vi "Beampointing_ajgEdit.vi"() -> ()   [LabVIEW 2020]
uses:
  Ctrs/beam detection.ctl
  GUI_Beampointing_single_TRA/Ctrs/move.ctl
  Shared/GUI_Template/GUI_master/tcp_new_data_event.ctl
  Shared/GUI_Template/GUI_master/tcp new data cluster.ctl
  Shared/MySQL/Preset Query Enum.ctl
  Ctrs/motor cfg.ctl
  Ctrs/BP configuration.ctl
  General GUIs/Device GUIs/GUI_Cameras/Controls/Crosshair type def.ctl
  <userlib>/_OpenG.lib/array/array.llb/Filter 1D Array with Scalar (String)__ogtk.vi
  <vilib>/Utility/file.llb/Read From Spreadsheet File (string).vi
  <userlib>/_OpenG.lib/array/array.llb/Index 1D Array Elements (String)__ogtk.vi
  <vilib>/Analysis/NI_AALBase.lvlib
  <vilib>/vision/NI_Vision_Development_Module.lvlib
  <vilib>/Utility/file.llb/Write To Spreadsheet File (string).vi
panel:
  in  "Position.Axis 3::99":dbl=77.0 caption="Motor Axis 1" min=0.0 max=20.0 format="%#_6f"
  out "tcp data event 2":T1
  out "error out 3":errorcluster
  out "Array 3":sgl[](array[numeric])
  in  "GUIdevice 97":string="BELLA_ESP_2"
  in  "GUIdevice 98":string="BellaESP"
  in  "Position.Axis 1::97":dbl=77.0 caption="Motor Axis 1" min=-10.0 max=10.0 format="%#_6f"
  in  "Position.Axis 2::97":dbl=77.0 caption="Motor Axis 1" min=-12.0 max=10.0 format="%#_6f"
  in  "Position.Axis 3::97":dbl=77.0 caption="Motor Axis 1" min=-12.0 max=12.0 format="%#_6f"
  in  "Position.Axis 1::98":dbl=77.0 caption="Motor Axis 1" min=0.0 max=20.0 format="%#_6f"
  in  "Position.Axis 2::98":dbl=77.0 caption="Motor Axis 1" min=0.0 max=20.0 format="%#_6f"
  in  "Position.Axis 3::98":dbl=77.0 caption="Motor Axis 1" min=0.0 max=20.0 format="%#_6f"
  in  "save path":path=path "W:/BP_DATA"
  out "size(s) 6":i32
  out "config path":string
  out "Moving Y":string
  out "Moving X":string
  out "particles":T2(array[cluster])
  out "millisecond timer value":u32
  out "appended path":path
  in  "active Axis ref 3":cluster{"Ref X":refnum<vi>, "Ref Y":refnum<vi>}
  out "motor refs 3":refnum<vi>[](array[refnum])
  in  "active man refs":cluster{"Ref X":refnum<vi>, "Ref Y":refnum<vi>}
  in  "Numeric":dbl
  out "Current State":string
  out "CCDs":string[](array[string])
  in  "GUIdevice 12":string
  in  "GUIdevice 11":string
  in  "GUIdevice 10":string
  in  "GUIdevice 9":string
  out "error out 2":errorcluster
  in  "active cams":string[](array[string])
  in  "Motor Y":dbl[][](array[numeric])
  in  "Motor X":dbl[][](array[numeric])
  out "Names":string[](array[string])
  in  "Offset X stats":dbl[][](array[numeric])
  in  "Offset Y stats":dbl[][](array[numeric])
  out "Box":T3(array[cluster])
  in  "Tab Cams":enum32{"Config ", "Main", "History"}(tab)=enum."Main"
  in  "associated motors Y":T4 {"Motor CCD 12" items=["F3M5 Horizontal", "F3M5 Vertical", "F3M6 Horizontal", "F3M3 Vertical", "F3M3 Horizontal", "F3M6 Vertical", "M4 X Axis", "M5 X Axis", "M5 Y Axis"]; "Motor CCD 11" items=["F3M5 Horizontal", "F3M5 Vertical", "F3M6 Horizontal", "F3M3 Vertical", "F3M3 Horizontal", "F3M6 Vertical", "M4 X Axis", "M5 X Axis", "M5 Y Axis"]; "Motor CCD 10" items=["F3M5 Horizontal", "F3M5 Vertical", "F3M6 Horizontal", "F3M3 Vertical", "F3M3 Horizontal", "F3M6 Vertical", "M4 X Axis", "M5 X Axis", "M5 Y Axis"]; "Motor CCD 9" items=["F3M5 Horizontal", "F3M5 Vertical", "F3M6 Horizontal", "F3M3 Vertical", "F3M3 Horizontal", "F3M6 Vertical", "M4 X Axis", "M5 X Axis", "M5 Y Axis"]; "Motor CCD 8" items=["F3M5 Horizontal", "F3M5 Vertical", "F3M6 Horizontal", "F3M3 Vertical", "F3M3 Horizontal", "F3M6 Vertical", "M4 X Axis", "M5 X Axis", "M5 Y Axis"]; "Motor CCD 7" items=["F3M5 Horizontal", "F3M5 Vertical", "F3M6 Horizontal", "F3M3 Vertical", "F3M3 Horizontal", "F3M6 Vertical", "M4 X Axis", "M5 X Axis", "M5 Y Axis"]; "Motor CCD 6" items=["F3M5 Horizontal", "F3M5 Vertical", "F3M6 Horizontal", "F3M3 Vertical", "F3M3 Horizontal", "F3M6 Vertical", "M4 X Axis", "M5 X Axis", "M5 Y Axis"]; "Motor CCD 5" items=["F3M5 Horizontal", "F3M5 Vertical", "F3M6 Horizontal", "F3M3 Vertical", "F3M3 Horizontal", "F3M6 Vertical", "M4 X Axis", "M5 X Axis", "M5 Y Axis"]; "Motor CCD 4" items=["F3M5 Horizontal", "F3M5 Vertical", "F3M6 Horizontal", "F3M3 Vertical", "F3M3 Horizontal", "F3M6 Vertical", "M4 X Axis", "M5 X Axis", "M5 Y Axis"]; "Motor CCD 3" items=["F3M5 Horizontal", "F3M5 Vertical", "F3M6 Horizontal", "F3M3 Vertical", "F3M3 Horizontal", "F3M6 Vertical", "M4 X Axis", "M5 X Axis", "M5 Y Axis"]; "Motor CCD 2" items=["F3M5 Horizontal", "F3M5 Vertical", "F3M6 Horizontal", "F3M3 Vertical", "F3M3 Horizontal", "F3M6 Vertical", "M4 X Axis", "M5 X Axis", "M5 Y Axis"]; "Motor CCD 1" items=["F3M5 Horizontal", "F3M5 Vertical", "F3M6 Horizontal", "F3M3 Vertical", "F3M3 Horizontal", "F3M6 Vertical", "M4 X Axis", "M5 X Axis", "M5 Y Axis"]}
  in  "associated motors X":T4 {"Motor CCD 12" items=["F3M5 Horizontal", "F3M5 Vertical", "F3M6 Horizontal", "F3M3 Vertical", "F3M3 Horizontal", "F3M6 Vertical", "M4 X Axis", "M5 X Axis", "M5 Y Axis"]; "Motor CCD 11" items=["F3M5 Horizontal", "F3M5 Vertical", "F3M6 Horizontal", "F3M3 Vertical", "F3M3 Horizontal", "F3M6 Vertical", "M4 X Axis", "M5 X Axis", "M5 Y Axis"]; "Motor CCD 10" items=["F3M5 Horizontal", "F3M5 Vertical", "F3M6 Horizontal", "F3M3 Vertical", "F3M3 Horizontal", "F3M6 Vertical", "M4 X Axis", "M5 X Axis", "M5 Y Axis"]; "Motor CCD 9" items=["F3M5 Horizontal", "F3M5 Vertical", "F3M6 Horizontal", "F3M3 Vertical", "F3M3 Horizontal", "F3M6 Vertical", "M4 X Axis", "M5 X Axis", "M5 Y Axis"]; "Motor CCD 8" items=["F3M5 Horizontal", "F3M5 Vertical", "F3M6 Horizontal", "F3M3 Vertical", "F3M3 Horizontal", "F3M6 Vertical", "M4 X Axis", "M5 X Axis", "M5 Y Axis"]; "Motor CCD 7" items=["F3M5 Horizontal", "F3M5 Vertical", "F3M6 Horizontal", "F3M3 Vertical", "F3M3 Horizontal", "F3M6 Vertical", "M4 X Axis", "M5 X Axis", "M5 Y Axis"]; "Motor CCD 6" items=["F3M5 Horizontal", "F3M5 Vertical", "F3M6 Horizontal", "F3M3 Vertical", "F3M3 Horizontal", "F3M6 Vertical", "M4 X Axis", "M5 X Axis", "M5 Y Axis"]; "Motor CCD 5" items=["F3M5 Horizontal", "F3M5 Vertical", "F3M6 Horizontal", "F3M3 Vertical", "F3M3 Horizontal", "F3M6 Vertical", "M4 X Axis", "M5 X Axis", "M5 Y Axis"]; "Motor CCD 4" items=["F3M5 Horizontal", "F3M5 Vertical", "F3M6 Horizontal", "F3M3 Vertical", "F3M3 Horizontal", "F3M6 Vertical", "M4 X Axis", "M5 X Axis", "M5 Y Axis"]; "Motor CCD 3" items=["F3M5 Horizontal", "F3M5 Vertical", "F3M6 Horizontal", "F3M3 Vertical", "F3M3 Horizontal", "F3M6 Vertical", "M4 X Axis", "M5 X Axis", "M5 Y Axis"]; "Motor CCD 2" items=["F3M5 Horizontal", "F3M5 Vertical", "F3M6 Horizontal", "F3M3 Vertical", "F3M3 Horizontal", "F3M6 Vertical", "M4 X Axis", "M5 X Axis", "M5 Y Axis"]; "Motor CCD 1" items=["F3M5 Horizontal", "F3M5 Vertical", "F3M6 Horizontal", "F3M3 Vertical", "F3M3 Horizontal", "F3M6 Vertical", "M4 X Axis", "M5 X Axis", "M5 Y Axis"]}
  out "Cameras":T5
  out "Status":cluster{i32, i32, "Centroid X":dbl[][]}(graph)
  in  "Exposure:12":dbl=0.095 min=0.0001 max=1.0 format="%#_6f"
  in  "Triggerdelay::12":dbl=0.003 min=0.0 max=0.09 format="%#_6f"
  in  "Exposure::11":dbl=0.095 min=0.0001 max=1.0 format="%#_6f"
  in  "Triggerdelay::11":dbl=0.003 min=0.0 max=0.09 format="%#_6f"
  in  "Exposure::10":dbl=0.095 min=0.0001 max=1.0 format="%#_6f"
  in  "Triggerdelay::10":dbl=0.003 min=0.0 max=0.09 format="%#_6f"
  in  "Exposure::9":dbl=0.095 min=0.0001 max=1.0 format="%#_6f"
  in  "Triggerdelay::9":dbl=0.003 min=0.0 max=0.09 format="%#_6f"
  in  "Trigger::9":bool
  in  "Trigger::10":bool caption="Trigger:10"
  in  "Trigger::11":bool
  in  "Trigger::12":bool
  in  "Target.Y::9":dbl=45.0 caption="T9y" min=0.0 max=2000.0 format="%#_6f"
  in  "Target.X::9":dbl=47.0 caption="Tx9" min=0.0 max=2000.0 format="%#_6f"
  in  "Target.Y::10":dbl=45.0 caption="T10y" min=0.0 max=2000.0 format="%#_6f"
  in  "Target.X::10":dbl=47.0 caption="T10x" min=0.0 max=2000.0 format="%#_6f"
  in  "Target.Y::11":dbl=45.0 caption="T11y" min=0.0 max=2000.0 format="%#_6f"
  in  "Target.X::11":dbl=47.0 caption="T11x" min=0.0 max=2000.0 format="%#_6f"
  in  "Target.Y::12":dbl=45.0 caption="T12y" min=0.0 max=2000.0 format="%#_6f"
  in  "Target.X::12":dbl=47.0 caption="T12x" min=0.0 max=2000.0 format="%#_6f"
  in  "Exposure::8":dbl=0.095 min=0.0001 max=1.0 format="%#_6f"
  in  "Triggerdelay::8":dbl=0.003 min=0.0 max=0.09 format="%#_6f"
  in  "Trigger::8":bool
  in  "Target.Y::8":dbl=45.0 caption="T8y" min=0.0 max=2000.0 format="%#_6f"
  in  "Target.X::8":dbl=47.0 caption="T8x" min=0.0 max=2000.0 format="%#_6f"
  in  "Target.Y::7":dbl=45.0 caption="T7x" min=0.0 max=2000.0 format="%#_6f"
  in  "Target.X::7":dbl=47.0 caption="T7y" min=0.0 max=2000.0 format="%#_6f"
  in  "Target.Y::6":dbl=45.0 caption="T6y" min=0.0 max=2000.0 format="%#_6f"
  in  "Target.X::6":dbl=47.0 caption="T6x" min=0.0 max=2000.0 format="%#_6f"
  in  "Target.Y::5":dbl=45.0 caption="T5y" min=0.0 max=2000.0 format="%#_6f"
  in  "Target.X::5":dbl=47.0 caption="T5x" min=0.0 max=2000.0 format="%#_6f"
  in  "Target.Y::4":dbl=45.0 caption="T4y" min=0.0 max=2000.0 format="%#_6f"
  in  "Target.X::4":dbl=47.0 caption="T4x" min=0.0 max=2000.0 format="%#_6f"
  in  "Target.Y::3":dbl=163.0 caption="T3y" min=0.0 max=2000.0 format="%#_6f"
  in  "Target.X::3":dbl=152.0 caption="T3x" min=0.0 max=2000.0 format="%#_6f"
  in  "Target.Y::2":dbl=74.0 caption="T2y" min=0.0 max=2000.0 format="%#_6f"
  in  "Target.X::2":dbl=75.0 caption="T2x" min=0.0 max=2000.0 format="%#_6f"
  in  "Target.Y::1":dbl=61.0 caption="T1y" min=0.0 max=2000.0 format="%#_6f"
  in  "Target.X::1":dbl=77.0 caption="T1x" min=0.0 max=2000.0 format="%#_6f"
  in  "Exposure::7":dbl=0.095 min=3.8e-05 max=1.0 format="%#_6f"
  in  "Triggerdelay::7":dbl=0.003 min=0.0 max=0.09 format="%#_6f"
  in  "Trigger::7":bool
  in  "Exposure::6":dbl=0.095 min=3.8e-05 max=1.0 format="%#_6f"
  in  "Triggerdelay::6":dbl=0.003 min=0.0 max=0.09 format="%#_6f"
  in  "Trigger::6":bool
  in  "Exposure::5":dbl=0.095 min=3.8e-05 max=1.0 format="%#_6f"
  in  "Triggerdelay::5":dbl=0.003 min=0.0 max=0.09 format="%#_6f"
  in  "Trigger::5":bool
  in  "Exposure::4":dbl=0.095 min=3.8e-05 max=1.0 format="%#_6f"
  in  "Triggerdelay::4":dbl=0.003 min=0.0 max=0.09 format="%#_6f"
  in  "Trigger::4":bool
  in  "Exposure::3":dbl=0.095 min=3.8e-05 max=1.0 format="%#_6f"
  in  "Triggerdelay::3":dbl=0.003 min=0.0 max=0.09 format="%#_6f"
  in  "Trigger::3":bool
  in  "Exposure::2":dbl=0.095 min=3.8e-05 max=1.0 format="%#_6f"
  in  "Triggerdelay::2":dbl=0.003 min=0.0 max=0.09 format="%#_6f"
  in  "Trigger::2":bool
  out "image::1":T6(plugin-control) caption="CAM-2BL-GHOST"
  out "image::2":T6(plugin-control) caption="CAM-2BL-F3M7"
  out "image::3":T6(plugin-control)
  out "image::4":T6(plugin-control)
  out "image::5":T6(plugin-control)
  out "image::6":T6(plugin-control)
  out "image::7":T6(plugin-control)
  out "image::8":T6(plugin-control)
  in  "Exposure::1":dbl=0.095 min=3.8e-05 max=1.0 format="%#_6f"
  in  "Triggerdelay::1":dbl=0.003 min=0.0 max=0.09 format="%#_6f"
  in  "Trigger::1":bool
  in  "UDP error message":string
  out "required Y":bool[](array[boolean])
  out "required X":bool[](array[boolean])
  out "detected":bool[](array[boolean])
  out "name array":string[](array[string])
  out "image::9":T6(plugin-control)
  out "image::10":T6(plugin-control)
  out "image::11":T6(plugin-control)
  out "image::12":T6(plugin-control)
  out "speedmode X":bool[](array[boolean])
  out "speedmode Y":bool[](array[boolean])
  out "CCD 9":cluster{timestamp[], dbl[]}[](graph)
  out "CCD 10":cluster{timestamp[], dbl[]}[](graph)
  out "CCD 11":cluster{timestamp[], dbl[]}[](graph)
  out "CCD 12":cluster{timestamp[], dbl[]}[](graph)
  out "CCD 5":cluster{timestamp[], dbl[]}[](graph)
  out "CCD 6":cluster{timestamp[], dbl[]}[](graph)
  out "CCD 7":cluster{timestamp[], dbl[]}[](graph)
  out "CCD 8":cluster{timestamp[], dbl[]}[](graph)
  out "CCD 2":cluster{timestamp[], dbl[]}[](graph)
  out "CCD 1":cluster{timestamp[], dbl[]}[](graph)
  out "CCD 3":cluster{timestamp[], dbl[]}[](graph)
  out "CCD 4":cluster{timestamp[], dbl[]}[](graph)
  in  "History Size":i32=500
  out "History Index":i32
  in  "Feedback Global":bool
  in  "detection para":T7[](array[typedef])=[{"Filter"=1, "Filter Para"={"X Size"=5, "Y Size"=5, "% Tolerance"=1}, "detection method"=4, "smal para"=[{"Measurement Parameter"=35, "Range Lower Value"=0.0, "Range Upper Value"=0.0, "Range"=TRUE, "Measurement Type"=FALSE}], "Remove small Objects"=TRUE, "Restrict to round Objects"=FALSE}, {"Filter"=1, "Filter Para"={"X Size"=5, "Y Size"=5, "% Tolerance"=1}, "detection method"=4, "smal para"=[{"Measurement Parameter"=35, "Range Lower Value"=0.0, "Range Upper Value"=500.0, "Range"=FALSE, "Measurement Type"=FALSE}], "Remove small Objects"=TRUE, "Restrict to round Objects"=FALSE}, {"Filter"=1, "Filter Para"={"X Size"=5, "Y Size"=5, "% Tolerance"=1}, "detection method"=4, "smal para"=[{"Measurement Parameter"=35, "Range Lower Value"=0.0, "Range Upper Value"=500.0, "Range"=TRUE, "Measurement Type"=FALSE}], "Remove small Objects"=TRUE, "Restrict to round Objects"=FALSE}, {"Filter"=1, "Filter Para"={"X Size"=5, "Y Size"=5, "% Tolerance"=1}, "detection method"=4, "smal para"=[{"Measurement Parameter"=35, "Range Lower Value"=0.0, "Range Upper Value"=500.0, "Range"=TRUE, "Measurement Type"=FALSE}], "Remove small Objects"=TRUE, "Restrict to round Objects"=FALSE}, {"Filter"=1, "Filter Para"={"X Size"=5, "Y Size"=5, "% Tolerance"=1}, "detection method"=4, "smal para"=[{"Measurement Parameter"=35, "Range Lower Value"=0.0, "Range Upper Value"=500.0, "Range"=TRUE, "Measurement Type"=FALSE}], "Remove small Objects"=TRUE, "Restrict to round Objects"=FALSE}, {"Filter"=1, "Filter Para"={"X Size"=5, "Y Size"=5, "% Tolerance"=1}, "detection method"=4, "smal para"=[{"Measurement Parameter"=35, "Range Lower Value"=0.0, "Range Upper Value"=500.0, "Range"=TRUE, "Measurement Type"=FALSE}], "Remove small Objects"=TRUE, "Restrict to round Objects"=FALSE}, {"Filter"=1, "Filter Para"={"X Size"=5, "Y Size"=5, "% Tolerance"=1}, "detection method"=4, "smal para"=[{"Measurement Parameter"=35, "Range Lower Value"=0.0, "Range Upper Value"=500.0, "Range"=TRUE, "Measurement Type"=FALSE}], "Remove small Objects"=TRUE, "Restrict to round Objects"=FALSE}, {"Filter"=1, "Filter Para"={"X Size"=5, "Y Size"=5, "% Tolerance"=1}, "detection method"=3, "smal para"=[{"Measurement Parameter"=35, "Range Lower Value"=0.0, "Range Upper Value"=0.0, "Range"=FALSE, "Measurement Type"=FALSE}], "Remove small Objects"=TRUE, "Restrict to round Objects"=FALSE}, {"Filter"=1, "Filter Para"={"X Size"=5, "Y Size"=5, "% Tolerance"=1}, "detection method"=4, "smal para"=[{"Measurement Parameter"=35, "Range Lower Value"=0.0, "Range Upper Value"=0.0, "Range"=FALSE, "Measurement Type"=FALSE}], "Remove small Objects"=TRUE, "Restrict to round Objects"=FALSE}, {"Filter"=1, "Filter Para"={"X Size"=5, "Y Size"=5, "% Tolerance"=1}, "detection method"=4, "smal para"=[{"Measurement Parameter"=35, "Range Lower Value"=0.0, "Range Upper Value"=500.0, "Range"=TRUE, "Measurement Type"=FALSE}], "Remove small Objects"=TRUE, "Restrict to round Objects"=FALSE}, {"Filter"=1, "Filter Para"={"X Size"=5, "Y Size"=5, "% Tolerance"=1}, "detection method"=4, "smal para"=[{"Measurement Parameter"=35, "Range Lower Value"=0.0, "Range Upper Value"=500.0, "Range"=TRUE, "Measurement Type"=FALSE}], "Remove small Objects"=TRUE, "Restrict to round Objects"=FALSE}, {"Filter"=1, "Filter Para"={"X Size"=5, "Y Size"=5, "% Tolerance"=1}, "detection method"=4, "smal para"=[{"Measurement Parameter"=35, "Range Lower Value"=0.0, "Range Upper Value"=500.0, "Range"=TRUE, "Measurement Type"=FALSE}], "Remove small Objects"=TRUE, "Restrict to round Objects"=FALSE}] {"smal para"."Measurement Parameter" items=["Center of Mass X", "Center of Mass Y", "First Pixel X", "First Pixel Y", "Bounding Rect Left", "Bounding Rect Top", "Bounding Rect Right", "Bounding Rect Bottom", "Max Feret Diameter Start X", "Max Feret Diameter Start Y", "Max Feret Diameter End X", "Max Feret Diameter End Y", "Max Horiz. Segment Length Left", "Max Horiz. Segment Length Right", "Max Horiz. Segment Length Row", "-", "Bounding Rect Width", "Bounding Rect Height", "Bounding Rect Diagonal", "Perimeter", "Convex Hull Perimeter", "Holes' Perimeter", "Max Feret Diameter", "Equivalent Ellipse Major Axis", "Equivalent Ellipse Minor Axis", "Equivalent Ellipse Minor Axis (Feret)", "Equivalent Rect Long Side", "Equivalent Rect Short Side", "Equivalent Rect Diagonal", "Equivalent Rect Short Side (Feret)", "Average Horiz. Segment Length", "Average Vert. Segment Length", "Hydraulic Radius", "Waddel Disk Diameter", "-", "Area", "Holes' Area", "Particle & Holes' Area", "Convex Hull Area", "Image Area", "-", "Number of Holes", "Number of Horiz. Segments", "Number of Vert. Segments", "-", "Orientation", "Max Feret Diameter Orientation", "-", "% Area/Image Area", "% Area/(Particle & Holes' Area)", "Ratio of Equivalent Ellipse Axes", "Ratio of Equivalent Rect Sides", "-", "Elongation Factor", "Compactness Factor", "Heywood Circularity Factor", "Type Factor", "-", "Sum X", "Sum Y", "Sum XX", "Sum XY", "Sum YY", "Sum XXX", "Sum XXY", "Sum XYY", "Sum YYY", "-", "Moment of Inertia XX", "Moment of Inertia XY", "Moment of Inertia YY", "Moment of Inertia XXX", "Moment of Inertia XXY", "Moment of Inertia XYY", "Moment of Inertia YYY", "Norm. Moment of Inertia XX", "Norm. Moment of Inertia XY", "Norm. Moment of Inertia YY", "Norm. Moment of Inertia XXX", "Norm. Moment of Inertia XXY", "Norm. Moment of Inertia XYY", "Norm. Moment of Inertia YYY", "Hu Moment 1", "Hu Moment 2", "Hu Moment 3", "Hu Moment 4", "Hu Moment 5", "Hu Moment 6", "Hu Moment 7"]; "smal para"."Range Lower Value" format="%.2f"; "smal para"."Range Upper Value" format="%.2f"; "detection method" items=["clustering", "entropy", "metric", "moments", "inter-class variance"]; "Filter" items=["No Filter", "Median Filter", "Low Pass Filter"]}
  in  "GUIdevice 8":string
  in  "Tab Control":T9(tab)
  in  "alarms":bool
  in  "new tdms":bool
  in  "Save Stats":bool
  in  "Save Config":bool
  in  "Load Config":bool
  in  "update speed [ms]":i32=2000
  in  "img to avg":i32=6 min=3 max=200
  in  "Reset History":bool
  in  "autodetect":bool
  in  "Detection Rate":dbl=0.9 min=0.001 max=1.0
  in  "Center":bool
  in  "Align":bool
  in  "Speedmode":dbl=5.0 min=1.0 max=20.0
  in  "device ini":bool
  in  "average centroid":bool
  in  "beam detection para":T7={"Filter"=1, "Filter Para"={"X Size"=5, "Y Size"=5, "% Tolerance"=1}, "detection method"=4, "smal para"=[{"Measurement Parameter"=35, "Range Lower Value"=0.0, "Range Upper Value"=500.0, "Range"=FALSE, "Measurement Type"=FALSE}], "Remove small Objects"=TRUE, "Restrict to round Objects"=FALSE} {"smal para"."Measurement Parameter" items=["Center of Mass X", "Center of Mass Y", "First Pixel X", "First Pixel Y", "Bounding Rect Left", "Bounding Rect Top", "Bounding Rect Right", "Bounding Rect Bottom", "Max Feret Diameter Start X", "Max Feret Diameter Start Y", "Max Feret Diameter End X", "Max Feret Diameter End Y", "Max Horiz. Segment Length Left", "Max Horiz. Segment Length Right", "Max Horiz. Segment Length Row", "-", "Bounding Rect Width", "Bounding Rect Height", "Bounding Rect Diagonal", "Perimeter", "Convex Hull Perimeter", "Holes' Perimeter", "Max Feret Diameter", "Equivalent Ellipse Major Axis", "Equivalent Ellipse Minor Axis", "Equivalent Ellipse Minor Axis (Feret)", "Equivalent Rect Long Side", "Equivalent Rect Short Side", "Equivalent Rect Diagonal", "Equivalent Rect Short Side (Feret)", "Average Horiz. Segment Length", "Average Vert. Segment Length", "Hydraulic Radius", "Waddel Disk Diameter", "-", "Area", "Holes' Area", "Particle & Holes' Area", "Convex Hull Area", "Image Area", "-", "Number of Holes", "Number of Horiz. Segments", "Number of Vert. Segments", "-", "Orientation", "Max Feret Diameter Orientation", "-", "% Area/Image Area", "% Area/(Particle & Holes' Area)", "Ratio of Equivalent Ellipse Axes", "Ratio of Equivalent Rect Sides", "-", "Elongation Factor", "Compactness Factor", "Heywood Circularity Factor", "Type Factor", "-", "Sum X", "Sum Y", "Sum XX", "Sum XY", "Sum YY", "Sum XXX", "Sum XXY", "Sum XYY", "Sum YYY", "-", "Moment of Inertia XX", "Moment of Inertia XY", "Moment of Inertia YY", "Moment of Inertia XXX", "Moment of Inertia XXY", "Moment of Inertia XYY", "Moment of Inertia YYY", "Norm. Moment of Inertia XX", "Norm. Moment of Inertia XY", "Norm. Moment of Inertia YY", "Norm. Moment of Inertia XXX", "Norm. Moment of Inertia XXY", "Norm. Moment of Inertia XYY", "Norm. Moment of Inertia YYY", "Hu Moment 1", "Hu Moment 2", "Hu Moment 3", "Hu Moment 4", "Hu Moment 5", "Hu Moment 6", "Hu Moment 7"]; "smal para"."Range Lower Value" format="%.2f"; "smal para"."Range Upper Value" format="%.2f"; "detection method" items=["clustering", "entropy", "metric", "moments", "inter-class variance"]; "Filter" items=["No Filter", "Median Filter", "Low Pass Filter"]}
  in  "move config":T10={"Tolerance [%]"=0.1, "Stepsize"=0.0001, "Invert Axis"=TRUE, "Invert Direction X"=FALSE, "Invert Direction Y"=TRUE, "enable feedback"=FALSE, "Set Centriod Target"=FALSE}
  in  "Position 2":dbl=0.001 caption="Stepsize" min=0.0 max=999999.0 format="%_6f"
  in  "Position 1":dbl=0.001 caption="Stepsize" min=0.0 max=999999.0 format="%_6f"
  in  "Right":bool caption="RelativeMove.Axis 1.CCW::1"
  in  "Left":bool caption="RelativeMove.Axis 1.CW::1"
  in  "Down":bool caption="RelativeMove.Axis. 2.CCW::1"
  in  "Up":bool caption="RelativeMove.Axis 2.CW::1"
  in  "StepSize":dbl=1.0 caption="Stepsize" min=0.0 max=1.0 step=0.001 format="%#_6p"
  in  "active axis refs 2":T11(array[cluster])
  in  "CCDs":u16(ring) items=["CAM-2BL-GHOST", "CAM-2BL-F3M7", "", "", "", "", "", "", "", "", "", ""]
  out "motor refs":refnum<vi>[](array[refnum])
  in  "Position.Axis 2::99":dbl=77.0 caption="Motor Axis 1" min=0.0 max=20.0 format="%#_6f"
  in  "Position.Axis 1::99":dbl=77.0 caption="Motor Axis 1" min=0.0 max=20.0 format="%#_6f"
  in  "GUIdevice 99":string="BELLA_ESP_M1"
  in  "move properties":T10[](array[typedef])=[{"Tolerance [%]"=0.1, "Stepsize"=0.0001, "Invert Axis"=TRUE, "Invert Direction X"=FALSE, "Invert Direction Y"=TRUE, "enable feedback"=FALSE, "Set Centriod Target"=FALSE}, {"Tolerance [%]"=0.1, "Stepsize"=0.0001, "Invert Axis"=TRUE, "Invert Direction X"=FALSE, "Invert Direction Y"=TRUE, "enable feedback"=FALSE, "Set Centriod Target"=FALSE}, {"Tolerance [%]"=0.1, "Stepsize"=0.0001, "Invert Axis"=TRUE, "Invert Direction X"=FALSE, "Invert Direction Y"=TRUE, "enable feedback"=FALSE, "Set Centriod Target"=FALSE}, {"Tolerance [%]"=0.1, "Stepsize"=0.0001, "Invert Axis"=TRUE, "Invert Direction X"=FALSE, "Invert Direction Y"=TRUE, "enable feedback"=FALSE, "Set Centriod Target"=FALSE}, {"Tolerance [%]"=0.1, "Stepsize"=0.0001, "Invert Axis"=TRUE, "Invert Direction X"=FALSE, "Invert Direction Y"=TRUE, "enable feedback"=FALSE, "Set Centriod Target"=FALSE}, {"Tolerance [%]"=0.1, "Stepsize"=0.0001, "Invert Axis"=TRUE, "Invert Direction X"=FALSE, "Invert Direction Y"=TRUE, "enable feedback"=FALSE, "Set Centriod Target"=FALSE}, {"Tolerance [%]"=0.1, "Stepsize"=0.0001, "Invert Axis"=TRUE, "Invert Direction X"=FALSE, "Invert Direction Y"=TRUE, "enable feedback"=FALSE, "Set Centriod Target"=FALSE}, {"Tolerance [%]"=0.1, "Stepsize"=0.0001, "Invert Axis"=TRUE, "Invert Direction X"=FALSE, "Invert Direction Y"=TRUE, "enable feedback"=FALSE, "Set Centriod Target"=FALSE}, {"Tolerance [%]"=0.1, "Stepsize"=0.0001, "Invert Axis"=TRUE, "Invert Direction X"=FALSE, "Invert Direction Y"=TRUE, "enable feedback"=FALSE, "Set Centriod Target"=FALSE}, {"Tolerance [%]"=0.1, "Stepsize"=0.0001, "Invert Axis"=TRUE, "Invert Direction X"=FALSE, "Invert Direction Y"=TRUE, "enable feedback"=FALSE, "Set Centriod Target"=FALSE}, {"Tolerance [%]"=0.1, "Stepsize"=0.0001, "Invert Axis"=TRUE, "Invert Direction X"=FALSE, "Invert Direction Y"=TRUE, "enable feedback"=FALSE, "Set Centriod Target"=FALSE}, {"Tolerance [%]"=0.1, "Stepsize"=0.0001, "Invert Axis"=TRUE, "Invert Direction X"=FALSE, "Invert Direction Y"=TRUE, "enable feedback"=FALSE, "Set Centriod Target"=FALSE}, {"Tolerance [%]"=0.1, "Stepsize"=0.0001, "Invert Axis"=TRUE, "Invert Direction X"=FALSE, "Invert Direction Y"=TRUE, "enable feedback"=FALSE, "Set Centriod Target"=FALSE}]
  in  "Time":timestamp[][](array[timestamp])
  in  "Mean Size":dbl[][](array[numeric])
  in  "Size":dbl[][](array[numeric])
  in  "active CCDs":i32(listbox)
  in  "Offset Y":dbl[][](array[numeric])
  in  "Offset X":dbl[][](array[numeric])
  in  "Mean Centroid X":dbl[][](array[numeric])
  in  "Mean Centroid Y":dbl[][](array[numeric])
  in  "Centroid Y":dbl[][](array[numeric])
  in  "Centroid X":dbl[][](array[numeric])
  in  "GUIdevice 7":string
  in  "GUIdevice 6":string
  in  "GUIdevice 5":string
  in  "GUIdevice 4":string
  in  "GUIdevice 3":string="TargetCam10Hz_Diode"
  in  "GUIdevice 2":string="StagingM1Far"
  in  "insert tag":bool=TRUE
  in  "stop":bool
  in  "GUIdevice 1":string="StagingM1Near"
  out "error IO 2":errorcluster
  # "Motor axes must have aliases"
  # "max"
  # "invert axis no longer used"
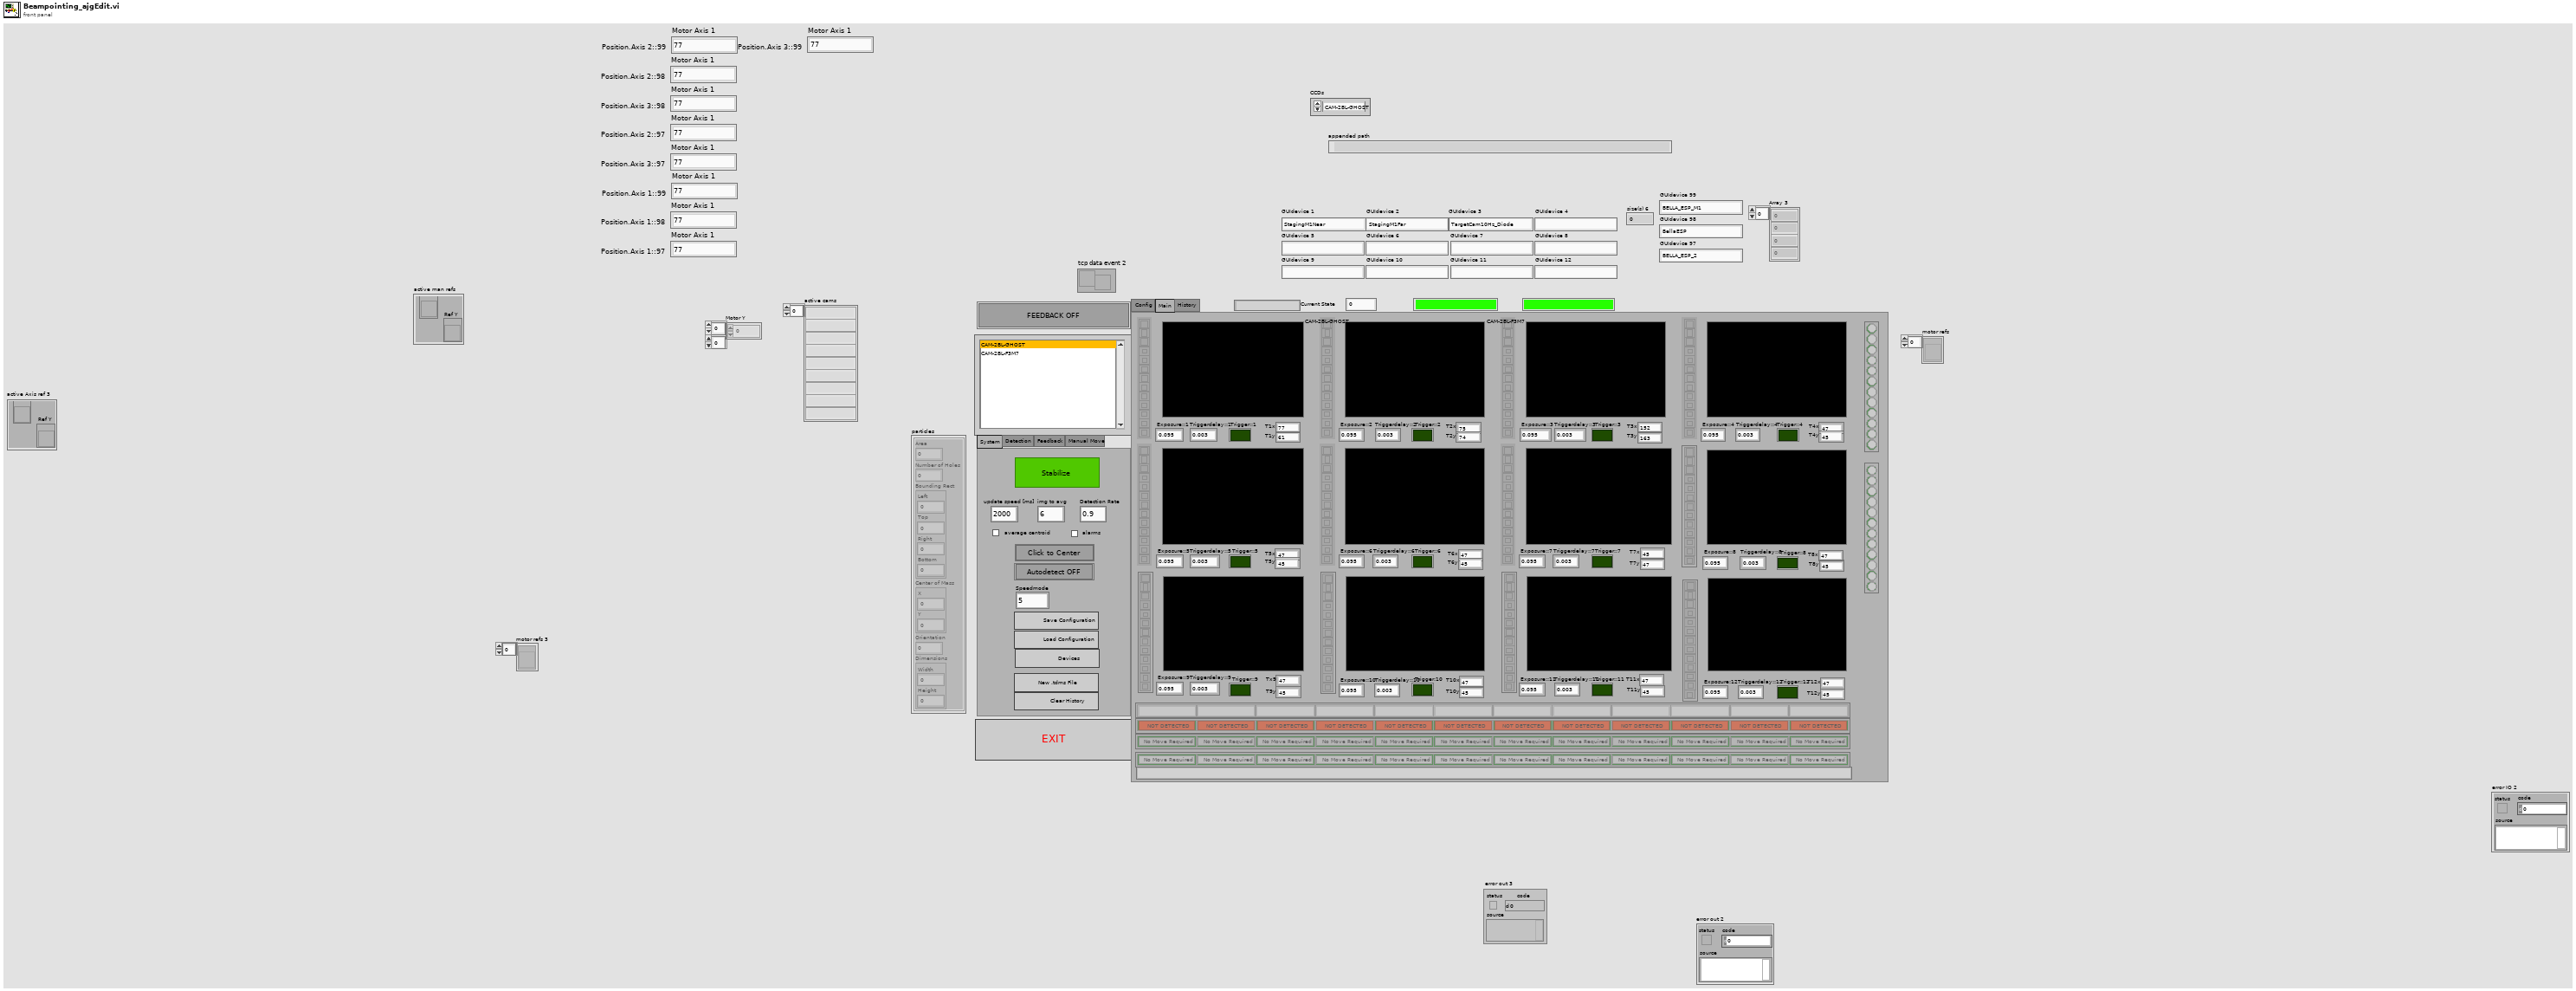
[diagram p1: front panel]
types:
  T1 = typedef "tcp_new_data_event.ctl" = refnum<user-event>
  T2 = cluster{"Area":dbl, "Number of Holes":dbl, "Bounding Rect":cluster{"Left":dbl, "Top":dbl, "Right":dbl, "Bottom":dbl}, "Center of Mass":cluster{"X":dbl, "Y":dbl}, "Orientation":dbl, "Dimensions":cluster{"Width":dbl, "Height":dbl}}[]
  T3 = cluster{"Left":dbl, "Top":dbl, "Right":dbl, "Bottom":dbl}[]
  T4 = cluster{"Motor CCD 1":u16, "Motor CCD 2":u16, "Motor CCD 3":u16, "Motor CCD 4":u16, "Motor CCD 5":u16, "Motor CCD 6":u16, "Motor CCD 7":u16, "Motor CCD 8":u16, "Motor CCD 9":u16, "Motor CCD 10":u16, "Motor CCD 11":u16, "Motor CCD 12":u16}
  T5 = cluster{"[0]":string, "[1]":string, "[2]":string, "[3]":string, "[4]":string, "[5]":string, "[6]":string, "[7]":string, "[8]":string, "[8] 2":string, "[8] 3":string, "[8] 4":string}
  T6 = typedef "IMAQ Image.ctl" = refnum<image>
  T7 = typedef "beam detection.ctl" = cluster{"Filter":u16, "Filter Para":cluster{"X Size":i32, "Y Size":i32, "% Tolerance":i32}, "detection method":i32, "smal para":cluster{"Measurement Parameter":T8, "Range Lower Value":dbl, "Range Upper Value":dbl, "Range":bool, "Measurement Type":bool}[], "Remove small Objects":bool, "Restrict to round Objects":bool}
  T8 = typedef "Particle Parameters" = i32
  T9 = enum32{"System", "Detection", "Feedback", "Manual Move"}
  T10 = typedef "move.ctl" = cluster{"Tolerance [%]":dbl, "Stepsize":dbl, "Invert Axis":bool, "Invert Direction X":bool, "Invert Direction Y":bool, "enable feedback":bool, "Set Centriod Target":bool}
  T11 = cluster{"Ref X":refnum<vi>, "Ref Y":refnum<vi>}[]
  T12 = cluster{"Target.X::1":refnum<vi>, "Target.Y::1":refnum<vi>}
  T13 = cluster{"Target.X::2":refnum<vi>, "Target.Y::2":refnum<vi>}
  T14 = cluster{"Target.X::3":refnum<vi>, "Target.Y::3":refnum<vi>}
  T15 = cluster{"Target.X::4":refnum<vi>, "Target.Y::4":refnum<vi>}
  T16 = cluster{"Target.X::5":refnum<vi>, "Target.Y::5":refnum<vi>}
  T17 = cluster{"Target.X::6":refnum<vi>, "Target.Y::6":refnum<vi>}
  T18 = cluster{"Target.X::7":refnum<vi>, "Target.Y::7":refnum<vi>}
  T19 = cluster{"Target.X::8":refnum<vi>, "Target.Y::8":refnum<vi>}
  T20 = cluster{"Target.X::12":refnum<vi>, "Target.Y::12":refnum<vi>}
  T21 = cluster{"Target.X::9":refnum<vi>, "Target.Y::9":refnum<vi>}
  T22 = cluster{"Target.X::10":refnum<vi>, "Target.Y::10":refnum<vi>}
  T23 = cluster{"Target.X::11":refnum<vi>, "Target.Y::11":refnum<vi>}
  T24 = cluster{"Target.X::12":refnum<vi>, "Target.Y::12":refnum<vi>}[]
  T25 = enum32{"invalid app kind", "Development System", "Run Time System", "Student Edition", "Embedded LabVIEW", "Evaluation", "Custom"}
  T26 = enum16{"open", "open or create", "create or replace", "create", "open (read-only)"}
  T27 = enum32{"Invalid", "Standard", "Closed", "Hidden", "Minimized", "Maximized"}
  T28 = typedef "Preset Query Enum.ctl" = enum16{"Get Locations", "Get all IPs and MACs", "Get classes", "Get expt variables to set at scanstart for particular device", "Get expt devices and variables with start values", "Get expt devices and variables (with data to get)", "Get expt devices with data to get", "Get Expt devices and GUIs", "Get all devices basic properties", "Get Virtual Devices Core Info", "Get Expt names", "Get experiment basic properties", "Get experiment alarm variables", "Get MC Ports", "Get device network comm port", "Get devicetype lvclass path", "Get basic device properties", "Get Init Order", "Get all setable variables of a device", "Get device variable aliases", "Get force values of all settable variables", "Get all variables of a devicetype", "Get all variables of a device", "Get plotter details", "Get Saved Scans", "Get Scan Info", "GetGeneralGUIs", "Get expt for plotter", "Get plotter IDs from expt", "Get all devices", "Get all Virtual Devices", "Get all aliases", "Get variable and device info for Virtual Device", "GetItemLocatorIP", "Get IPs for GUIs", "Get DeviceType from Device", "GetLocalPortRange", "GetDevicePresetVariables", "Get Device Configuration", "GetAllPresetNames", "GetAllConfigurationNames", "GetPresetDeviceNames"}
  T29 = typedef "tcp new data cluster.ctl" = cluster{"EventEnum":enum16{"new data", "connection status update"}, "Device name":string}
  T30 = typedef "motor cfg.ctl" = cluster{"CCDs":string[], "move properties":T10[], "detection para":T7[], "thresholds":cluster{"Lower value":sgl, "Upper value":sgl}[], "Motors X":cluster{"Motor CCD 1":u16, "Motor CCD 2":u16, "Motor CCD 3":u16, "Motor CCD 4":u16, "Motor CCD 5":u16, "Motor CCD 6":u16, "Motor CCD 7":u16, "Motor CCD 8":u16, "Motor CCD 9":u16, "Motor CCD 10":u16, "Motor CCD 11":u16, "Motor CCD 12":u16}, "Motors Y":cluster{"Motor CCD 1":u16, "Motor CCD 2":u16, "Motor CCD 3":u16, "Motor CCD 4":u16, "Motor CCD 5":u16, "Motor CCD 6":u16, "Motor CCD 7":u16, "Motor CCD 8":u16, "Motor CCD 9":u16, "Motor CCD 10":u16, "Motor CCD 11":u16, "Motor CCD 12":u16}}
  T31 = enum16{"open", "replace", "create", "open or create", "replace or create", "replace or create with confirmation"}
  T32 = enum8{"Enabled", "Disabled", "Disabled and Grayed Out"}
  T33 = cluster{"Left":dbl, "Top":dbl, "Right":dbl, "Bottom":dbl}
  T34 = cluster{"Core":cluster{"Current VI Reference":refnum<vi>, "Close Panel on Exit?":bool}, "detection para":T7[], "thresholds":cluster{"Lower value":sgl, "Upper value":sgl}[], "Centroid X":dbl[][], "Centroid Y":dbl[][], "img to avg":i32, "Mean Centroid X":dbl[][], "Mean Centroid Y":dbl[][], "Offset X":dbl[][], "Offset Y":dbl[][], "Offset X stats ":dbl[][], "Offset Y stats ":dbl[][], "Size":dbl[][], "Mean Size":dbl[][], "Time":timestamp[][], "move properties":T10[], "active axis refs 2":cluster{"Ref X":refnum<vi>, "Ref Y":refnum<vi>}[], "active ccd":i32, "Feedback global":bool, "Motor X":dbl[][], "Motor Y":dbl[][], "active cams":string[], "Data Value Reference out":refnum<k34>, "active man refs":cluster{"Ref X":refnum<vi>, "Ref Y":refnum<vi>}, "detected":bool[], "speedmode X":bool[], "speedmode Y":bool[], "steps speed X":dbl[], "steps speed Y":dbl[], "Supergui":cluster{"STOP queue":refnum<queue>, "SuperGUI ref":refnum<vi>}}
  T35 = cluster{"STOP queue":refnum<queue>, "SuperGUI ref":refnum<vi>}
  T36 = cluster{"Current VI Reference":refnum<vi>, "Close Panel on Exit?":bool}
  T37 = typedef "Image Type" = u32
  T38 = cluster{"[0]":string, "[1]":string, "[2]":string, "[3]":string, "[4]":string, "[5]":string, "[6]":string, "[7]":string, "[8]":string, "[9]":string, "[10]":string, "[11]":string}
  T39 = typedef "BP configuration.ctl" = cluster{"Camera names":string[], "Motor aliases x":string[], "Motor aliases y":string[], "detection para":T7[], "thresholds":cluster{"Lower value":sgl, "Upper value":sgl}[], "move properties":T10[]}
  T40 = cluster{"appended array":timestamp[], "appended array":dbl[]}
  T41 = cluster{"appended array":timestamp[], "appended array":dbl[]}[]
  T42 = typedef "Crosshair type def.ctl" = cluster{"Draw":bool, "Target":cluster{"x":dbl, "y":dbl}, "Size":cluster{"x":dbl, "y":dbl}, "Angle":dbl, "Color":u32, "Thickness":u8, "CrosshairLabel":string}
  T43 = cluster{"Left":i32, "Top":i32, "Right":i32, "Bottom":i32}
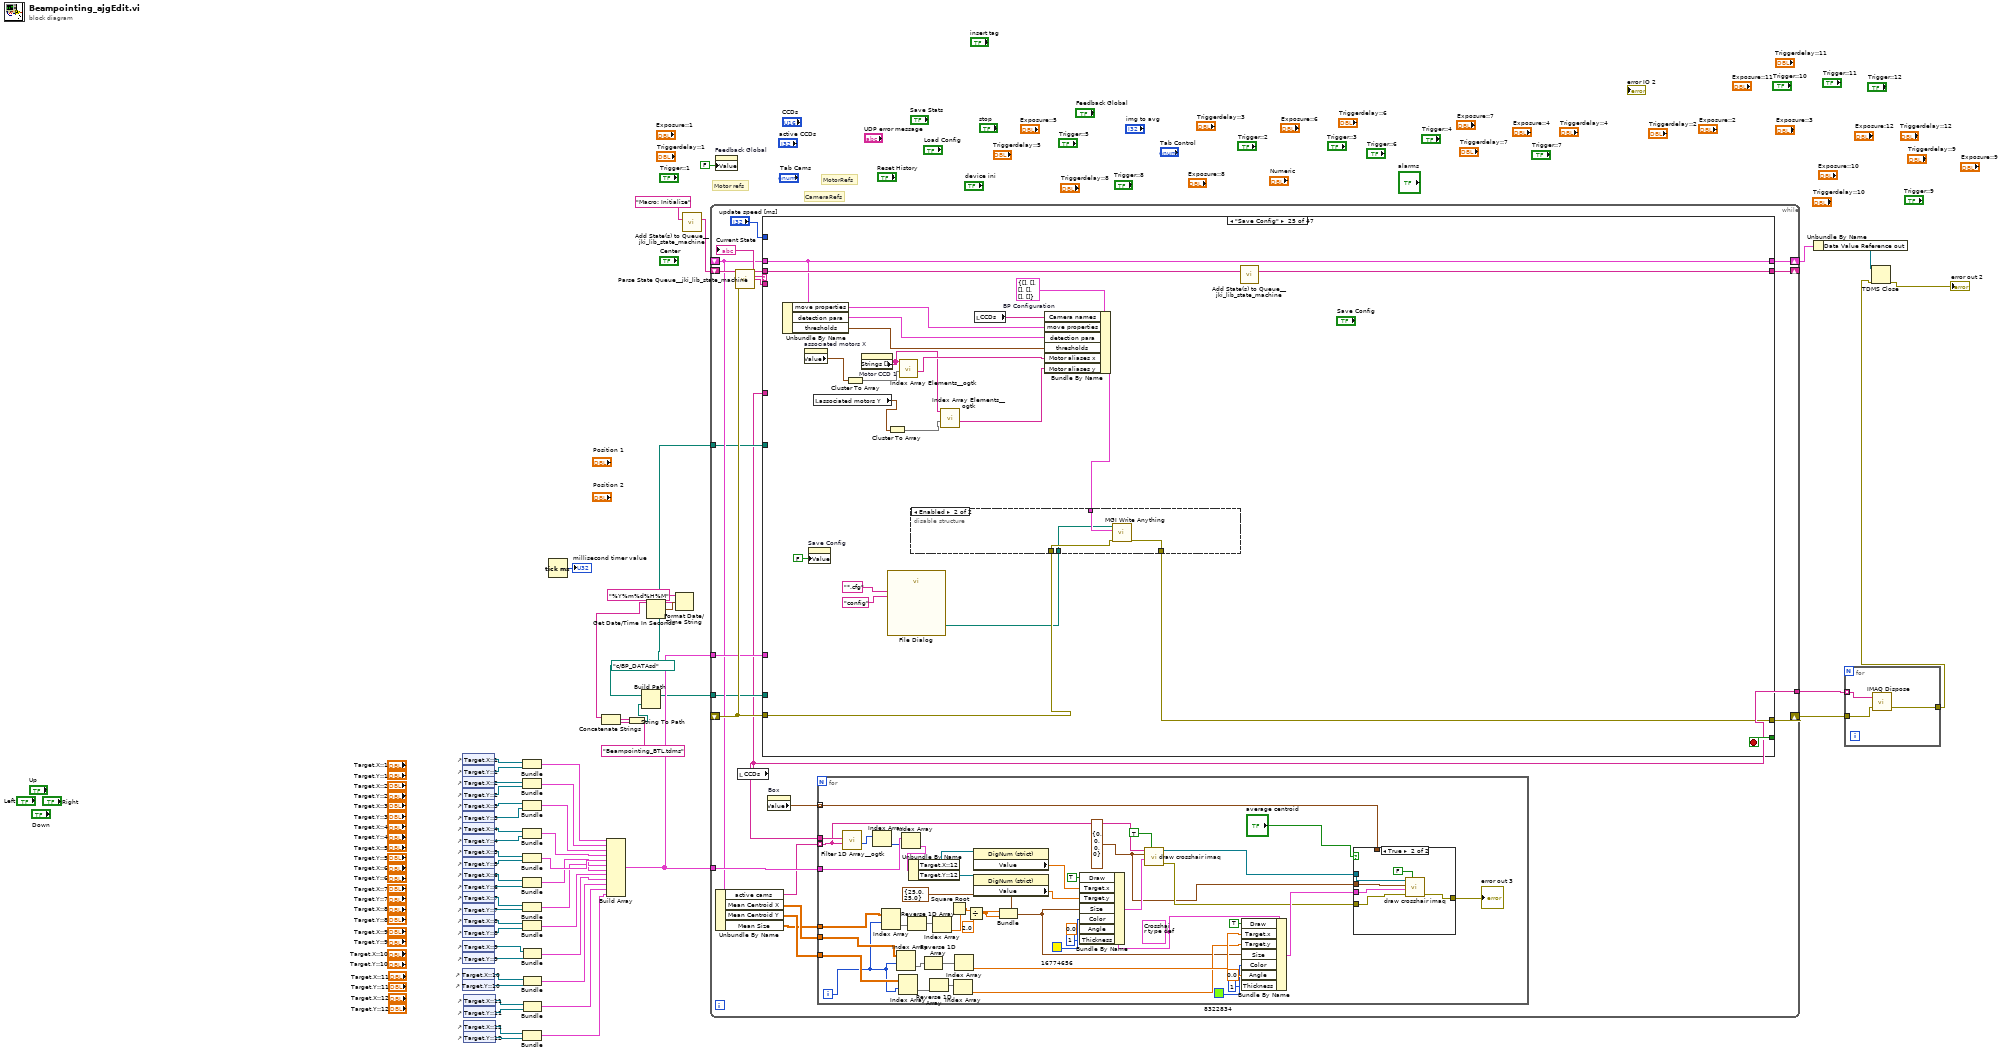
[diagram p0: block diagram]
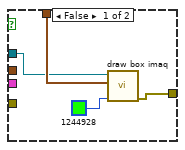
[diagram p2: hidden frame]
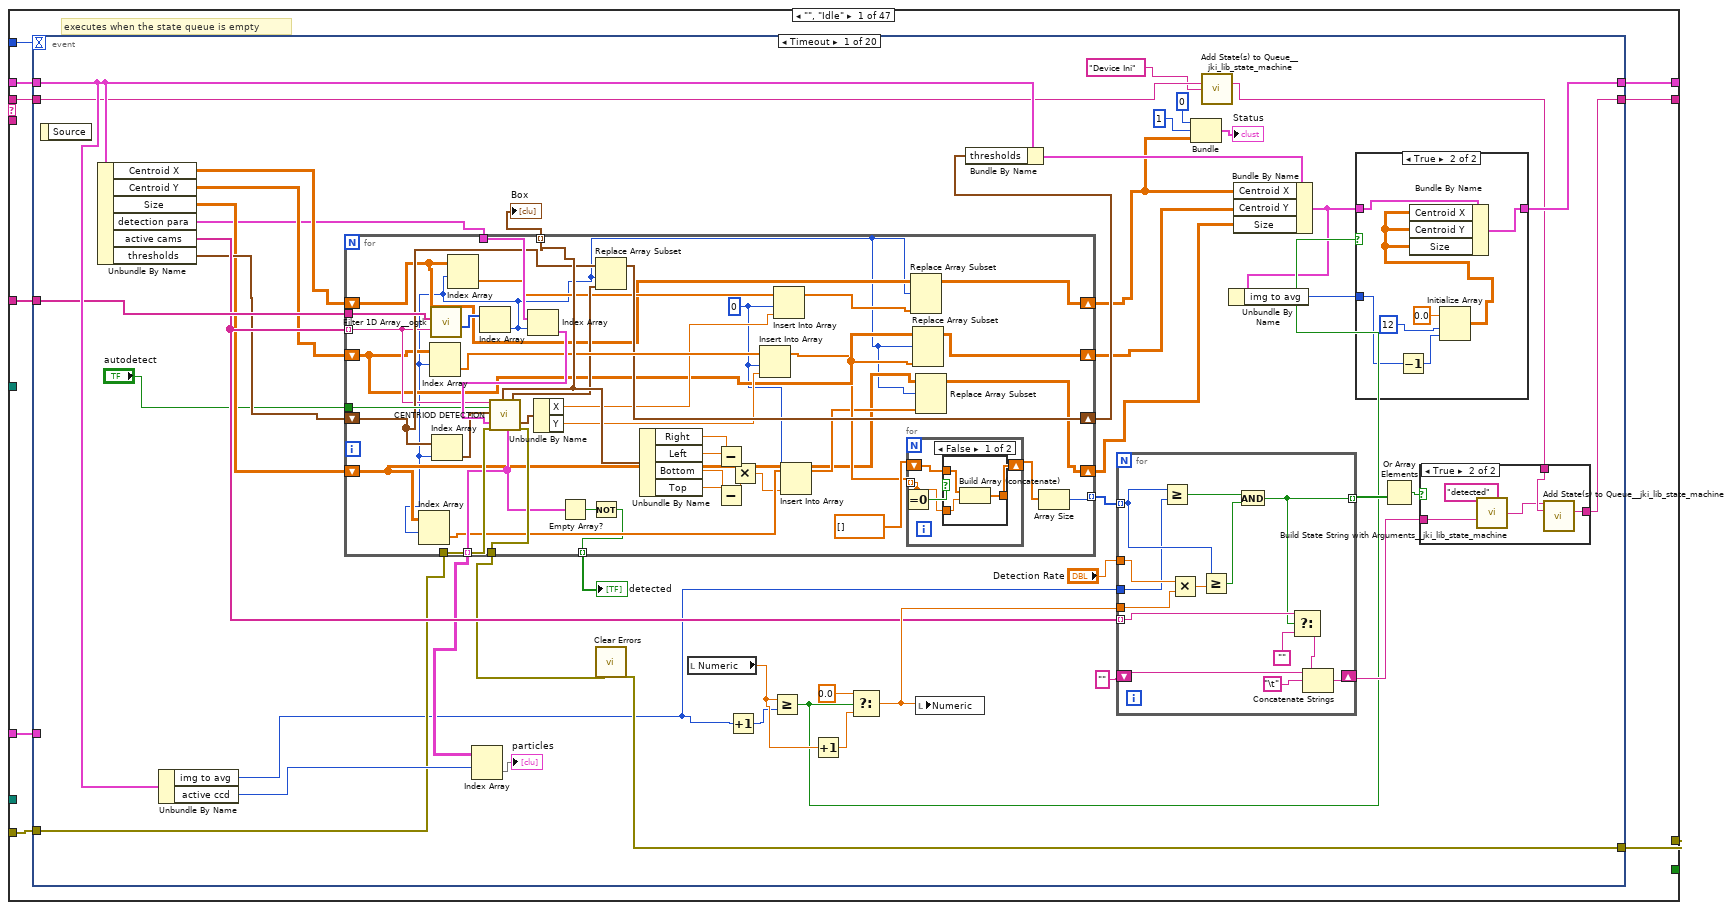
[diagram p3: hidden frame]
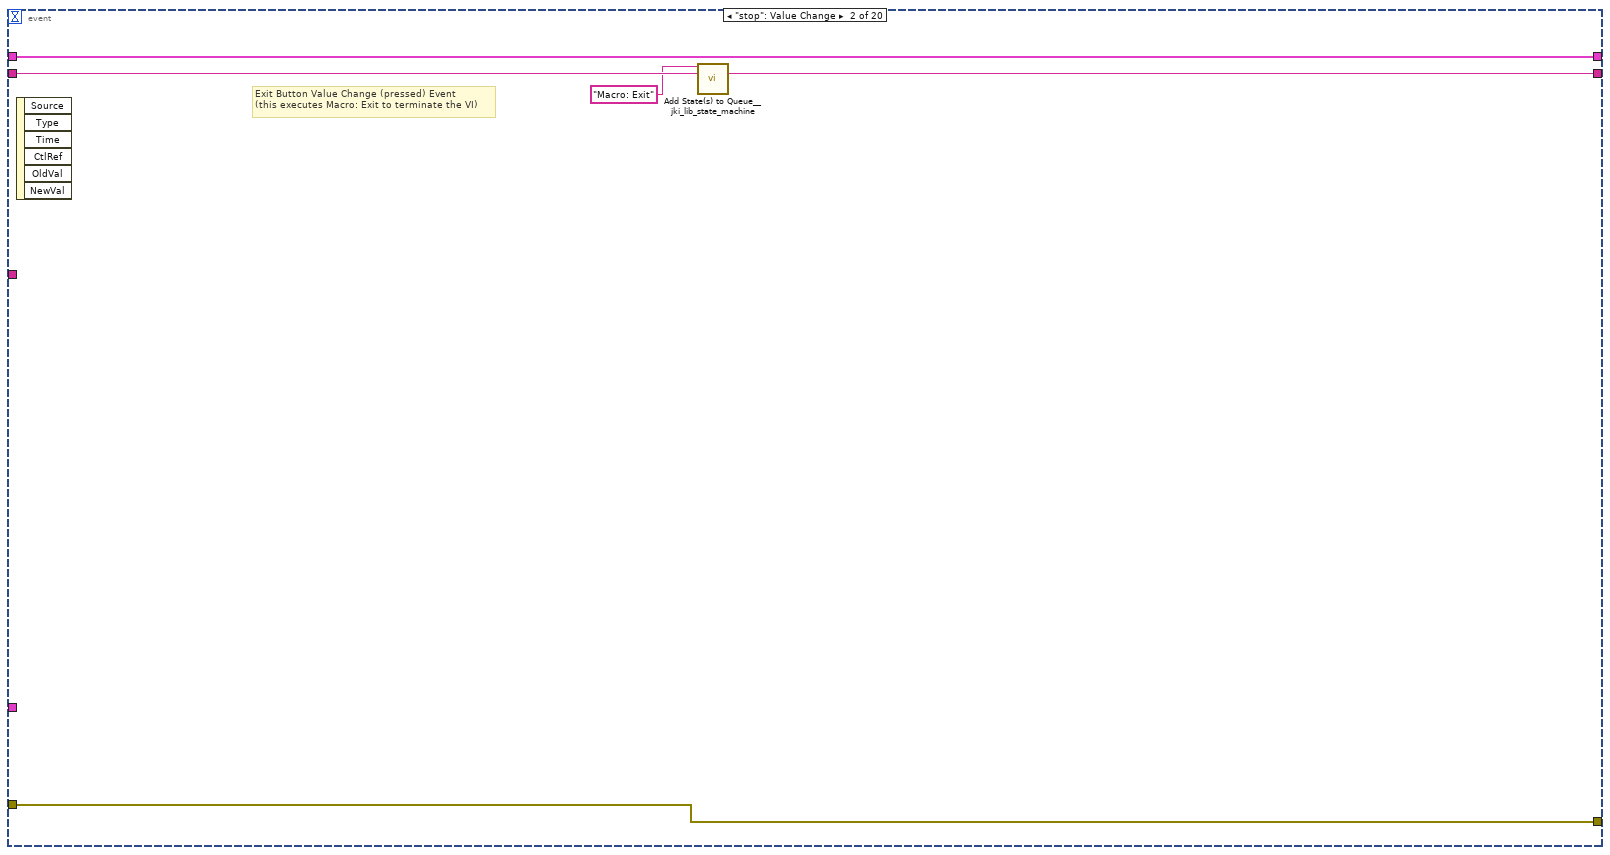
[diagram p7: hidden frame]
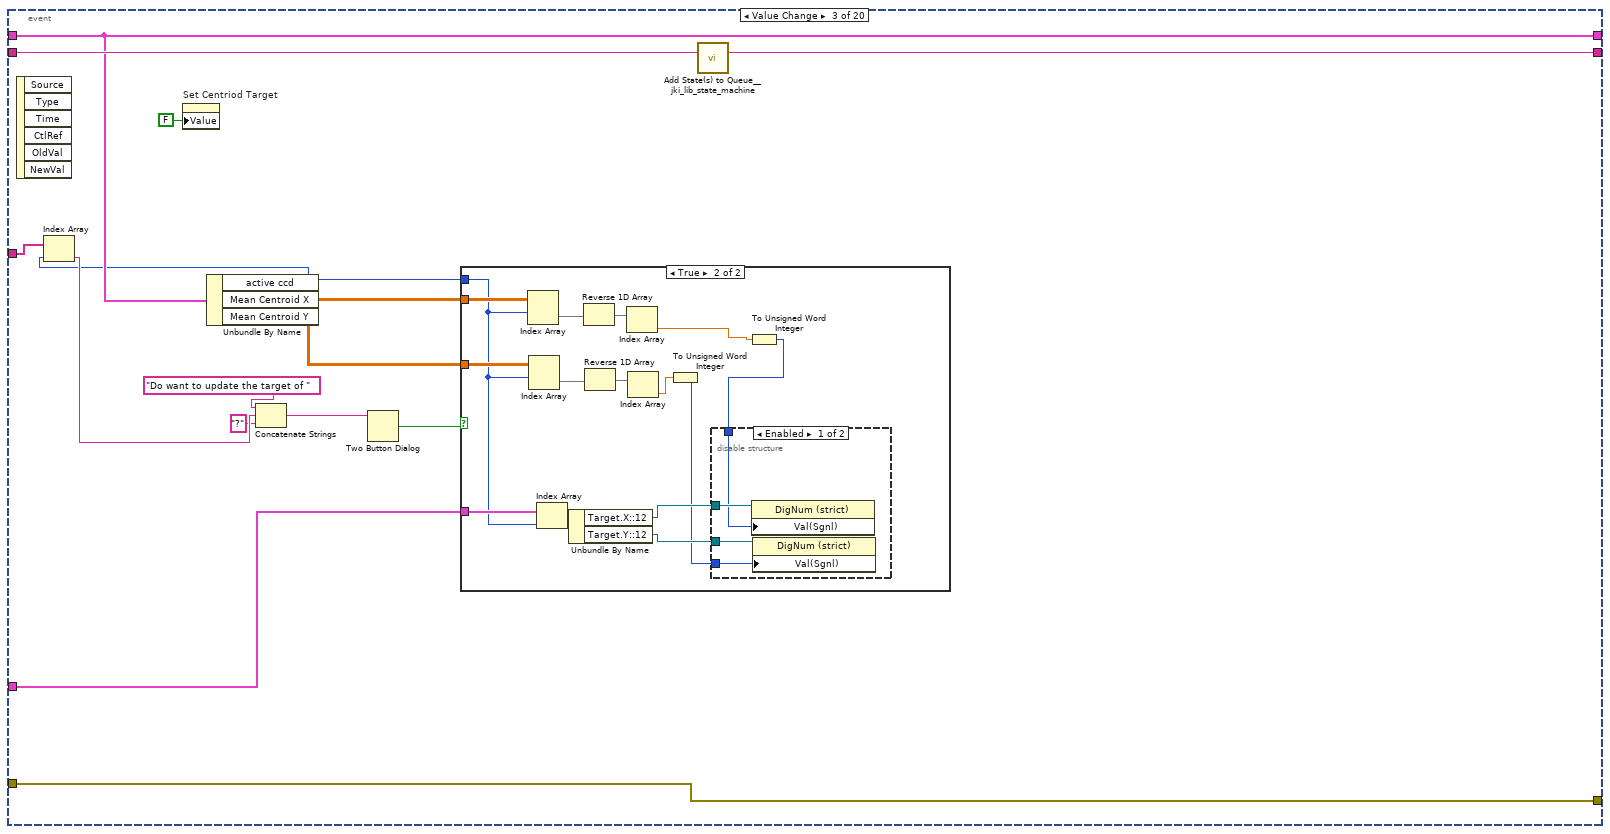
[diagram p8: hidden frame]
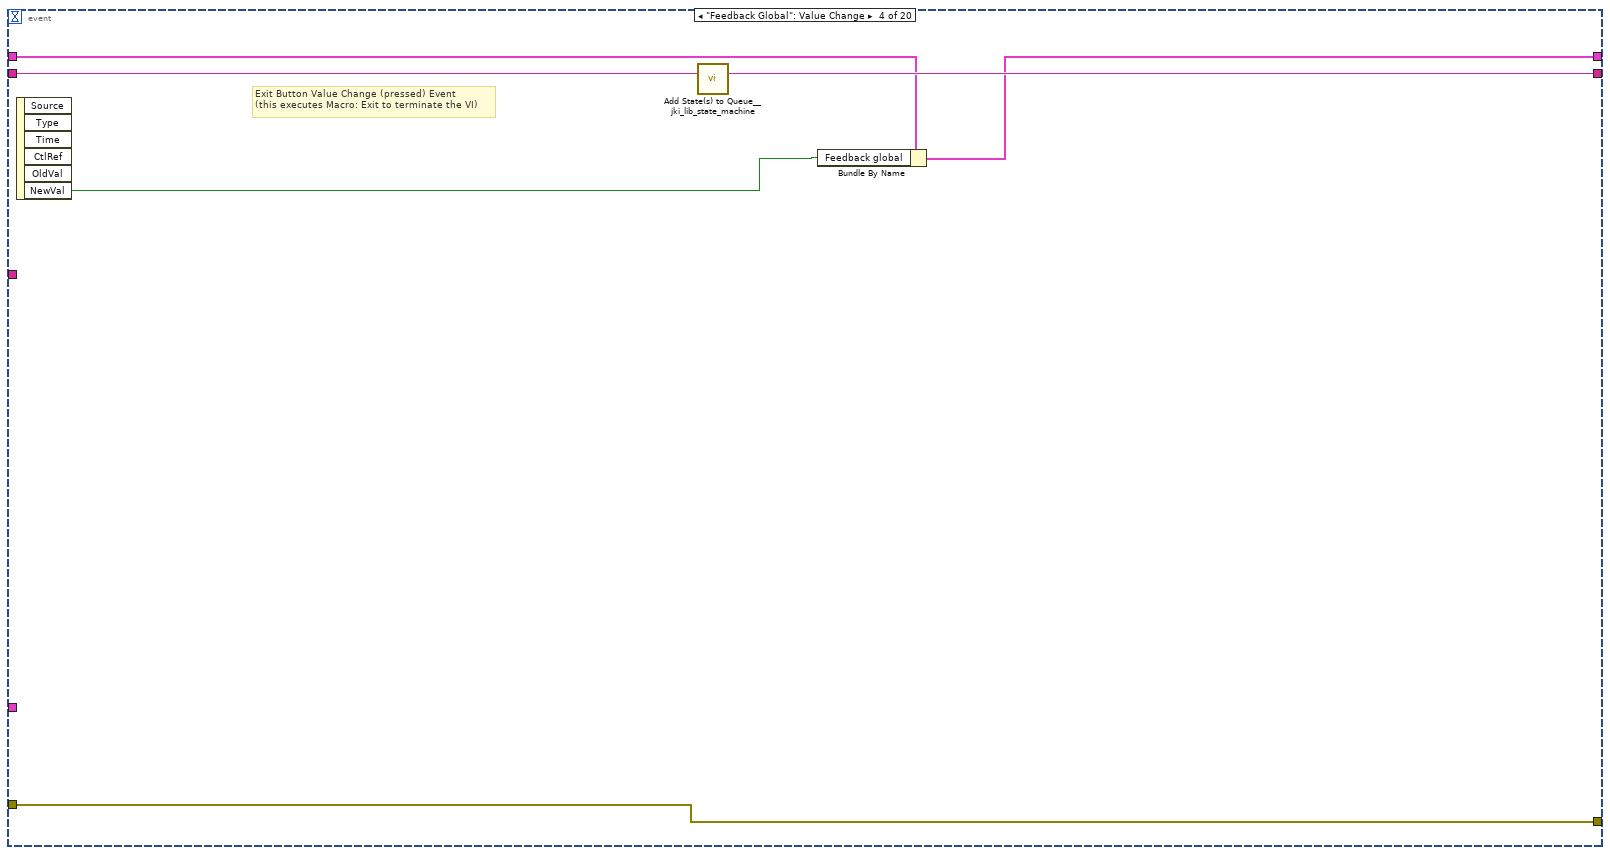
[diagram p11: hidden frame]
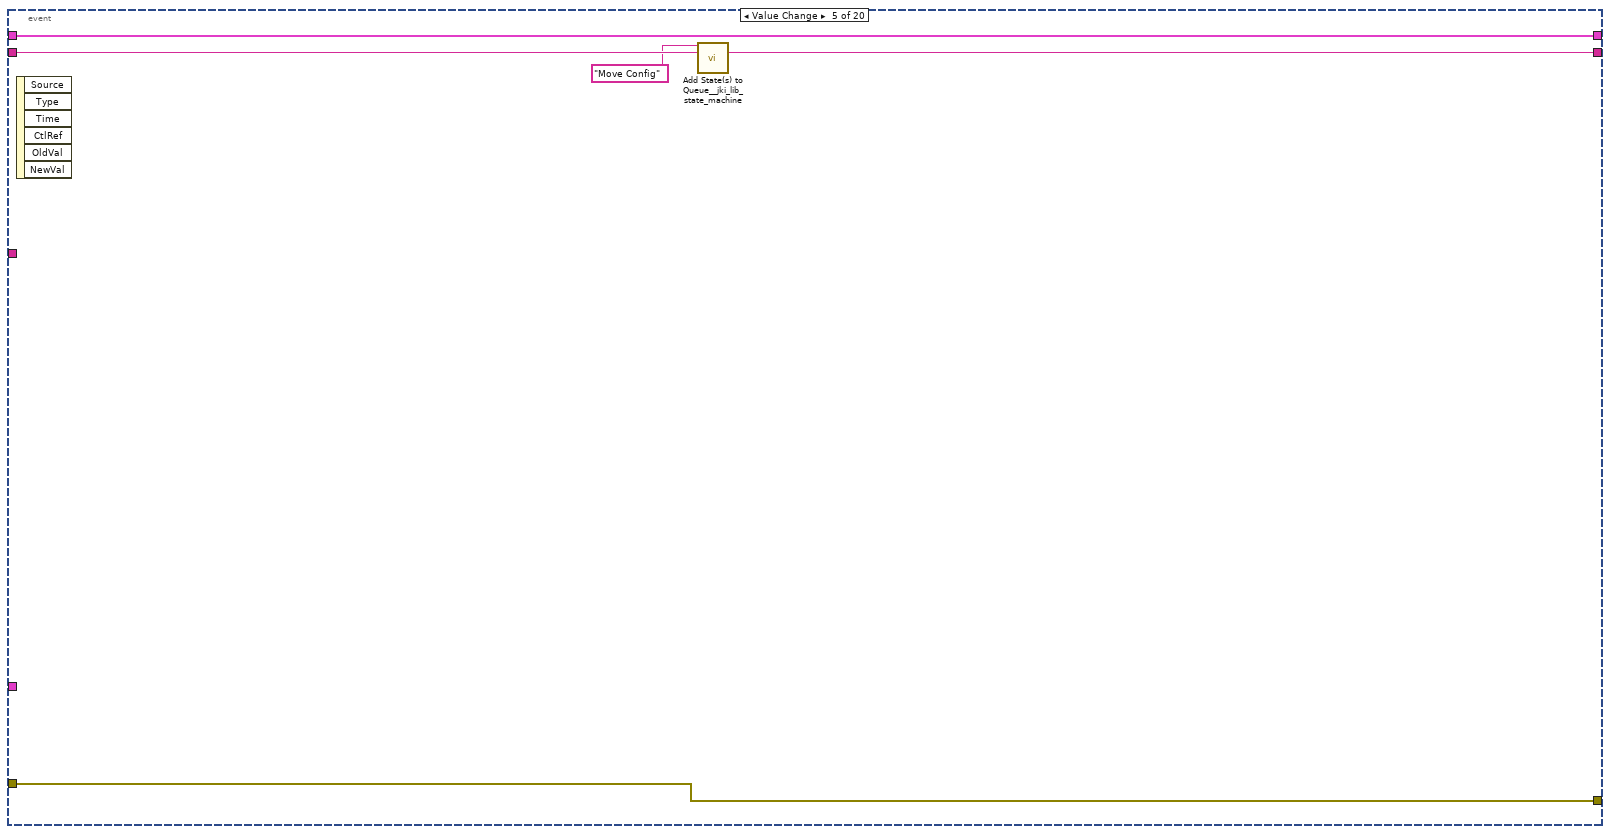
[diagram p12: hidden frame]
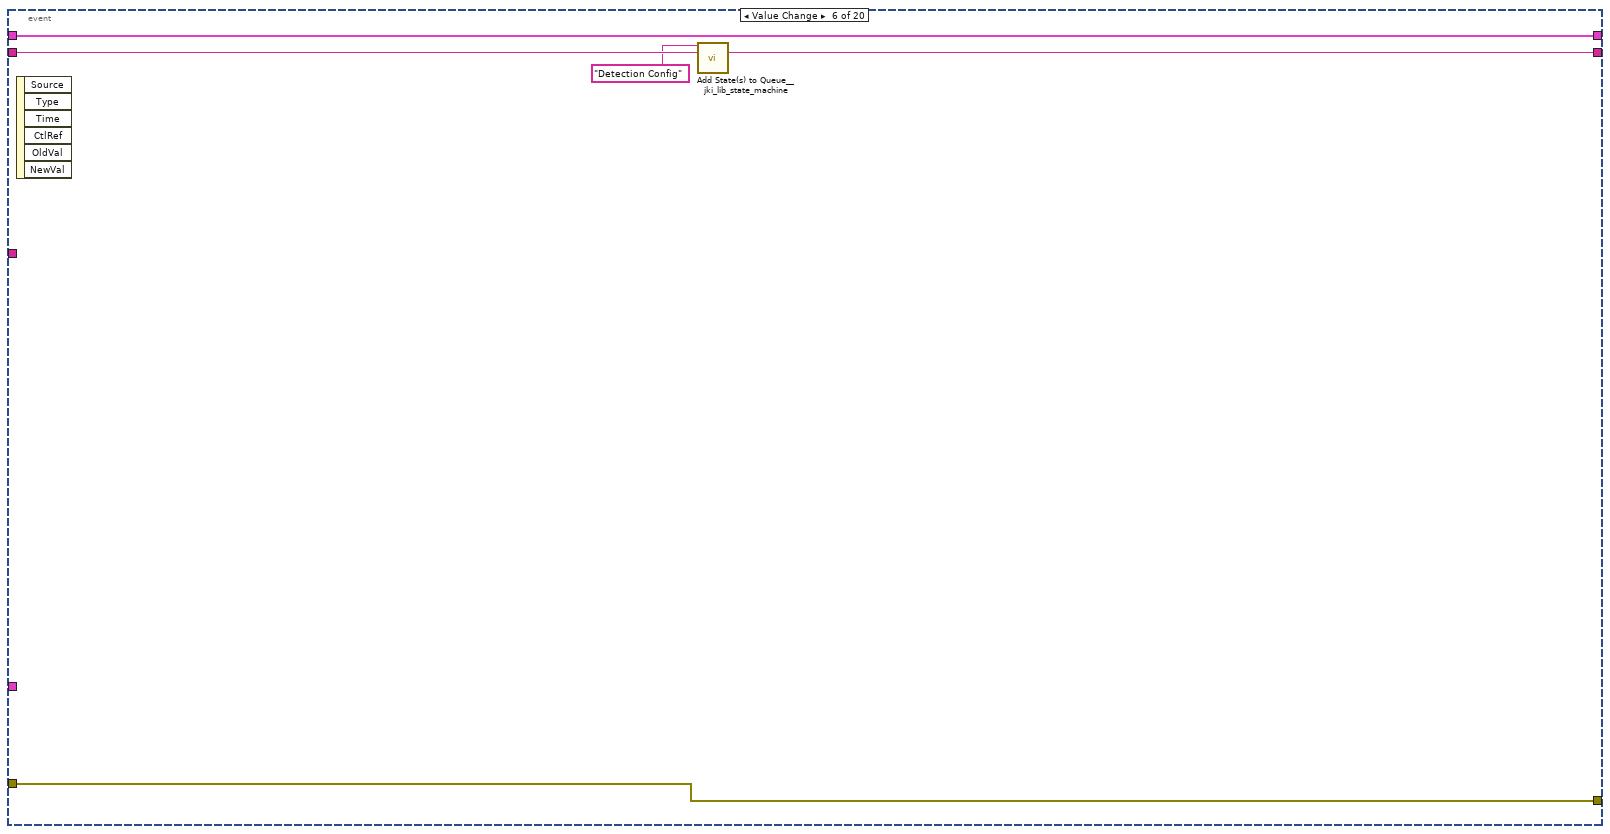
[diagram p13: hidden frame]
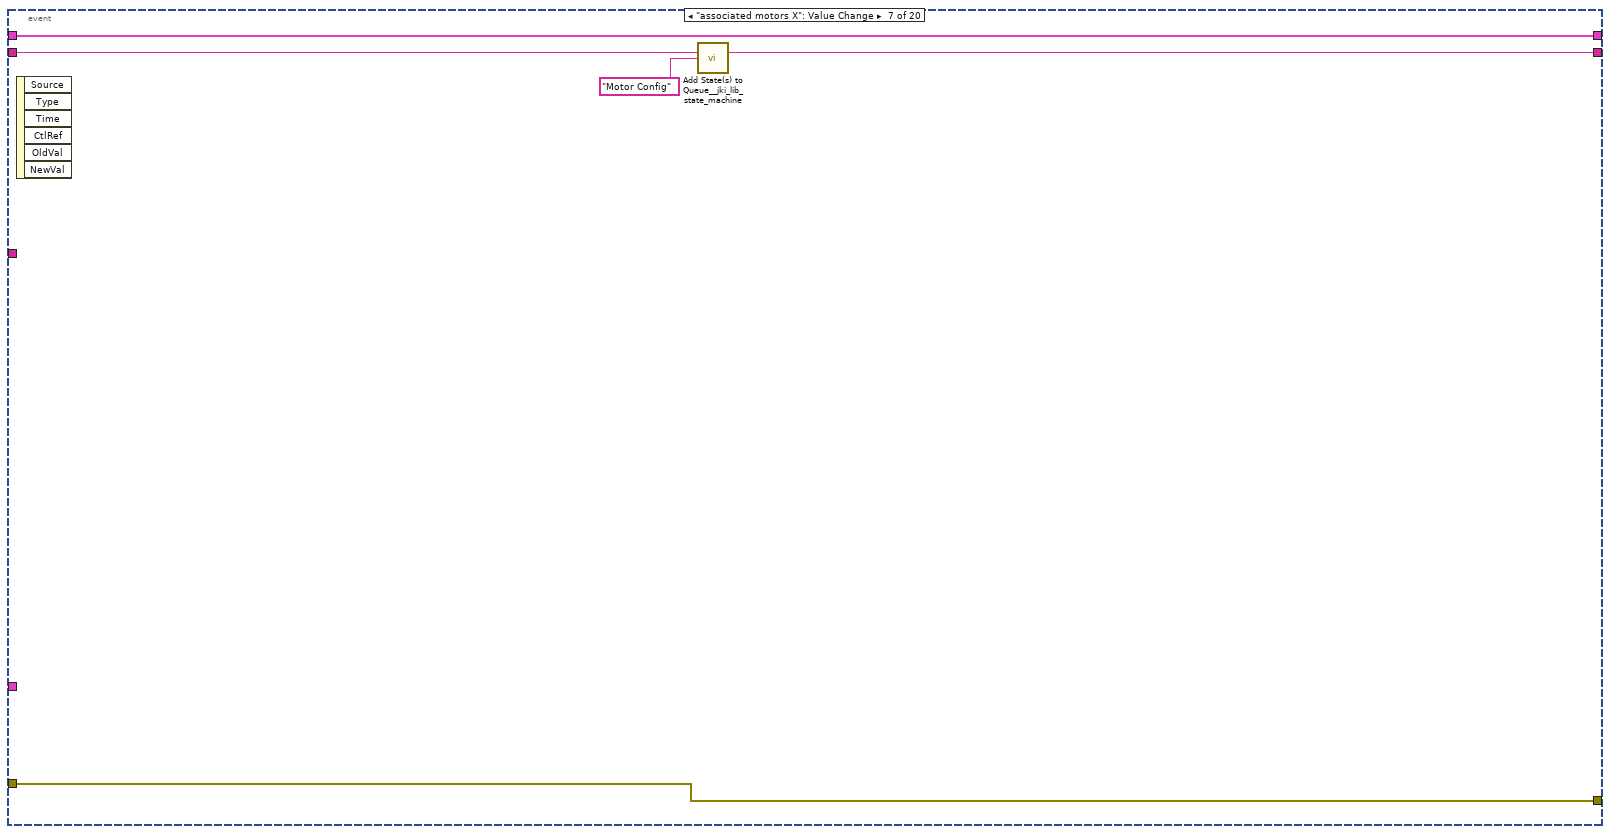
[diagram p14: hidden frame]
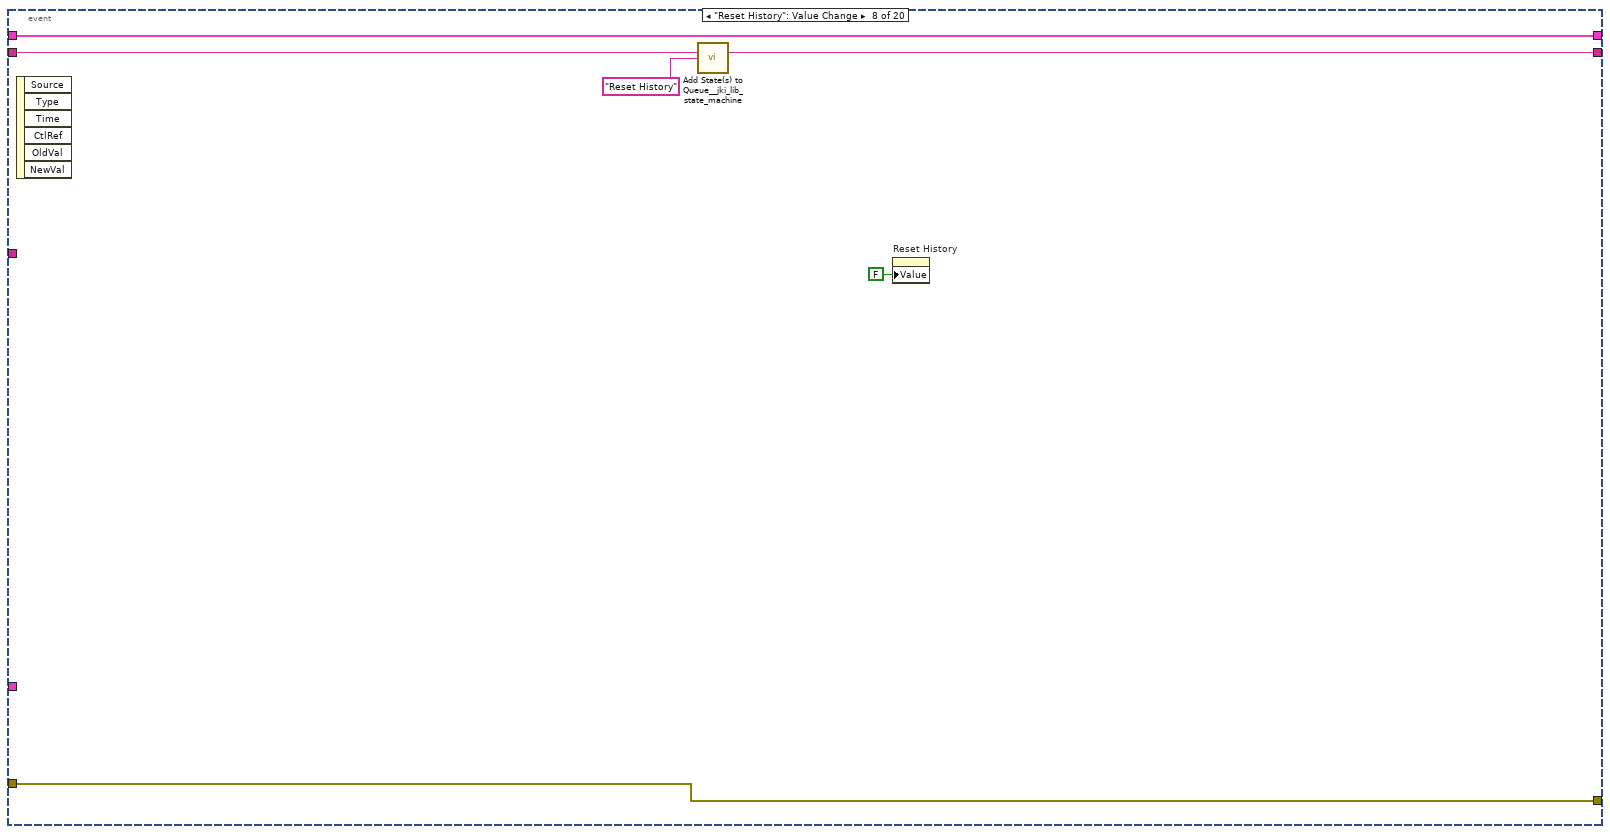
[diagram p15: hidden frame]
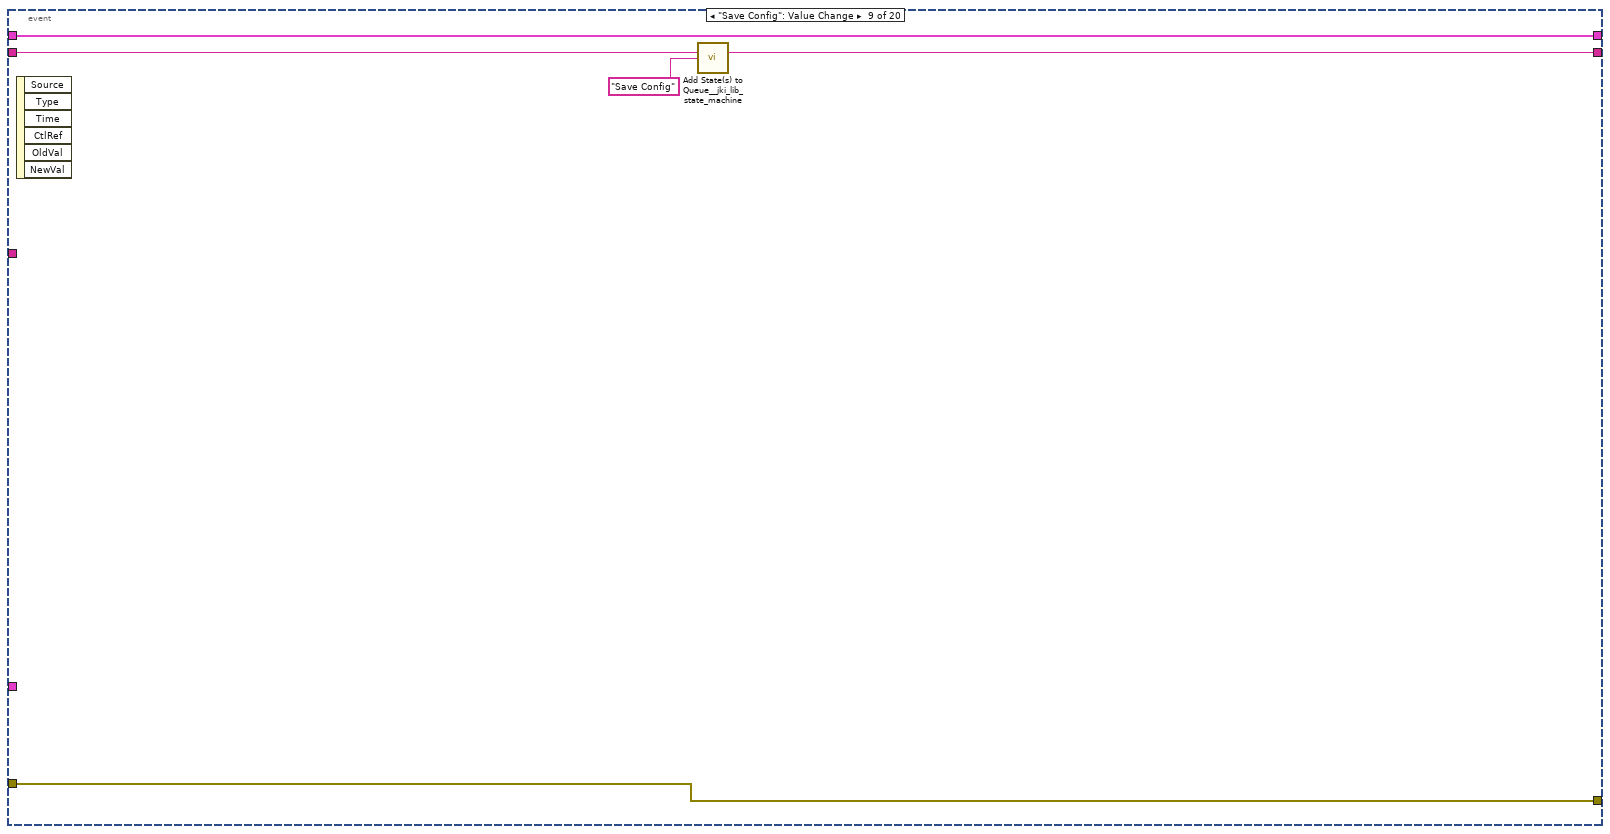
[diagram p16: hidden frame]
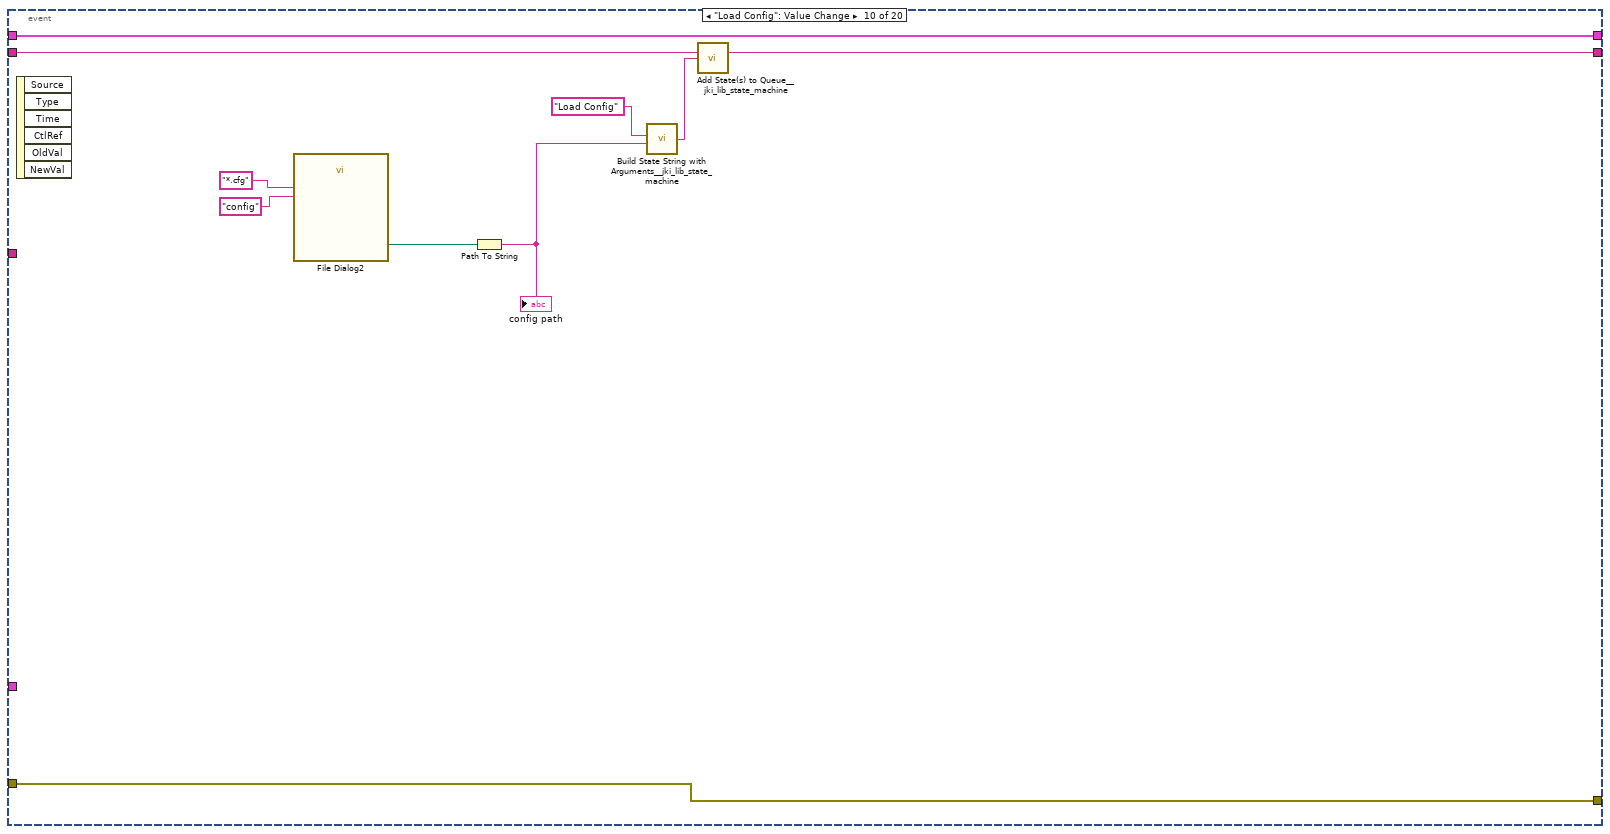
[diagram p17: hidden frame]
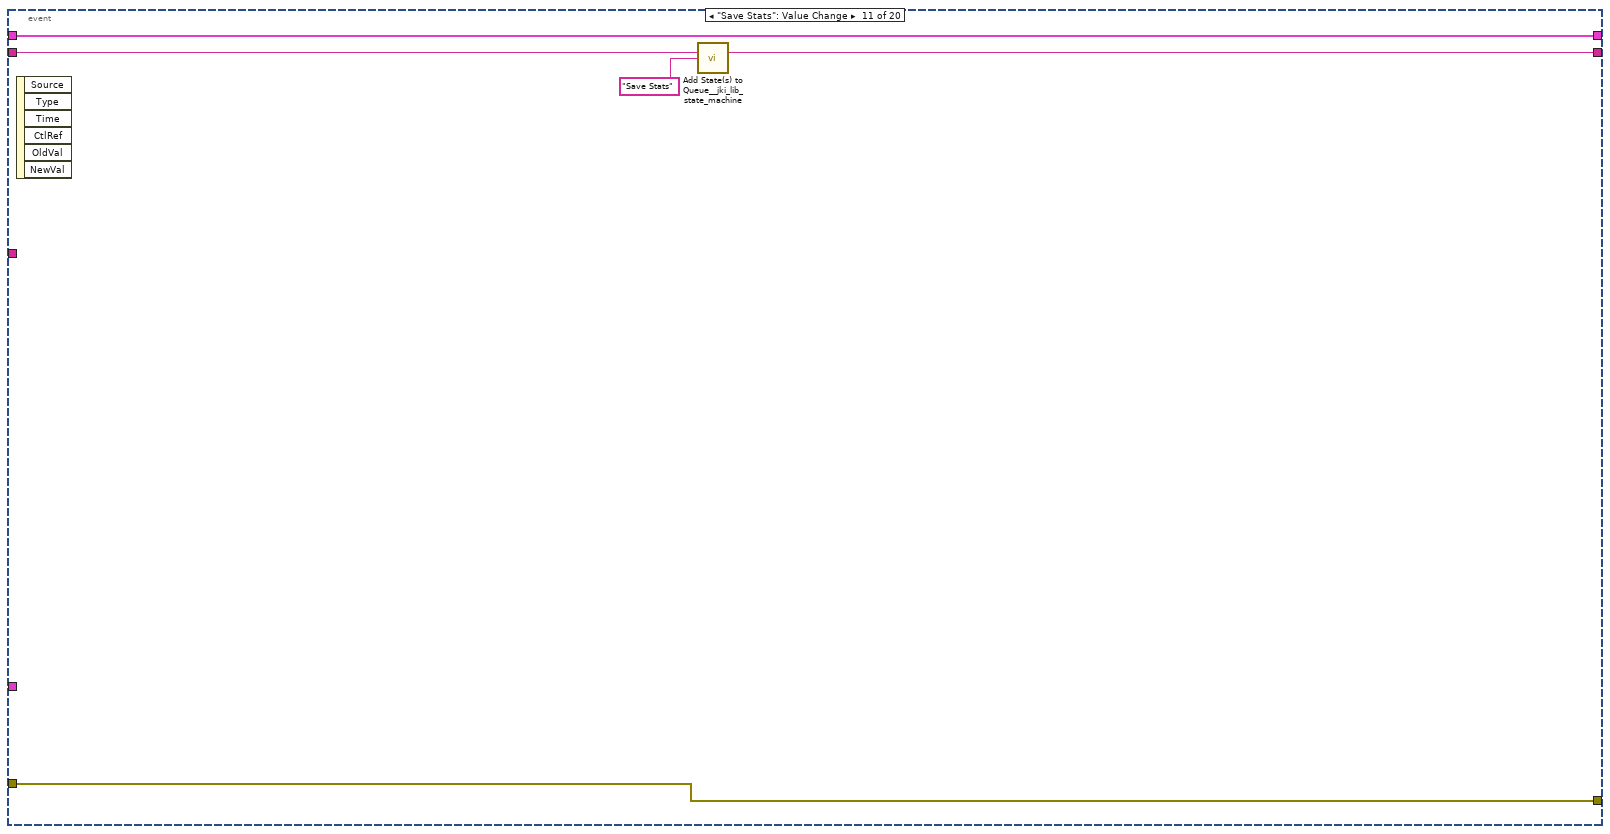
[diagram p18: hidden frame]
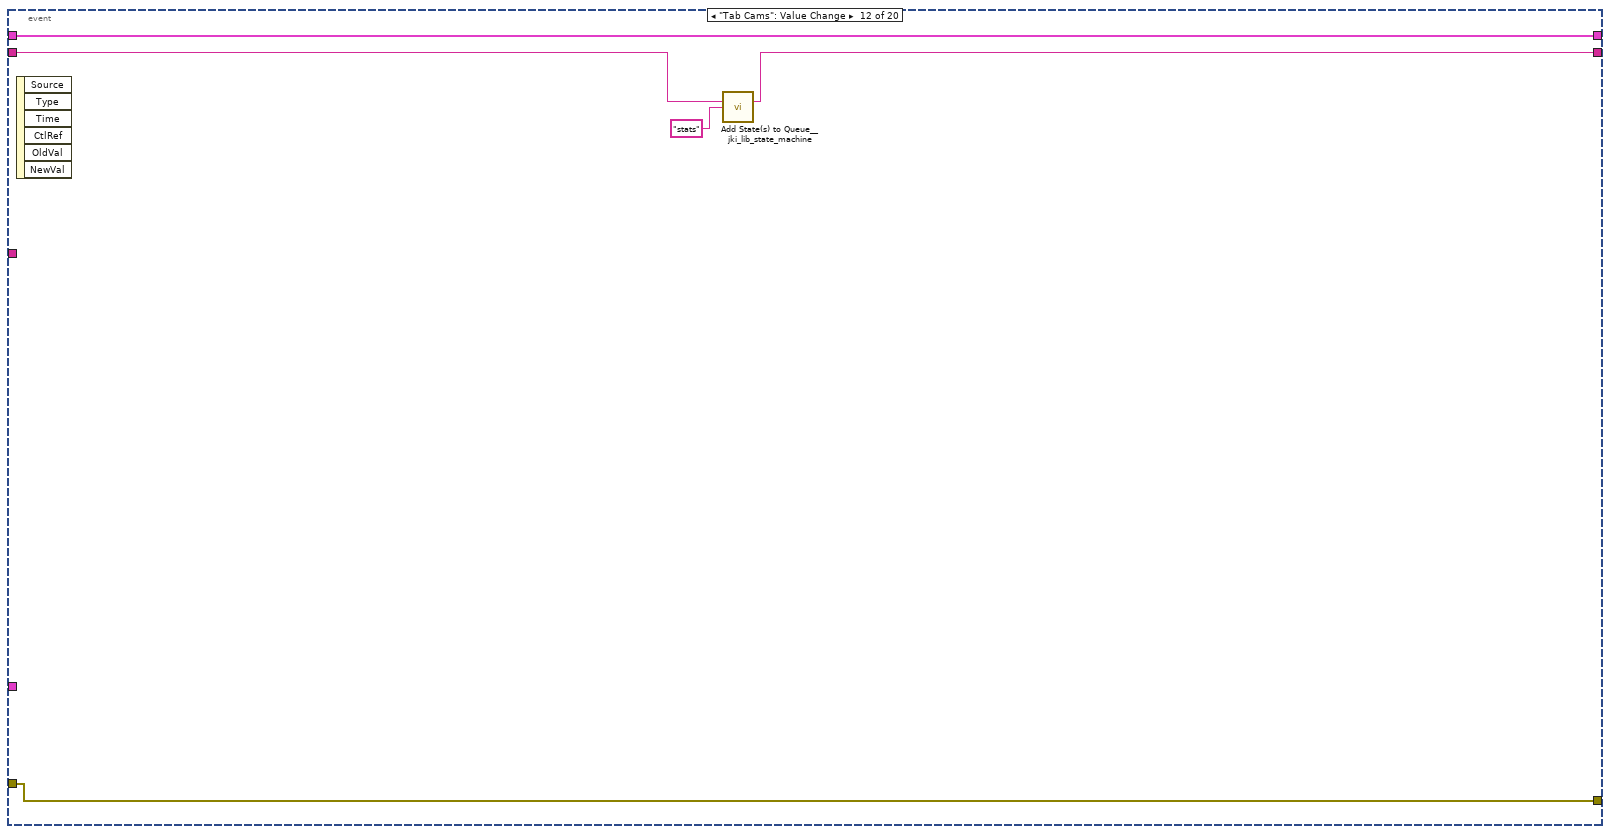
[diagram p19: hidden frame]
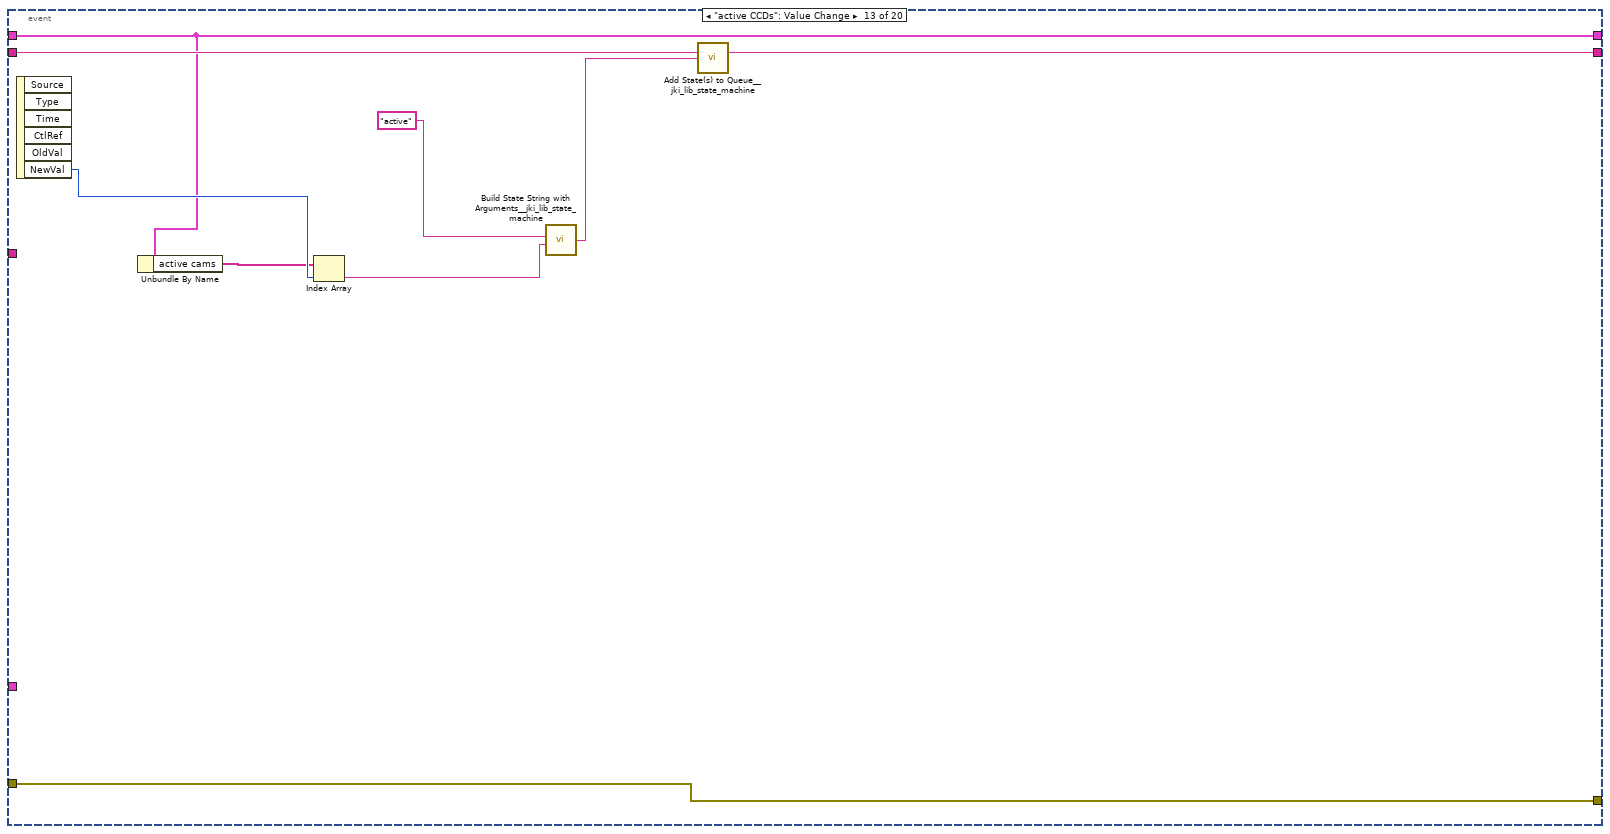
[diagram p20: hidden frame]
diagram:
  w2 = path "c:/BP_DATAsd" ("base path")
  # "MotorRefs"
  # "CameraRefs"
  # "Motor refs"
  n1 = control-ref of="Target.X::1"() -> (w51:refnum<vi>)
  n2 = control-ref of="Target.Y::1"() -> (w50:refnum<vi>)
  n3 = control-ref of="Target.X::2"() -> (w49:refnum<vi>)
  n4 = control-ref of="Target.Y::2"() -> (w48:refnum<vi>)
  n5 = control-ref of="Target.X::3"() -> (w47:refnum<vi>)
  n6 = control-ref of="Target.Y::3"() -> (w46:refnum<vi>)
  n7 = control-ref of="Target.X::4"() -> (w45:refnum<vi>)
  n8 = control-ref of="Target.Y::4"() -> (w44:refnum<vi>)
  n9 = control-ref of="Target.X::5"() -> (w43:refnum<vi>)
  n10 = control-ref of="Target.Y::5"() -> (w42:refnum<vi>)
  n11 = control-ref of="Target.X::6"() -> (w41:refnum<vi>)
  n12 = control-ref of="Target.Y::6"() -> (w40:refnum<vi>)
  n13 = control-ref of="Target.X::7"() -> (w39:refnum<vi>)
  n14 = control-ref of="Target.Y::7"() -> (w38:refnum<vi>)
  n15 = control-ref of="Target.X::8"() -> (w37:refnum<vi>)
  n16 = control-ref of="Target.Y::8"() -> (w36:refnum<vi>)
  n17 = control-ref of="Target.X::9"() -> (w15:refnum<vi>)
  n18 = control-ref of="Target.Y::9"() -> (w14:refnum<vi>)
  n19 = control-ref of="Target.X::10"() -> (w13:refnum<vi>)
  n20 = control-ref of="Target.Y::10"() -> (w12:refnum<vi>)
  n21 = control-ref of="Target.X::11"() -> (w11:refnum<vi>)
  n22 = control-ref of="Target.Y::11"() -> (w10:refnum<vi>)
  n23 = control-ref of="Target.X::12"() -> (w9:refnum<vi>)
  n24 = control-ref of="Target.Y::12"() -> (w8:refnum<vi>)
  n25 = Bundle("Target.X::1"=w51, "Target.Y::1"=w50) -> (w35:T12)  [unwired: 1 in]
  n26 = Bundle("Target.X::2"=w49, "Target.Y::2"=w48) -> (w34:T13)  [unwired: 1 in]
  n27 = Bundle("Target.X::3"=w47, "Target.Y::3"=w46) -> (w33:T14)  [unwired: 1 in]
  n28 = Bundle("Target.X::4"=w45, "Target.Y::4"=w44) -> (w26:T15)  [unwired: 1 in]
  n29 = Bundle("Target.X::5"=w43, "Target.Y::5"=w42) -> (w32:T16)  [unwired: 1 in]
  n30 = Bundle("Target.X::6"=w41, "Target.Y::6"=w40) -> (w31:T17)  [unwired: 1 in]
  n31 = Bundle("Target.X::7"=w39, "Target.Y::7"=w38) -> (w30:T18)  [unwired: 1 in]
  n32 = Bundle("Target.X::8"=w37, "Target.Y::8"=w36) -> (w29:T19)  [unwired: 1 in]
  n33 = Bundle("Target.X::12"=w9, "Target.Y::12"=w8) -> (w4:T20)  [unwired: 1 in]
  n34 = Bundle("Target.X::9"=w15, "Target.Y::9"=w14) -> (w7:T21)  [unwired: 1 in]
  n35 = Bundle("Target.X::10"=w13, "Target.Y::10"=w12) -> (w6:T22)  [unwired: 1 in]
  n36 = Bundle("Target.X::11"=w11, "Target.Y::11"=w10) -> (w5:T23)  [unwired: 1 in]
  n37 = Tick Count (ms)() -> (millisecond timer value=→"millisecond timer value":u32)
  n38 = Build Array(w35, w34, w33, w26, w32, w31, w30, w29, w7, w6, w5, w4) -> (w28:T24)
  n39 = Get Date/Time In Seconds() -> (seconds since 1Jan1904=w17:timestamp)
  n40 = Format Date/Time String(time format string (%c)="%Y%m%d%H%M", seconds (now)=w17) -> (date/time string=w16:string)  [unwired: 1 in]
  n41 = Concatenate Strings(w16, "Beampointing_BTL.tdms" ("string")) -> (w20:string)
  n42 = String To Path(string=w20) -> (path=w19:path)
  n43 = Build Path(base path=w2, name or relative path=w19) -> (appended path=w22:path)
  n44 = call <vilib>:"Add State(s) to Queue__jki_lib_state_machine.vi"("State(s) in (\"\")"="Macro: Initialize") -> ("States Out"=w55:string)  [unwired: 14 in]
  n45 = while "JKI - String-Based Queued State Machine (Basic) v1.0" {
    shift-right: [w69] -> w25
    shift-left: _ -> [w63]
    shift-right: [w72] -> w52
    shift-left: _ -> [w68]
    shift-right: [w71] -> _
    shift-left: w55 -> [w73]
    tunnel: w28 -> [w66]
    tunnel: [w56] -> w53
    tunnel: w28 -> [w65]
    tunnel: w22 -> [w61]
    tunnel: w2 -> [w60]
    stop <- w70 stop-if-true
    n46 = Unbundle By Name(w63) -> ("active cams"=w62:string[], "Mean Centroid X"=w59:dbl[][], "Mean Centroid Y"=w58:dbl[][], "Mean Size"=w57:dbl[][])
    n47 = call <vilib>:"Parse State Queue__jki_lib_state_machine.vi"("State Queue"=w73, "Error In (no error)"=w68) -> ("Remaining States"=w75:string, "Current State"=w76:string, "Arguments"=w74:string)  [unwired: 11 in]
    "Current State" <- w76
    n48 = local read "CCDs"() -> (w56:string[])
    n49 = case shown="\"Save Config\"" w76 {
      selector: w76 -> [_ _ w424 _ _ _ _ _ _ _ _ _ _ _ _ _ _ _ _ _ _ _ _ _ _ _ _ _ _ _ _ _ _ _ _ _ _ _ _ _ _ _ _ _ _ _ _]
      tunnel: w75 -> [w141 w423 w428 w446 w452 w457 w461 w503 w519 w527 w531 w535 w541 w552 w576 w585 w596 w600 w637 w658 w701 w721 w749 w874 w930 w973 w982 w1017 w1033 w1037 w1056 w1201 w1364 w1416 w1455 w1506 w1558 w1582 w1597 w1671 w1723 w1733 w1774 w1869 w1895 w1909 w1932]
      tunnel: w74 -> [_ _ _ _ _ _ _ _ _ _ _ _ w536 w547 _ _ _ _ _ _ _ _ w725 w839 _ w958 _ _ _ _ w1057 _ w1345 w1401 w1439 w1487 w1552 _ _ _ _ _ _ _ _ w1913 _]
      tunnel: w63 -> [w139 w420 w426 w436 w449 w455 w458 _ w514 w522 w528 w533 w539 w546 w573 w582 w588 w597 w635 w656 w699 w706 w740 w864 w928 w954 w978 w1009 w1026 w1034 w1045 w1184 w1342 w1412 w1451 w1479 w1554 w1579 w1594 w1667 w1720 w1730 w1748 w1867 w1892 w1912 w1923]
      tunnel: [w138 w421 w430 w444 errorcluster {"status"=FALSE, "code"=0, "source"=""} ("error out") w454 w459 w470 w516 w520 w529 w532 w537 w549 w574 w583 w594 w598 w634 w655 w698 w703 w743 w842 w926 w962 w980 w1015 w1031 w1035 w1086 w1214 w1362 w1414 w1453 w1504 w1547 w1580 w1595 w1668 w1721 w1731 w1741 w1831 w1893 w1907 w1930] -> w72
      tunnel: w68 -> [w137 w421 w429 w444 w448 w454 w459 w471 w517 w521 w529 w532 w538 w550 w574 w583 w594 w598 w634 w655 w698 w704 w744 w840 w927 w961 w980 w1015 w1031 w1035 w1086 w1214 w1362 w1414 w1453 w1504 w1548 w1580 w1595 w1669 w1721 w1731 w1742 w1865 w1893 w1907 w1930]
      tunnel: [w140 w422 w427 w445 w451 w456 w460 w502 w518 w526 w530 w534 w540 w551 w575 w584 w595 w599 w636 w657 w700 w720 w734 w873 w929 w972 w981 w1016 w1032 w1036 w1039 w1215 w1363 w1415 w1454 w1505 w1557 w1581 w1596 w1670 w1722 w1732 w1773 w1868 w1894 w1908 w1931] -> w71
      tunnel: [_ _ _ _ _ TRUE _ _ _ _ _ _ _ _ _ _ _ _ _ _ _ _ _ _ _ _ _ _ _ _ _ _ _ _ _ _ _ _ _ _ _ _ _ _ _ _ _] -> w70
      tunnel: [w134 w420 w426 w435 w449 w455 w458 w472 w514 w522 w528 w533 w539 w546 w573 w582 w588 w597 w635 w656 w699 w705 w746 w863 w928 w967 w977 w1008 w1025 w1034 w1038 w1185 w1342 w1412 w1451 w1479 w1556 w1579 w1594 w1667 w1719 w1730 w1748 w1866 w1892 w1911 w1922] -> w69
      tunnel: "update speed [ms]" -> [w136 _ _ _ _ _ _ _ _ _ _ _ _ _ _ _ _ _ _ _ _ _ _ _ _ _ _ _ _ _ _ _ _ _ _ _ _ _ _ _ _ _ _ _ _ _ _]
      tunnel: w66 -> [w133 _ _ _ _ _ _ _ _ _ _ _ _ _ _ _ _ _ _ _ _ _ _ _ _ _ _ _ _ _ w1078 _ _ _ _ _ _ _ _ _ _ _ _ _ w1877 _ _]
      tunnel: w56 -> [w135 _ _ _ _ _ _ w467 _ _ _ _ _ _ _ _ _ _ _ _ _ _ w748 w862 _ w968 _ _ _ _ w1049 w1186 w1361 _ _ w1503 w1553 _ w1584 _ _ _ w1747 _ _ _ _]
      tunnel: w61 -> [_ _ _ _ _ _ _ w469 _ _ _ _ _ _ _ _ _ _ _ _ _ _ w745 _ _ _ _ _ _ _ _ _ _ _ _ _ _ _ _ _ _ _ _ _ _ _ _]
      tunnel: w60 -> [_ _ _ _ _ _ _ _ _ _ _ _ _ _ _ _ _ _ _ _ _ _ _ _ _ _ _ _ _ _ _ _ _ _ _ _ _ _ _ _ _ _ _ w1837 _ _ _]
      frame "", "Idle" {
        # "executes when the state queue is empty"
        n50 = event shown="[0] Timeout" {
          selector: _ -> [_ _ _ _ _ _ _ _ _ _ _ _ _ _ _ _ _ _ _ _]
          dyn-events: _ -> [_ _ _ _ _ _ _ _ _ _ _ _ _ _ _ _ _ _ _ _]
          timeout: w136 -> [_ _ _ _ _ _ _ _ _ _ _ _ _ _ _ _ _ _ _ _]
          tunnel: w141 -> [w146 w270 w285 w310 w315 w320 w325 w331 w336 w346 w351 w353 w365 w377 w389 w394 w399 w405 w409 w419]
          tunnel: [w171 w269 w284 w309 w314 w319 w324 w330 w335 w345 w350 w352 w364 w376 w388 w393 w398 w404 w408 w418] -> w140
          tunnel: w139 -> [w167 w267 w281 w306 w312 w317 w322 w328 w333 w343 w348 w356 w358 w375 w387 w392 w397 w403 w410 w416]
          tunnel: [w182 w268 w283 w308 w313 w318 w323 w329 w334 w344 w349 w355 w363 w370 w382 w391 w396 w402 w407 w417] -> w138
          tunnel: w137 -> [w158 w268 w283 w308 w313 w318 w323 w329 w334 w344 w349 w355 w363 w371 w383 w391 w396 w402 w407 w417]
          tunnel: [w170 w267 w281 w305 w312 w317 w322 w328 w333 w343 w348 w356 w358 w375 w387 w392 w397 w403 w410 w416] -> w134
          tunnel: w135 -> [w163 _ w277 _ _ _ _ _ _ _ _ _ _ _ _ _ _ _ _ _]
          tunnel: w133 -> [_ _ w279 _ _ _ _ _ _ _ _ _ _ _ _ _ _ _ _ _]
          event Timeout {
            n51 = event-data() -> ()  [unwired: 1 in, 1 out]
            n52 = Unbundle By Name(w167) -> ("Centroid X"=w164:dbl[][], "Centroid Y"=w161:dbl[][], "Size"=w159:dbl[][], "detection para"=w154:T7[], "active cams"=w162:string[], "thresholds"=w160:cluster{"Lower value":sgl, "Upper value":sgl}[])
            n53 = Unbundle By Name(w167) -> ("img to avg"=w143:i32, "active ccd"=w166:i32)
            n54 = for {
              tunnel: w162 -> [w203] mode=indexing
              tunnel: [w204] -> w150 mode=indexing
              tunnel: w163 -> [w226]
              tunnel: w154 -> [w224]
              tunnel: [w187] -> w149 mode=indexing
              tunnel: [w222] -> w157 mode=indexing
              tunnel: [w220] -> w165 mode=indexing
              tunnel: "autodetect" -> [w214]
              tunnel: w158 -> [w227]
              tunnel: [w228] -> w156
              shift-right: [w211] -> w153
              shift-left: w160 -> [w213]
              shift-right: [w198] -> w142
              shift-left: w164 -> [w200]
              shift-right: [w194] -> w152
              shift-left: w161 -> [w196]
              shift-right: [w188] -> w151
              shift-left: w159 -> [w190]
              w192 = 0 ("index")
              n55 = call-poly <userlib>:"Filter 1D Array__ogtk.vi"("items to filter"=w203, "array"=w226) -> ("filtered item indices"=w225:i32[])  [unwired: 4 in, 1 out]
              n56 = Index Array(array=w225) -> (element=w189:i32)  [unwired: 1 in]
              n57 = Index Array(array=w190, index (row)=w189) -> (element=w218:dbl[])  [unwired: 1 in]
              n58 = Index Array(array=w196, index (row)=w189) -> (element=w219:dbl[])  [unwired: 1 in]
              n59 = Index Array(array=w213, index=w189) -> (element=w217:cluster{"Lower value":sgl, "Upper value":sgl})
              n60 = Index Array(array=w200, index (row)=w189) -> (element=w202:dbl[])  [unwired: 1 in]
              n61 = Index Array(array=w224, index=w189) -> (element=w221:T7)
              n62 = call "CENTRIOD DETECTION.vi"("Refnum in"=w203, "auto threshold"=w214, "Threshold Range In"=w217, "beam detection para"=w221, "error in (no error)"=w227) -> ("Bounding Rect"=w220:T33, "Particle Reports (Pixels)"=w222:T2, "Threshold Range Out"=w212:cluster{"Lower value":sgl, "Upper value":sgl}, "Centriod"=w229:cluster{"X":dbl, "Y":dbl}, "error out"=w228:errorcluster)  [unwired: 7 in, 3 out]
              n63 = Unbundle By Name(w229) -> ("X"=w201:dbl, "Y"=w197:dbl)
              n64 = Empty Array?(array=w222) -> (empty?=w223:bool)
              n65 = Not(x=w223) -> (.not. x?=w187:bool)
              n66 = Replace Array Subset(array=w213, new element=w212, index=w189) -> (w211:cluster{"Lower value":sgl, "Upper value":sgl}[])
              n67 = Unbundle By Name(w220) -> ("Right"=w210:dbl, "Left"=w209:dbl, "Bottom"=w208:dbl, "Top"=w207:dbl)
              n68 = Subtract(x=w210, y=w209) -> (x-y=w205:dbl)
              n69 = Subtract(x=w208, y=w207) -> (x-y=w206:dbl)
              n70 = Multiply(x=w205, y=w206) -> (x*y=w193:dbl)
              n71 = Insert Into Array(array=w219, index=w192, new element=w197) -> (w195:dbl[])
              n72 = Insert Into Array(array=w202, index=w192, new element=w201) -> (w199:dbl[])
              n73 = Insert Into Array(array=w218, index=w192, new element=w193) -> (w191:dbl[])
              n74 = for {
                shift-right: [w230] -> w215
                shift-left: dbl[] [] ("Array 4") -> [w233]
                tunnel: w195 -> [w231] mode=indexing
                n75 = Equal To 0?(x=w231) -> (x = 0?=w232:bool)
                n76 = case shown="False" w232 {
                  tunnel: w233 -> [w236 w237]
                  tunnel: w231 -> [w235 _]
                  tunnel: [w234 w237] -> w230
                  frame False {
                    n77 = Build Array (concatenate)(w236, w235) -> (w234:dbl[])
                  }
                  frame True {
                  }
                }
              }
              n78 = Replace Array Subset(array=w200, new element=w199, index (row)=w189) -> (w198:dbl[][])  [unwired: 1 in]
              n79 = Replace Array Subset(array=w196, new element=w195, index (row)=w189) -> (w194:dbl[][])  [unwired: 1 in]
              n80 = Replace Array Subset(array=w190, new element=w191, index (row)=w189) -> (w188:dbl[][])  [unwired: 1 in]
              n81 = Array Size(array=w215) -> (size(s)=w204:i32)
            }
            "detected" <- w149
            "Box" <- w165
            n82 = Index Array(array=w157, index (row)=w166) -> (element=→"particles":T2)  [unwired: 1 in]
            n83 = call <vilib>:"Clear Errors.vi"("error in (no error)"=w156) -> ("error out"=w182:errorcluster)  [unwired: 5 in, 1 out]
            n84 = local read "Numeric"() -> (w175:dbl)
            n85 = Increment(x=w143) -> (x+1=w172:i32)
            n86 = Greater Or Equal?(x=w175, y=w172) -> (x >= y?=w169:bool)
            n87 = Increment(x=w175) -> (x+1=w174:dbl)
            n88 = Select(t=0.0, s=w169, f=w174) -> (s? t:f=w173:dbl)
            n89 = local write "Numeric"(w173) -> ()
            n90 = Bundle By Name(cluster=w167, "thresholds"=w153) -> (w178:T34)
            n91 = for {
              tunnel: w150 -> [w259] mode=indexing
              tunnel: w162 -> [w265] mode=indexing
              shift-right: [w260] -> w183
              shift-left: "" ("GUIdevice 7") -> [w263]
              tunnel: [w254] -> w185 mode=indexing
              tunnel: "Detection Rate" -> [w258]
              tunnel: w173 -> [w256]
              tunnel: w143 -> [w252]
              n92 = Greater Or Equal?(x=w259, y=w252) -> (x >= y?=w255:bool)
              n93 = Multiply(x=w258, y=w256) -> (x*y=w257:dbl)
              n94 = Greater Or Equal?(x=w259, y=w257) -> (x >= y?=w253:bool)
              n95 = And(x=w255, y=w253) -> (x .and. y?=w254:bool)
              n96 = Select(t=w265, s=w254, f="") -> (s? t:f=w261:string)
              n97 = Concatenate Strings(w263, "\t", w261) -> (w260:string)
            }
            n98 = Bundle(0, 1, "Centroid X"=w142) -> (→"Status":cluster{i32, i32, "Centroid X":dbl[][]})  [unwired: 1 in]
            n99 = call <vilib>:"Add State(s) to Queue__jki_lib_state_machine.vi"("State(s) in (\"\")"=w146, "State(s) at Back (\"\")"="Device Ini" ("State(s) at Back (\"\")")) -> ("States Out"=w145:string)  [unwired: 13 in]
            n100 = Bundle By Name(cluster=w178, "Centroid X"=w142, "Centroid Y"=w152, "Size"=w151) -> (w148:T34)
            n101 = Unbundle By Name(w148) -> ("img to avg"=w147:i32)
            n102 = case shown="True" w169 {
              tunnel: w148 -> [w238 w245]
              tunnel: [w238 w244] -> w170
              tunnel: w147 -> [_ w240]
              frame False {
              }
              frame True {
                n103 = Decrement(x=w240) -> (x-1=w243:i32)
                n104 = Initialize Array(0.0 ("element"), 12 ("dimension size"), w243) -> (w239:dbl[][])
                n105 = Bundle By Name(cluster=w245, "Centroid X"=w239, "Centroid Y"=w239, "Size"=w239) -> (w244:T34)
              }
            }
            n106 = Or Array Elements(Boolean array=w185) -> (logical OR=w184:bool)
            n107 = case shown="True" w184 {
              tunnel: w183 -> [_ w250]
              tunnel: w145 -> [w246 w249]
              tunnel: [w246 w248] -> w171
              frame False {
              }
              frame True {
                n108 = call <vilib>:"Build State String with Arguments__jki_lib_state_machine.vi"("Arguments (\"\")"=w250, "State"="detected") -> ("State with Arguments"=w247:string)  [unwired: 4 in]
                n109 = call <vilib>:"Add State(s) to Queue__jki_lib_state_machine.vi"("State(s) in Front (\"\")"=w247, "State(s) in (\"\")"=w249) -> ("States Out"=w248:string)  [unwired: 13 in]
              }
            }
          }
          event "stop": Value Change {
            # "Exit Button Value Change (pressed) Event\n(this executes Macro: Exit to terminate the VI)"
            n110 = event-data() -> ()  [unwired: 1 in, 6 out]
            n111 = call <vilib>:"Add State(s) to Queue__jki_lib_state_machine.vi"("State(s) in Front (\"\")"="Macro: Exit", "State(s) in (\"\")"=w270) -> ("States Out"=w269:string)  [unwired: 13 in]
          }
          event Value Change {
            n112 = event-data() -> ()  [unwired: 1 in, 6 out]
            n113 = property on="Set Centriod Target" class="Bool (strict)"("Value"=FALSE) -> ()  [unwired: 2 in, 2 out]
            n114 = Unbundle By Name(w281) -> ("active ccd"=w273:i32, "Mean Centroid X"=w272:dbl[][], "Mean Centroid Y"=w271:dbl[][])
            n115 = Index Array(array=w277, index=w273) -> (element=w276:string)
            n116 = Concatenate Strings("Do want to update the target of " ("message"), w276, "?" ("string")) -> (w274:string)
            n117 = Two Button Dialog(message=w274) -> (T button?=w280:bool)  [unwired: 2 in]
            n118 = case shown="True" w280 {
              tunnel: w279 -> [_ w294]
              tunnel: w273 -> [_ w293]
              tunnel: w272 -> [_ w300]
              tunnel: w271 -> [_ w295]
              frame False {
              }
              frame True {
                n119 = Index Array(array=w300, index (row)=w293) -> (element=w299:dbl[])  [unwired: 1 in]
                n120 = Index Array(array=w295, index (row)=w293) -> (element=w296:dbl[])  [unwired: 1 in]
                n121 = Index Array(array=w294, index=w293) -> (element=w292:T20)
                n122 = Unbundle By Name(w292) -> ("Target.X::12"=w291:refnum<vi>, "Target.Y::12"=w290:refnum<vi>)
                n123 = Reverse 1D Array(array=w299) -> (reversed array=w298:dbl[])
                n124 = Reverse 1D Array(array=w296) -> (reversed array=w297:dbl[])
                n125 = Index Array(array=w298) -> (element=w289:dbl)  [unwired: 1 in]
                n126 = Index Array(array=w297) -> (element=w287:dbl)  [unwired: 1 in]
                n127 = To Unsigned Word Integer(number=w287) -> (unsigned 16bit integer=w286:u16)
                n128 = To Unsigned Word Integer(number=w289) -> (unsigned 16bit integer=w288:u16)
                n129 = disable-structure shown="Enabled" {
                  disable-tunnel: w291 -> [w304 _]
                  disable-tunnel: w288 -> [w303 _]
                  disable-tunnel: w290 -> [w302 _]
                  disable-tunnel: w286 -> [w301 _]
                  frame Enabled {
                    n130 = property class="DigNum (strict)"(reference=w304, "Val(Sgnl)"=w303) -> ()  [unwired: 1 in, 2 out]
                    n131 = property class="DigNum (strict)"(reference=w302, "Val(Sgnl)"=w301) -> ()  [unwired: 1 in, 2 out]
                  }
                  frame Disabled {
                  }
                }
              }
            }
            n132 = call <vilib>:"Add State(s) to Queue__jki_lib_state_machine.vi"("State(s) in (\"\")"=w285) -> ("States Out"=w284:string)  [unwired: 14 in]
          }
          event "Feedback Global": Value Change {
            # "Exit Button Value Change (pressed) Event\n(this executes Macro: Exit to terminate the VI)"
            n133 = event-data() -> ("NewVal"=w307:bool)  [unwired: 1 in, 5 out]
            n134 = call <vilib>:"Add State(s) to Queue__jki_lib_state_machine.vi"("State(s) in (\"\")"=w310) -> ("States Out"=w309:string)  [unwired: 14 in]
            n135 = Bundle By Name(cluster=w306, "Feedback global"=w307) -> (w305:T34)
          }
          event Value Change {
            n136 = event-data() -> ()  [unwired: 1 in, 6 out]
            n137 = call <vilib>:"Add State(s) to Queue__jki_lib_state_machine.vi"("State(s) in Front (\"\")"="Move Config", "State(s) in (\"\")"=w315) -> ("States Out"=w314:string)  [unwired: 13 in]
          }
          event Value Change {
            n138 = event-data() -> ()  [unwired: 1 in, 6 out]
            n139 = call <vilib>:"Add State(s) to Queue__jki_lib_state_machine.vi"("State(s) in Front (\"\")"="Detection Config", "State(s) in (\"\")"=w320) -> ("States Out"=w319:string)  [unwired: 13 in]
          }
          event "associated motors X": Value Change {
            n140 = event-data() -> ()  [unwired: 1 in, 6 out]
            n141 = call <vilib>:"Add State(s) to Queue__jki_lib_state_machine.vi"("State(s) in (\"\")"=w325, "State(s) at Back (\"\")"="Motor Config" ("State(s) at Back (\"\")")) -> ("States Out"=w324:string)  [unwired: 13 in]
          }
          event "Reset History": Value Change {
            n142 = event-data() -> ()  [unwired: 1 in, 6 out]
            n143 = call <vilib>:"Add State(s) to Queue__jki_lib_state_machine.vi"("State(s) in (\"\")"=w331, "State(s) at Back (\"\")"="Reset History" ("State(s) at Back (\"\")")) -> ("States Out"=w330:string)  [unwired: 13 in]
            n144 = property on="Reset History" class="Bool (strict)"("Value"=FALSE ("Reset History")) -> ()  [unwired: 2 in, 2 out]
          }
          event "Save Config": Value Change {
            n145 = event-data() -> ()  [unwired: 1 in, 6 out]
            n146 = call <vilib>:"Add State(s) to Queue__jki_lib_state_machine.vi"("State(s) in (\"\")"=w336, "State(s) at Back (\"\")"="Save Config" ("State(s) at Back (\"\")")) -> ("States Out"=w335:string)  [unwired: 13 in]
          }
          event "Load Config": Value Change {
            n147 = event-data() -> ()  [unwired: 1 in, 6 out]
            n148 = call "File Dialog2"("pattern (all files)"="*.cfg", "pattern label"="config") -> ("selected path"=w340:path)  [unwired: 10 in, 3 out]
            n149 = Path To String(path=w340) -> (string=w338:string)
            "config path" <- w338
            n150 = call <vilib>:"Build State String with Arguments__jki_lib_state_machine.vi"("Arguments (\"\")"=w338, "State"="Load Config" ("State(s) at Back (\"\")")) -> ("State with Arguments"=w337:string)  [unwired: 4 in]
            n151 = call <vilib>:"Add State(s) to Queue__jki_lib_state_machine.vi"("State(s) in (\"\")"=w346, "State(s) at Back (\"\")"=w337) -> ("States Out"=w345:string)  [unwired: 13 in]
          }
          event "Save Stats": Value Change {
            n152 = event-data() -> ()  [unwired: 1 in, 6 out]
            n153 = call <vilib>:"Add State(s) to Queue__jki_lib_state_machine.vi"("State(s) in (\"\")"=w351, "State(s) at Back (\"\")"="Save Stats" ("State(s) at Back (\"\")")) -> ("States Out"=w350:string)  [unwired: 13 in]
          }
          event "Tab Cams": Value Change {
            n154 = event-data() -> ()  [unwired: 1 in, 6 out]
            n155 = call <vilib>:"Add State(s) to Queue__jki_lib_state_machine.vi"("State(s) in (\"\")"=w353, "State(s) at Back (\"\")"="stats" ("State")) -> ("States Out"=w352:string)  [unwired: 13 in]
          }
          event "active CCDs": Value Change {
            n156 = event-data() -> ("NewVal"=w362:i32)  [unwired: 1 in, 5 out]
            n157 = Unbundle By Name(w358) -> ("active cams"=w357:string[])
            n158 = Index Array(array=w357, index=w362) -> (element=w360:string)
            n159 = call <vilib>:"Build State String with Arguments__jki_lib_state_machine.vi"("Arguments (\"\")"=w360, "State"="active" ("State(s) at Back (\"\")")) -> ("State with Arguments"=w359:string)  [unwired: 4 in]
            n160 = call <vilib>:"Add State(s) to Queue__jki_lib_state_machine.vi"("State(s) in (\"\")"=w365, "State(s) at Back (\"\")"=w359) -> ("States Out"=w364:string)  [unwired: 13 in]
          }
          event "Left", "Right": Value Change {
            n161 = event-data() -> ("CtlRef"=w374:refnum<vi>)  [unwired: 1 in, 5 out]
            n162 = property class="Bool (strict)"(reference=w374, error in=w371) -> (reference out=w373:refnum<vi>, error out=w372:errorcluster, "Label.Text"=w368:string)
            n163 = property class="Bool (strict)"(reference=w373, error in=w372, "Value"=FALSE) -> (error out=w370:errorcluster)  [unwired: 1 out]
            n164 = call <vilib>:"Build State String with Arguments__jki_lib_state_machine.vi"("Arguments (\"\")"=w368, "State"="ManMove X") -> ("State with Arguments"=w367:string)  [unwired: 4 in]
            n165 = call <vilib>:"Add State(s) to Queue__jki_lib_state_machine.vi"("State(s) in (\"\")"=w377, "State(s) at Back (\"\")"=w367) -> ("States Out"=w376:string)  [unwired: 13 in]
          }
          event "Up", "Down": Value Change {
            n166 = event-data() -> ("CtlRef"=w386:refnum<vi>)  [unwired: 1 in, 5 out]
            n167 = property class="Bool (strict)"(reference=w386, error in=w383) -> (reference out=w385:refnum<vi>, error out=w384:errorcluster, "Label.Text"=w380:string)
            n168 = property class="Bool (strict)"(reference=w385, error in=w384, "Value"=FALSE) -> (error out=w382:errorcluster)  [unwired: 1 out]
            n169 = call <vilib>:"Build State String with Arguments__jki_lib_state_machine.vi"("Arguments (\"\")"=w380, "State"="ManMove Y") -> ("State with Arguments"=w379:string)  [unwired: 4 in]
            n170 = call <vilib>:"Add State(s) to Queue__jki_lib_state_machine.vi"("State(s) in (\"\")"=w389, "State(s) at Back (\"\")"=w379) -> ("States Out"=w388:string)  [unwired: 13 in]
          }
          event "Center": Value Change {
            n171 = event-data() -> ()  [unwired: 1 in, 6 out]
            n172 = call <vilib>:"Add State(s) to Queue__jki_lib_state_machine.vi"("State(s) in (\"\")"=w394, "State(s) at Back (\"\")"="Center" ("State(s) at Back (\"\")")) -> ("States Out"=w393:string)  [unwired: 13 in]
          }
          event "new tdms": Value Change {
            n173 = event-data() -> ()  [unwired: 1 in, 6 out]
            n174 = call <vilib>:"Add State(s) to Queue__jki_lib_state_machine.vi"("State(s) in (\"\")"=w399, "State(s) at Back (\"\")"="newtdms" ("State(s) at Back (\"\")")) -> ("States Out"=w398:string)  [unwired: 13 in]
          }
          event "device ini": Value Change {
            n175 = event-data() -> ()  [unwired: 1 in, 6 out]
            n176 = property on="device ini" class="Bool (strict)"("Value"=FALSE ("test")) -> ()  [unwired: 2 in, 2 out]
            n177 = call <vilib>:"Add State(s) to Queue__jki_lib_state_machine.vi"("State(s) in (\"\")"=w405, "State(s) at Back (\"\")"="Device Ini" ("State(s) at Back (\"\")")) -> ("States Out"=w404:string)  [unwired: 13 in]
          }
          event "img to avg": Value Change {
            n178 = event-data() -> ("NewVal"=w411:i32)  [unwired: 1 in, 5 out]
            n179 = Number To Decimal String(number=w411) -> (decimal integer string=w413:string)  [unwired: 1 in]
            n180 = call <vilib>:"Build State String with Arguments__jki_lib_state_machine.vi"("Arguments (\"\")"=w413, "State"="ImgToAvg" ("State(s) at Back (\"\")")) -> ("State with Arguments"=w406:string)  [unwired: 4 in]
            n181 = call <vilib>:"Add State(s) to Queue__jki_lib_state_machine.vi"("State(s) in Front (\"\")"=w406, "State(s) in (\"\")"=w409) -> ("States Out"=w408:string)  [unwired: 13 in]
          }
          event Panel Close? {
            # "Discard the event because we'll close the front panel ourselves in Macro: Exit"
            # "Close Panel button (pressed) Event\n(this executes Macro: Exit to terminate the VI)"
            n182 = event-data() -> ()  [unwired: 1 in, 1 out]
            n183 = call <vilib>:"Add State(s) to Queue__jki_lib_state_machine.vi"("State(s) in Front (\"\")"="Macro: Exit", "State(s) in (\"\")"=w419) -> ("States Out"=w418:string)  [unwired: 13 in]
            n184 = event-data("Discard?"=TRUE) -> ()  [unwired: 1 in, 1 out]
          }
        }
      }
      frame "---------- Core ----------" {
        # "Do not put any code in this frame.\n(it is a separator no-op)"
        n185 = call <vilib>:"Add State(s) to Queue__jki_lib_state_machine.vi"("State(s) in (\"\")"=w423) -> ("States Out"=w422:string)  [unwired: 14 in]
      }
      frame Default {
        w433 = 42 items=["No error", "Argument error", "Memory is full", "Out of zone", "End of file", "File already open", "Generic file I/O error", "File not found", "File permission error", "Disk is full", "Duplicate path", "Too many files open", "System feature not enabled", "Resource file not found", "Cannot add resource", "Resource not found", "Image not found", "Image memory error", "Pen does not exist", "Config type invalid", "Config token not found", "Config parse error", "Config memory error", "Bad external code format", "Bad external code offset", "External code not present", "Null window", "Destroy window error", "Null menu", "Print aborted", "Bad print record", "Print driver error", "Windows error during printing", "Memory error during printing", "Print dialog error", "Generic print error", "Invalid device refnum", "Device not found", "Device parameter error", "Device unit error", "Cannot open device", "Device call aborted", "Generic error", "Cancelled by user", "Object ID too low", "Object ID too high", "Object not in heap", "Unknown heap", "Unknown object (invalid DefProc)", "Unknown object (DefProc not in table)", "Message out of range", "Invalid (null) method", "Unknown message", "Manager call not supported", "Bad address", "Network operation in progress", "Network operation timed out", "Connection is busy", "Network attribute not supported", "Network error", "Address in use", "System out of memory", "Connection aborted", "Connection refused", "Not connected", "Already connected", "Connection closed", "Initialization error (interapplication manager)", "Bad occurrence", "Wait on unbound occurrence handler", "Occurrence queue overflow", "Datalog type conflict", "Unused", "Unrecognized type (interapplication manager)", "Memory corrupt", "Failed to make temporary DLL", "Old CIN version", "Drag socket not found", "Failed to load drop-object", "Failed to register OLE object", "Failed to release OLE object", "Format specifier type mismatch", "Unknown format specifier", "Too few format specifiers", "Too many format specifiers", "Scan failed", "Newer CIN version", "Error converting to variant", "Runtime menu error", "Password tampered", "Variant attribute not found", "Incompatible variant data type", "Event data is not available", "Event Store is not present", "Occurrence is not found", "Event Queue is not created", "Event info is not available", "Refnum passed is NULL", "Error retrieving Class GUID", "Error retrieving CoClass GUID", "Error retrieving TypeLib GUID.", "Bad built application magic bytes.", "Specific driver is different from the specific driver associated with the Logical Name.", "There is no session opened to the class driver.", "Max Error", "MAX - Error with config objects", "MAX - Error loading configuration", "MAX - Group not supported"]
        # "Current State"
        # "Do not delete, rename, or modify this frame.\n(this is used to capture unhandled states and typos)"
        # "Handle mistyped state name (developer tool)"
        n186 = Format Into String(format string="Software Exception: Unhandled State \"%s\"." ("message"), error in=w429, w424) -> (resulting string=w432:string, error out=w431:errorcluster)  [unwired: 1 in]
        n187 = call <vilib>:"Error Cluster From Error Code.vi"("show call chain? (False)"=TRUE, "error in (no error)"=w431, "error message (\"\")"=w432, "error code (0)"=w433) -> ("error out"=w430:errorcluster)  [unwired: 5 in]
        n188 = call <vilib>:"Add State(s) to Queue__jki_lib_state_machine.vi"("State(s) in (\"\")"=w428) -> ("States Out"=w427:string)  [unwired: 14 in]
      }
      frame "Initialize Core Data" {
        # "Do not delete, rename, or modify this frame.\n(this is used to determine panel behavior on exit)"
        # "originally closed?"
        # "exe?"
        # "If panel starts closed or is an EXE, then close it when we exit"
        n189 = property class="VI"() -> ("Front Panel.Open"=w443:bool)  [unwired: 2 in, 2 out]
        n190 = property class="App"() -> ("App.Kind"=w442:T25)  [unwired: 2 in, 2 out]
        n191 = control-ref of="Current VI Reference"() -> (w437:refnum<vi>)
        n192 = Not(x=w443) -> (.not. x?=w440:bool)
        n193 = Equal?(x=w442, y=T25."Run Time System" ("Application:Kind")) -> (x = y?=w439:bool)
        n194 = Or(x=w440, y=w439) -> (x .or. y?=w438:bool)
        n195 = Bundle By Name(cluster=w436, "Core.Current VI Reference"=w437, "Core.Close Panel on Exit?"=w438) -> (w435:T34)
        n196 = call <vilib>:"Add State(s) to Queue__jki_lib_state_machine.vi"("State(s) in (\"\")"=w446) -> ("States Out"=w445:string)  [unwired: 14 in]
      }
      frame "Error Handler" {
        # "Unhandled Error -- Display it"
        # "Handle any errors here.\nYou can also output any states to clean-up after errors occur"
        # "Clear error"
        n197 = call <vilib>:"General Error Handler.vi"("error in (no error)"=w448) -> ()  [unwired: 10 in, 5 out]
        n198 = call <vilib>:"Add State(s) to Queue__jki_lib_state_machine.vi"("State(s) in Front (\"\")"="/* Post Error States", "State(s) in (\"\")"=w452) -> ("States Out"=w451:string)  [unwired: 13 in]
      }
      frame "Exit" {
        # "Do not put any code in this frame.\n(No errors that occur here will be handled.)"
        n199 = call <vilib>:"Add State(s) to Queue__jki_lib_state_machine.vi"("State(s) in (\"\")"=w457) -> ("States Out"=w456:string)  [unwired: 14 in]
      }
      frame "---------- Data ----------" {
        # "Do not put any code in this frame.\n(It is a separator no-op. You can make a copy of this frame to create a new Data frame)"
        n200 = call <vilib>:"Add State(s) to Queue__jki_lib_state_machine.vi"("State(s) in (\"\")"=w461) -> ("States Out"=w460:string)  [unwired: 14 in]
      }
      frame "Data: Initialize" {
        w462 = T35 {"STOP queue"=refnum, "SuperGUI ref"=refnum}  # Supergui
        w463 = dbl[] [0.0, 0.0, 0.0, 0.0, 0.0, 0.0, 0.0, 0.0, 0.0, 0.0, 0.0, 0.0]  # steps speed Y
        w464 = dbl[] [0.0, 0.0, 0.0, 0.0, 0.0, 0.0, 0.0, 0.0, 0.0, 0.0, 0.0, 0.0]  # steps speed X
        w468 = bool[] [FALSE, FALSE, FALSE, FALSE, TRUE, TRUE, TRUE, FALSE, FALSE, FALSE, FALSE, FALSE]  # detected
        w478 = bool[] [FALSE, FALSE, FALSE, FALSE, FALSE, FALSE, FALSE, FALSE, FALSE, FALSE, FALSE, TRUE]  # speedmode Y
        w479 = bool[] [FALSE, FALSE, FALSE, FALSE, FALSE, FALSE, FALSE, FALSE, FALSE, FALSE, FALSE, TRUE]  # speedmode X
        w481 = cluster{"Lower value":sgl, "Upper value":sgl}[] [{"Lower value"=93.0, "Upper value"=255.0}, {"Lower value"=105.0, "Upper value"=255.0}, {"Lower value"=0.0, "Upper value"=255.0}, {"Lower value"=127.0, "Upper value"=255.0}, {"Lower value"=0.0, "Upper value"=255.0}, {"Lower value"=0.0, "Upper value"=255.0}, {"Lower value"=0.0, "Upper value"=255.0}, {"Lower value"=0.0, "Upper value"=255.0}, {"Lower value"=0.0, "Upper value"=255.0}, {"Lower value"=0.0, "Upper value"=255.0}, {"Lower value"=0.0, "Upper value"=255.0}, {"Lower value"=0.0, "Upper value"=255.0}]  # thresholds
        w488 = FALSE  # Feedback global
        w490 = 0  # active ccd
        w474 = 6  # img to avg
        w501 = T36 {"Current VI Reference"=refnum, "Close Panel on Exit?"=FALSE}  # Core
        # "Initialize the shift-register data, here.\n(data names are defined by what you wire into the bundle function)"
        n201 = disable-structure shown="Disabled" {
          disable-tunnel: w471 -> [w513 _]
          disable-tunnel: [w512 _] -> w470
          disable-tunnel: w469 -> [w511 _]
          disable-tunnel: [w510 _] -> _
          disable-tunnel: w467 -> [w504 _]
          frame Disabled {
            n202 = TDMS Open(6:FALSE ("disable buffering (T)"), 7:enum16{"1.0", "2.0"}."2.0" ("file format version (2.0)"), 8:w513, 10:T26."create or replace" ("operation"), 11:w511) -> (0:w508:errorcluster, 3:w509:refnum<k34>)  [unwired: 2 in]
            n203 = call "TDMSbuffersize.vi"("error in (no error)"=w508, "group names"=w504, "Data Value Reference in"=w509) -> ("error out"=w512:errorcluster, "Data Value Reference out"=w510:refnum<k34>)  [unwired: 7 in]
          }
          frame Enabled {
          }
        }
        n204 = call <vilib>:"Add State(s) to Queue__jki_lib_state_machine.vi"("State(s) in Front (\"\")"="newtdms" ("State(s) in Front (\"\")"), "State(s) in (\"\")"=w503) -> ("States Out"=w502:string)  [unwired: 13 in]
        n205 = Bundle("Core"=w501, "detection para"="detection para", "thresholds"=w481, "Centroid X"="Centroid X", "Centroid Y"="Centroid Y", "img to avg"=w474, "Mean Centroid X"="Mean Centroid X", "Mean Centroid Y"="Mean Centroid Y", "Offset X"="Offset X", "Offset Y"="Offset Y", "Offset X stats"="Offset X stats", "Offset Y stats"="Offset Y stats", "Size"="Size", "Mean Size"="Mean Size", "Time"="Time", "move properties"="move properties", "active axis refs 2"="active axis refs 2", "active ccd"=w490, "Feedback global"=w488, "Motor X"="Motor X", "Motor Y"="Motor Y", "active cams"="active cams", "Data Value Reference out"=refnum<k34> refnum, "active man refs"="active man refs", "detected"=w468, "speedmode X"=w479, "speedmode Y"=w478, "steps speed X"=w464, "steps speed Y"=w463, "Supergui"=w462) -> (w473:T34)  [unwired: 1 in]
        n206 = Initialize Array(0.0 ("element"), 12 ("dimension size"), w474) -> (w477:dbl[][])
        n207 = Bundle By Name(cluster=w473, "Centroid X"=w477, "Centroid Y"=w477, "Size"=w477) -> (w472:T34)
      }
      frame "Data: Cleanup" {
        # "Cleanup any data and references, here.\n(this is called automatically, by the Macro: Exit)"
        n208 = Unbundle By Name(w514) -> ("Core.Current VI Reference"=w515:refnum<vi>)
        n209 = Close Reference(reference=w515, error in (no error)=w517) -> (error out=w516:errorcluster)
        n210 = call <vilib>:"Add State(s) to Queue__jki_lib_state_machine.vi"("State(s) in (\"\")"=w519) -> ("States Out"=w518:string)  [unwired: 14 in]
      }
      frame "StopSuperGUI" {
        # "Initialize the User Interface, here.\n(this is called automatically, by the Macro: Init)"
        n211 = Unbundle By Name(w522) -> ("Supergui.SuperGUI ref"=w524:refnum<vi>, "Supergui.STOP queue"=w525:refnum<queue>)
        n212 = Release Queue(queue=w525, error in (no error)=w521) -> (error out=w523:errorcluster)  [unwired: 1 in, 2 out]
        n213 = call <vilib>:"Add State(s) to Queue__jki_lib_state_machine.vi"("State(s) in (\"\")"=w527) -> ("States Out"=w526:string)  [unwired: 14 in]
        n214 = call-by-ref "Wait On Asynchronous Call"(reference=w524, error in=w523) -> ("error out"=w520:errorcluster)  [unwired: 11 in, 2 out]
      }
      frame "---------- UI ----------" {
        # "Do not put any code in this frame.\n(It is a separator no-op. You can make a copy of this frame to create a new UI frame)"
        n215 = call <vilib>:"Add State(s) to Queue__jki_lib_state_machine.vi"("State(s) in (\"\")"=w531) -> ("States Out"=w530:string)  [unwired: 14 in]
      }
      frame "UI: Initialize" {
        # "Initialize the User Interface, here.\n(this is called automatically, by the Macro: Init)"
        n216 = call <vilib>:"Add State(s) to Queue__jki_lib_state_machine.vi"("State(s) in (\"\")"=w535) -> ("States Out"=w534:string)  [unwired: 14 in]
      }
      frame "UI: Cursor Set" {
        # "Argument"
        # "Set and Unset Cursor Busy.\n(Usage: \"UI: Cursor Set >> Busy|Idle\")"
        n217 = case shown="\"Idle\", Default" w536 {
          tunnel: w538 -> [w543 w545]
          tunnel: [w542 w544] -> w537
          frame "Idle", Default {
            n218 = call <vilib>:"Unset Busy.vi"("error in (no error)"=w543) -> ("error out"=w542:errorcluster)  [unwired: 10 in]
          }
          frame "Busy" {
            n219 = call <vilib>:"Set Busy.vi"("error in (no error)"=w545) -> ("error out"=w544:errorcluster)  [unwired: 9 in, 1 out]
          }
        }
        n220 = call <vilib>:"Add State(s) to Queue__jki_lib_state_machine.vi"("State(s) in (\"\")"=w541) -> ("States Out"=w540:string)  [unwired: 14 in]
      }
      frame "UI: Front Panel State" {
        # "Argument"
        # "Set Front Panel Open or Closed\n(Usage: \"UI: Front Panel State >> Open|Close\")"
        n221 = Unbundle By Name(w546) -> ("Core.Current VI Reference"=w548:refnum<vi>)
        n222 = case shown="\"Open\", Default" w547 {
          tunnel: w550 -> [w556 w567]
          tunnel: [w557 w568] -> w549
          tunnel: w548 -> [_ _]
          frame "Open", Default {
            n223 = property class="VI"(error in=w556) -> (reference out=w554:refnum<vi>, error out=w555:errorcluster, "Front Panel.Open"=w553:bool)  [unwired: 1 in]
            n224 = case shown="False" w553 {
              tunnel: [w560 w563] -> w557
              tunnel: w555 -> [w559 w563]
              tunnel: w554 -> [w558 _]
              frame False {
                n225 = invoke class="VI" method="FP.Open"(reference=w558, error in=w559, "Activate"=TRUE, "State"=T27."Standard") -> (error out=w560:errorcluster)  [unwired: 1 in, 4 out]
              }
              frame True {
              }
            }
          }
          frame "Close" {
            n226 = property class="VI"(error in=w567) -> (reference out=w565:refnum<vi>, error out=w566:errorcluster, "Front Panel.Open"=w564:bool)  [unwired: 1 in]
            n227 = case shown="True" w564 {
              tunnel: [w569 w572] -> w568
              tunnel: w566 -> [w569 w571]
              tunnel: w565 -> [_ w570]
              frame False {
              }
              frame True {
                n228 = invoke class="VI" method="FP.Close"(reference=w570, error in=w571) -> (error out=w572:errorcluster)  [unwired: 1 in, 2 out]
              }
            }
          }
        }
        n229 = call <vilib>:"Add State(s) to Queue__jki_lib_state_machine.vi"("State(s) in (\"\")"=w552) -> ("States Out"=w551:string)  [unwired: 14 in]
      }
      frame "---------- Macro ----------" {
        # "Do not put any code in this frame.\n(It is a separator no-op. You can make a copy of this frame to create a new Macro frame)"
        n230 = call <vilib>:"Add State(s) to Queue__jki_lib_state_machine.vi"("State(s) in (\"\")"=w576) -> ("States Out"=w575:string)  [unwired: 14 in]
      }
      frame "Macro: Initialize" {
        # "Initialization Macro\n(This is called once, when the VI starts)"
        n231 = property on="img to avg" class="DigNum (strict)"() -> ("Value"=w578:i32)  [unwired: 2 in, 2 out]
        n232 = Number To Decimal String(number=w578) -> (decimal integer string=w580:string)  [unwired: 1 in]
        n233 = call <vilib>:"Build State String with Arguments__jki_lib_state_machine.vi"("Arguments (\"\")"=w580, "State"="ImgToAvg") -> ("State with Arguments"=w577:string)  [unwired: 4 in]
        n234 = call <vilib>:"Add State(s) to Queue__jki_lib_state_machine.vi"("State(s) in Front (\"\")"="Data: Initialize\nInitialize Core Data\nUI: Initialize\nUI: Front Panel State >> Open\nReadDevicesFile\nMotorRefs\nCameraRefs\nStartSuperGUI\nDevice Ini >> 3000", "State(s) in (\"\")"=w585, "State(s) at Back (\"\")"=w577) -> ("States Out"=w584:string)  [unwired: 12 in]
      }
      frame "Macro: Exit" {
        # "Exit Macro\n(This is called once, when the VI exits)"
        n235 = Unbundle By Name(w588) -> ("Core.Close Panel on Exit?"=w587:bool)
        n236 = Select(t="UI: Front Panel State >> Close", s=w587, f="") -> (s? t:f=w591:string)
        n237 = call <vilib>:"Add State(s) to Queue__jki_lib_state_machine.vi"("State(s) in Front (\"\")"="StopSuperGUI" ("State(s) in Front (\"\")"), "State(s) in (\"\")"=w591, "State(s) at Back (\"\")"="Data: Cleanup\nExit") -> ("States Out"=w589:string)  [unwired: 12 in]
        n238 = call <vilib>:"Add State(s) to Queue__jki_lib_state_machine.vi"("State(s) in Front (\"\")"=w589, "State(s) in (\"\")"=w596) -> ("States Out"=w595:string)  [unwired: 13 in]
      }
      frame "---------- Ini and Configure ----------" {
        # "Template Separator\n(You can make a copy of, or modify, this frame)"
        n239 = call <vilib>:"Add State(s) to Queue__jki_lib_state_machine.vi"("State(s) in (\"\")"=w600) -> ("States Out"=w599:string)  [unwired: 14 in]
      }
      frame "ReadDevicesFile" {
        # "Initialize the User Interface, here.\n(this is called automatically, by the Macro: Init)"
        n240 = call <vilib>:"Application Directory.vi"() -> ("Application Directory"=w604:path)
        n241 = call "File Dialog3"("start path"=w604, "default name"="defaultDevices_ BELLA_BTL.txt", "pattern (all files)"="*.txt") -> ("selected path"=w601:path)  [unwired: 9 in, 3 out]
        "appended path" <- w601
        n242 = Build Path(base path=w604, name or relative path="defaultDevices_ BELLA_BTL.txt") -> ()  [unwired: 1 out]
        n243 = call-poly <vilib>:"Read From Spreadsheet File.vi"("file path (dialog if empty)"=w601) -> ("all rows"=w633:string[][])  [unwired: 6 in, 4 out]
        n244 = Index Array(array=w633, index (col) #1=0 ("disabled index (col)"), index (col) #2=1 ("index (col)")) -> (element #1=w632:string[])  [unwired: 2 in, 1 out]
        n245 = call <vilib>:"Add State(s) to Queue__jki_lib_state_machine.vi"("State(s) in (\"\")"=w637) -> ("States Out"=w636:string)  [unwired: 14 in]
        n246 = Index Array(array=w632, index #1=0 ("index"), index #2=1 ("index"), index #3=2 ("index"), index #4=3 ("index"), index #5=4 ("index"), index #6=5 ("index"), index #7=6 ("index"), index #8=7 ("index"), index #9=8 ("index"), index #10=9 ("index"), index #11=10 ("index"), index #12=11 ("index")) -> (element #1=w631:string, element #2=w630:string, element #3=w629:string, element #4=w628:string, element #5=w627:string, element #6=w626:string, element #7=w625:string, element #8=w624:string, element #9=w623:string, element #10=w622:string, element #11=w621:string, element #12=w620:string)
        n247 = property on="GUIdevice 1" class="Str"("Val(Sgnl)"=w631) -> ()  [unwired: 2 in, 2 out]
        n248 = property on="GUIdevice 2" class="Str"("Val(Sgnl)"=w630) -> ()  [unwired: 2 in, 2 out]
        n249 = property on="GUIdevice 3" class="Str"("Val(Sgnl)"=w629) -> ()  [unwired: 2 in, 2 out]
        n250 = property on="GUIdevice 4" class="Str"("Val(Sgnl)"=w628) -> ()  [unwired: 2 in, 2 out]
        n251 = property on="GUIdevice 5" class="Str"("Val(Sgnl)"=w627) -> ()  [unwired: 2 in, 2 out]
        n252 = property on="GUIdevice 6" class="Str"("Val(Sgnl)"=w626) -> ()  [unwired: 2 in, 2 out]
        n253 = property on="GUIdevice 7" class="Str"("Val(Sgnl)"=w625) -> ()  [unwired: 2 in, 2 out]
        n254 = property on="GUIdevice 8" class="Str"("Val(Sgnl)"=w624) -> ()  [unwired: 2 in, 2 out]
        n255 = property on="GUIdevice 9" class="Str"("Val(Sgnl)"=w623) -> ()  [unwired: 2 in, 2 out]
        n256 = property on="GUIdevice 10" class="Str"("Val(Sgnl)"=w622) -> ()  [unwired: 2 in, 2 out]
        n257 = property on="GUIdevice 11" class="Str"("Val(Sgnl)"=w621) -> ()  [unwired: 2 in, 2 out]
        n258 = property on="GUIdevice 12" class="Str"("Val(Sgnl)"=w620) -> ()  [unwired: 2 in, 2 out]
      }
      frame "MotorRefs" {
        # "#todo can use get all aliases to fill in motor names, and use\nudp directly to set and get values, rather than super gui"
        n259 = Build Array("GUIdevice 99", "GUIdevice 98", "GUIdevice 97") -> (w649:string[])
        n260 = for {
          tunnel: w649 -> [w664] mode=indexing
          tunnel: [w663] -> w654 mode=concatenating
          n261 = for {
            tunnel: w664 -> [w670]
            tunnel: string[] ["Position.Axis 1", "Position.Axis 2", "Position.Axis 3"] ("elements") -> [w669] mode=indexing
            tunnel: [w666] -> w663 mode=indexing
            n262 = call "preset SQL Queries.vi"("Expt name / MCIP/ Variable/Preset Name"=w669, "Device/Devicetype name\n/Plotter.id/ScanName#"=w670, "Preset Query"=Preset_Query_Enum."Get device variable aliases") -> ("1st column 1st data"=w667:string[])  [unwired: 6 in, 2 out]
            n263 = Index Array(array=w667) -> (element=w666:string)  [unwired: 1 in]
          }
        }
        "Names" <- w654
        n264 = control-ref of="Position.Axis 1::99"() -> (w639:refnum<vi>)
        n265 = control-ref of="Position.Axis 2::99"() -> (w640:refnum<vi>)
        n266 = control-ref of="Position.Axis 3::99"() -> (w650:refnum<vi>)
        n267 = control-ref of="Position.Axis 1::98"() -> (w642:refnum<vi>)
        n268 = control-ref of="Position.Axis 2::98"() -> (w643:refnum<vi>)
        n269 = control-ref of="Position.Axis 3::98"() -> (w644:refnum<vi>)
        n270 = control-ref of="Position.Axis 1::97"() -> (w645:refnum<vi>)
        n271 = control-ref of="Position.Axis 2::97"() -> (w646:refnum<vi>)
        n272 = control-ref of="Position.Axis 3::97"() -> (w647:refnum<vi>)
        n273 = property on="associated motors Y" class="Clust (strict)"() -> ("Controls[]"=w653:refnum<vi>[])  [unwired: 2 in, 2 out]
        n274 = for {
          tunnel: w653 -> [w662] mode=indexing
          tunnel: refnum<vi> refnum ("Motor CCD 1") -> [w661]
          tunnel: w654 -> [w659]
          n275 = To More Specific Class(target class=w661, reference=w662) -> (specific class reference=w660:refnum<vi>)  [unwired: 1 in, 1 out]
          n276 = property on="Property Node" class="Ring (strict)"(reference=w660, "Strings []"=w659) -> ()  [unwired: 1 in, 2 out]
        }
        n277 = Build Array(w639, w640, w650, w642, w643, w644, w645, w646, w647) -> (→"motor refs":refnum<vi>[])
        n278 = call <vilib>:"Add State(s) to Queue__jki_lib_state_machine.vi"("State(s) in (\"\")"=w658) -> ("States Out"=w657:string)  [unwired: 14 in]
        n279 = property on="Motor CCD 1" class="Ring (strict)"("Strings []"=w654) -> ()  [unwired: 2 in, 2 out]
        n280 = property on="Motor CCD 2" class="Ring (strict)"("Strings []"=w654) -> ()  [unwired: 2 in, 2 out]
        n281 = property on="Motor CCD 3" class="Ring (strict)"("Strings []"=w654) -> ()  [unwired: 2 in, 2 out]
        n282 = property on="Motor CCD 4" class="Ring (strict)"("Strings []"=w654) -> ()  [unwired: 2 in, 2 out]
        n283 = property on="Motor CCD 5" class="Ring (strict)"("Strings []"=w654) -> ()  [unwired: 2 in, 2 out]
        n284 = property on="Motor CCD 6" class="Ring (strict)"("Strings []"=w654) -> ()  [unwired: 2 in, 2 out]
        n285 = property on="Motor CCD 7" class="Ring (strict)"("Strings []"=w654) -> ()  [unwired: 2 in, 2 out]
        n286 = property on="Motor CCD 8" class="Ring (strict)"("Strings []"=w654) -> ()  [unwired: 2 in, 2 out]
        n287 = property on="Motor CCD 9" class="Ring (strict)"("Strings []"=w654) -> ()  [unwired: 2 in, 2 out]
        n288 = property on="Motor CCD 10" class="Ring (strict)"("Strings []"=w654) -> ()  [unwired: 2 in, 2 out]
        n289 = property on="Motor CCD 11" class="Ring (strict)"("Strings []"=w654) -> ()  [unwired: 2 in, 2 out]
        n290 = property on="Motor CCD 12" class="Ring (strict)"("Strings []"=w654) -> ()  [unwired: 2 in, 2 out]
      }
      frame "CameraRefs" {
        w671 = T37 0 items=["Grayscale (U8)", "Grayscale (I16)", "Grayscale (SGL)", "Complex (CSG)", "RGB (U32)", "HSL (U32)", "RGB (U64)", "Grayscale (U16)"] ("Image Type")
        n291 = property on="image::5" class="ImageControl"("Caption.Text"="GUIdevice 5") -> ()  [unwired: 2 in, 2 out]
        n292 = property on="image::7" class="ImageControl"("Caption.Text"="GUIdevice 7") -> ()  [unwired: 2 in, 2 out]
        n293 = property on="image::6" class="ImageControl"("Caption.Text"="GUIdevice 6") -> ()  [unwired: 2 in, 2 out]
        n294 = property on="image::9" class="ImageControl"("Caption.Text"="GUIdevice 9") -> ()  [unwired: 2 in, 2 out]
        n295 = property on="image::1" class="ImageControl"("Caption.Text"="GUIdevice 1") -> ()  [unwired: 2 in, 2 out]
        n296 = property on="image::10" class="ImageControl"("Caption.Text"="GUIdevice 10") -> ()  [unwired: 2 in, 2 out]
        n297 = property on="image::8" class="ImageControl"("Caption.Text"="GUIdevice 8") -> ()  [unwired: 2 in, 2 out]
        n298 = property on="image::2" class="ImageControl"("Caption.Text"="GUIdevice 2") -> ()  [unwired: 2 in, 2 out]
        n299 = property on="image::4" class="ImageControl"("Caption.Text"="GUIdevice 4") -> ()  [unwired: 2 in, 2 out]
        n300 = property on="image::3" class="ImageControl"("Caption.Text"="GUIdevice 3") -> ()  [unwired: 2 in, 2 out]
        n301 = property on="image::11" class="ImageControl"("Caption.Text"="GUIdevice 11") -> ()  [unwired: 2 in, 2 out]
        n302 = property on="image::12" class="ImageControl"("Caption.Text"="GUIdevice 12") -> ()  [unwired: 2 in, 2 out]
        n303 = call "IMAQ Create"("Image Name"="GUIdevice 8", "Image Type"=w671) -> ("New Image"=→"image::8":T6)  [unwired: 3 in, 1 out]
        n304 = call "IMAQ Create"("Image Name"="GUIdevice 9", "Image Type"=w671) -> ("New Image"=→"image::9":T6)  [unwired: 3 in, 1 out]
        n305 = call "IMAQ Create"("Image Name"="GUIdevice 10", "Image Type"=w671) -> ("New Image"=→"image::10":T6)  [unwired: 3 in, 1 out]
        n306 = call "IMAQ Create"("Image Name"="GUIdevice 6", "Image Type"=w671) -> ("New Image"=→"image::6":T6)  [unwired: 3 in, 1 out]
        n307 = call "IMAQ Create"("Image Name"="GUIdevice 7", "Image Type"=w671) -> ("New Image"=→"image::7":T6)  [unwired: 3 in, 1 out]
        n308 = call "IMAQ Create"("Image Name"="GUIdevice 11", "Image Type"=w671) -> ("New Image"=→"image::11":T6)  [unwired: 3 in, 1 out]
        n309 = call "IMAQ Create"("Image Name"="GUIdevice 12", "Image Type"=w671) -> ("New Image"=→"image::12":T6)  [unwired: 3 in, 1 out]
        n310 = call "IMAQ Create"("Image Name"="GUIdevice 2") -> ("New Image"=→"image::2":T6)  [unwired: 4 in, 1 out]
        n311 = call "IMAQ Create"("Image Name"="GUIdevice 4", "Image Type"=w671) -> ("New Image"=→"image::4":T6)  [unwired: 3 in, 1 out]
        n312 = call "IMAQ Create"("Image Name"="GUIdevice 1", "Image Type"=w671) -> ("New Image"=→"image::1":T6)  [unwired: 3 in, 1 out]
        n313 = call "IMAQ Create"("Image Name"="GUIdevice 3", "Image Type"=w671) -> ("New Image"=→"image::3":T6)  [unwired: 3 in, 1 out]
        n314 = call "IMAQ Create"("Image Name"="GUIdevice 5", "Image Type"=w671) -> ("New Image"=→"image::5":T6)  [unwired: 3 in, 1 out]
        n315 = Build Array("GUIdevice 1", "GUIdevice 2", "GUIdevice 3", "GUIdevice 4", "GUIdevice 5", "GUIdevice 6", "GUIdevice 7", "GUIdevice 8", "GUIdevice 9", "GUIdevice 10", "GUIdevice 11", "GUIdevice 12") -> (w689:string[])
        "CCDs" <- w689
        n316 = Array To Cluster(array=w689) -> (cluster=→"Cameras":T38)
        n317 = property on="CCDs" class="Ring (strict)"("Strings []"=w689) -> ()  [unwired: 2 in, 2 out]
        n318 = call <vilib>:"Add State(s) to Queue__jki_lib_state_machine.vi"("State(s) in (\"\")"=w701) -> ("States Out"=w700:string)  [unwired: 14 in]
      }
      frame "StartSuperGUI" {
        # "create stop queue for supergui and its clones"
        # "can make an icon"
        # "x100 abort will be dependent on caller VI\nx80 abort will be independent of caller vi, this will abort vi when labview is closed."
        # "Initialize the User Interface, here.\n(this is called automatically, by the Macro: Init)"
        n319 = vi-ref "GUI_Master_subvi_reentrant_queues.vi"() -> (w709:refnum<vi>)
        n320 = call "supergui create stop queue.vi"() -> ("STOP Queue out"=w710:refnum<queue>)  [unwired: 11 in]
        n321 = control-ref of="This Application"() -> (w713:refnum<vi>)
        n322 = property class="VI"(reference=w709) -> ("Path"=w708:path)  [unwired: 1 in, 2 out]
        n323 = control-ref of="This VI"() -> (w712:refnum<vi>)
        n324 = Create User Event(user event datatype=T29 {"EventEnum"=enum."new data", "Device name"="Device name"} ("New Event"), error in=w704) -> (user event=w714:refnum<user-event>, error out=w715:errorcluster)
        "tcp data event 2" <- w714
        n325 = Current VI's Menubar() -> (w711:refnum<k9>)
        n326 = register-events(w714) -> ()  [unwired: 2 in, 2 out]
        n327 = Open VI Reference(type specifier VI Refnum (for type only)=refnum<vi> refnum, vi path=w708, options=256, error in (no error)=w704) -> (vi reference=w719:refnum<vi>, error out=w718:errorcluster)  [unwired: 2 in]
        n328 = call <vilib>:"Add State(s) to Queue__jki_lib_state_machine.vi"("State(s) in (\"\")"=w721) -> ("States Out"=w720:string)  [unwired: 14 in]
        n329 = call-by-ref "Start Asynchronous Call"(reference=w719, error in=w718, "STOP Queue in"=w710, "This Application"=w713, 8:"error in (no error)"=w715, "tcp data event"=w714, "Caller menu reference"=w711, "Caller VI ref"=w712) -> (reference out=w707:refnum<vi>, error out=w703:errorcluster)  [unwired: 5 in, 1 out]
        n330 = Bundle By Name(cluster=w706, "Supergui.SuperGUI ref"=w707, "Supergui.STOP queue"=w710) -> (w705:T34)
      }
      frame "Device Ini" {
        # "Your code here.\n(You can make a copy of, or modify, this frame)"
        n331 = Empty String/Path?(string/path=w725) -> (empty?=w742:bool)
        n332 = case shown="False" w742 {
          tunnel: w725 -> [w784 _]
          tunnel: [w783 0] -> w741
          frame False {
            n333 = Decimal String To Number(string=w784) -> (number=w783:i32)  [unwired: 2 in, 1 out]
          }
          frame True {
          }
        }
        n334 = flat-sequence {
          tunnel: w748 -> [w787]
          tunnel: [w787] -> w747
          tunnel: w741 -> [w786]
          tunnel: w747 -> [w793]
          tunnel: [w791] -> w728
          tunnel: [w790] -> _
          frame #0 {
            n335 = Wait (ms)(milliseconds to wait=w786) -> ()  [unwired: 1 out]
          }
          frame #1 {
            n336 = local read "Array 3"() -> (w788:sgl[])
            n337 = disable-structure shown="Disabled" {
              disable-tunnel: w793 -> [w796 _]
              disable-tunnel: [w794 _] -> w790
              frame Disabled {
                n338 = for {
                  tunnel: w796 -> [w797] mode=indexing
                  shift-right: [w799] -> w794
                  shift-left: string[] [] -> [w800]
                  n339 = call "send command.vi"("Device Name"=w797) -> ("status"=w801:bool)  [unwired: 4 in]
                  n340 = Wait (ms)(milliseconds to wait=u32 1) -> ()  [unwired: 1 out]
                  n341 = case shown="True" w801 {
                    tunnel: w800 -> [w802 w805]
                    tunnel: [w802 w804] -> w799
                    tunnel: w797 -> [_ w803]
                    frame False {
                    }
                    frame True {
                      n342 = Build Array (concatenate)(w805, w803) -> (w804:string[])
                    }
                  }
                }
              }
              frame Enabled {
              }
            }
            n343 = for {
              tunnel: w793 -> [w808] mode=indexing
              shift-right: [w813] -> w791
              shift-left: string[] [] -> [w814]
              tunnel: [w807] -> w789 mode=indexing
              shift-right: [w811] -> _
              shift-left: w788 -> [w811]
              i -> [w812]
              n344 = call "IMAQ Histograph"("Image"=w808) -> ("error out"=w806:errorcluster, "Mean Value"=w807:sgl)  [unwired: 7 in, 2 out]
              n345 = Index Array(array=w811, index=w812) -> (element=w810:sgl)
              n346 = call <vilib>:"Clear Errors.vi"("error in (no error)"=w806) -> ()  [unwired: 5 in, 2 out]
              n347 = Equal?(x=w807, y=w810) -> (x = y?=w809:bool)
              n348 = case shown="False" w809 {
                tunnel: w814 -> [w817 w818]
                tunnel: [w816 w818] -> w813
                tunnel: w808 -> [w815 _]
                frame False {
                  n349 = Build Array (concatenate)(w817, w815) -> (w816:string[])
                }
                frame True {
                }
              }
            }
            "Array 3" <- w789
          }
        }
        n350 = Equal?(x=w725, y="T") -> (x = y?=w723:bool)
        n351 = Unbundle By Name(w740) -> ("active cams"=w733:string[])
        n352 = call <vilib>:"Add State(s) to Queue__jki_lib_state_machine.vi"("State(s) in (\"\")"=w749) -> ("States Out"=w735:string)  [unwired: 14 in]
        n353 = Equal?(x=w733, y=w728) -> (x = y?=w739:bool[])
        n354 = Empty Array?(array=w733) -> (empty?=w738:bool)
        n355 = Not(x=w738) -> (.not. x?=w737:bool)
        n356 = Build Array (concatenate)(w739, w737) -> (w736:bool[])
        n357 = Array Size(array=w728) -> (size(s)=w732:i32)
        n358 = Array Size(array=w733) -> (size(s)=w731:i32)
        n359 = And Array Elements(Boolean array=w736) -> (logical AND=w729:bool)
        n360 = Equal?(x=w732, y=w731) -> (x = y?=w730:bool)
        n361 = And(x=w730, y=w729) -> (x .and. y?=w727:bool)
        n362 = Not(x=w727) -> (.not. x?=w724:bool)
        n363 = Or(x=w724, y=w723) -> (x .or. y?=w722:bool)
        n364 = case shown="True" w722 {
          tunnel: [w752 w768] -> w746
          tunnel: w745 -> [_ _]
          tunnel: w744 -> [w751 w766]
          tunnel: [w751 w766] -> w743
          tunnel: w740 -> [w752 w762]
          tunnel: w728 -> [_ w763]
          tunnel: w735 -> [w750 _]
          tunnel: [w750 w756] -> w734
          frame False {
          }
          frame True {
            n365 = property on="active CCDs" class="LstBox (strict)"("Item Names"=w763) -> ()  [unwired: 2 in, 2 out]
            n366 = Array Size(array=w763) -> (size(s)=w775:i32)
            n367 = Initialize Array(0.0 ("element"), w775, 0 ("dimension size")) -> (w770:dbl[][])
            n368 = Unbundle By Name(w762) -> ("img to avg"=w761:i32)
            n369 = Bundle By Name(cluster=w762, "active cams"=w763) -> (w769:T34)
            n370 = Initialize Array(0.0 ("element"), 12 ("dimension size"), w761) -> (w760:dbl[][])
            n371 = local write "Numeric"(0.0 ("Numeric")) -> ()
            n372 = Bundle By Name(cluster=w769, "Offset X stats"=w770, "Offset Y stats"=w770, "Centroid X"=w760, "Centroid Y"=w760, "Mean Centroid X"=w770, "Mean Centroid Y"=w770, "Offset X"=w770, "Offset Y"=w770, "Size"=w760, "Mean Size"=w770, "Motor X"=w770, "Motor Y"=w770) -> (w768:T34)
            n373 = for {
              N: 1 -> [_]
              shift-right: [w777] -> w773
              shift-left: timestamp[][] [] ("Time") -> [w779]
              n374 = for {
                N: 12 -> [_]
                tunnel: w779 -> [w782] mode=indexing
                tunnel: [w780] -> w777 mode=indexing
                n375 = Get Date/Time In Seconds() -> (seconds since 1Jan1904=w781:timestamp)
                n376 = Build Array (concatenate)(w782, w781) -> (w780:timestamp[])
              }
            }
            n377 = property on="config path" class="Str"() -> ("Value"=w758:string)  [unwired: 2 in, 2 out]
            n378 = call <vilib>:"Add State(s) to Queue__jki_lib_state_machine.vi"("State(s) in Front (\"\")"="Move Config\nMotor Config\nDetection Config\nactive\nCenter" ("State(s) in Front (\"\")"), "State(s) in (\"\")"="" ("State(s) in (\"\")")) -> ("States Out"=w757:string)  [unwired: 13 in]
            n379 = call <vilib>:"Build State String with Arguments__jki_lib_state_machine.vi"("Arguments (\"\")"=w758, "State"="Load Config" ("State(s) in Front (\"\")")) -> ("State with Arguments"=w755:string)  [unwired: 4 in]
            n380 = call <vilib>:"Add State(s) to Queue__jki_lib_state_machine.vi"("State(s) in (\"\")"=w757, "State(s) at Back (\"\")"=w755) -> ("States Out"=w756:string)  [unwired: 13 in]
            n381 = property on="Time" class="Arr (strict)"("Value"=w773) -> ()  [unwired: 2 in, 2 out]
            "name array" <- w763
          }
        }
      }
      frame "Load Config" {
        # "Your code here.\n(You can make a copy of, or modify, this frame)"
        n382 = Unbundle By Name(w864) -> ("detection para"=w870:T7[], "move properties"=w867:T10[], "thresholds"=w860:cluster{"Lower value":sgl, "Upper value":sgl}[])
        n383 = Empty String/Path?(string/path=w839) -> (empty?=w838:bool)
        n384 = case shown="False" w838 {
          tunnel: [w880 T30 {"CCDs"=[], "move properties"=[], "detection para"=[], "thresholds"=[], "Motors X"={"Motor CCD 1"=0, "Motor CCD 2"=0, "Motor CCD 3"=0, "Motor CCD 4"=0, "Motor CCD 5"=0, "Motor CCD 6"=0, "Motor CCD 7"=0, "Motor CCD 8"=0, "Motor CCD 9"=0, "Motor CCD 10"=0, "Motor CCD 11"=0, "Motor CCD 12"=0}, "Motors Y"={"Motor CCD 1"=0, "Motor CCD 2"=0, "Motor CCD 3"=0, "Motor CCD 4"=0, "Motor CCD 5"=0, "Motor CCD 6"=0, "Motor CCD 7"=0, "Motor CCD 8"=0, "Motor CCD 9"=0, "Motor CCD 10"=0, "Motor CCD 11"=0, "Motor CCD 12"=0}} ("motor cfg")] -> w872
          tunnel: [w879 w887] -> w843
          tunnel: w840 -> [w878 w887]
          tunnel: w839 -> [w877 _]
          frame False {
            n385 = String To Path(string=w877) -> (path=w876:path)
            n386 = Open/Create/Replace File(file path (use dialog)=w876, error in=w878, operation (0:open)=T31."open or create") -> (refnum out=w882:refnum<file>, error out=w883:errorcluster)  [unwired: 3 in, 1 out]
            n387 = Read from Binary File(5:T30 {"CCDs"=[], "move properties"=[], "detection para"=[], "thresholds"=[], "Motors X"={"Motor CCD 1"=0, "Motor CCD 2"=0, "Motor CCD 3"=0, "Motor CCD 4"=0, "Motor CCD 5"=0, "Motor CCD 6"=0, "Motor CCD 7"=0, "Motor CCD 8"=0, "Motor CCD 9"=0, "Motor CCD 10"=0, "Motor CCD 11"=0, "Motor CCD 12"=0}, "Motors Y"={"Motor CCD 1"=0, "Motor CCD 2"=0, "Motor CCD 3"=0, "Motor CCD 4"=0, "Motor CCD 5"=0, "Motor CCD 6"=0, "Motor CCD 7"=0, "Motor CCD 8"=0, "Motor CCD 9"=0, "Motor CCD 10"=0, "Motor CCD 11"=0, "Motor CCD 12"=0}} ("motor cfg"), 8:w883, 11:w882) -> (0:w884:errorcluster, 2:w880:T30, 3:w885:refnum<file>)  [unwired: 3 in, 1 out]
            n388 = Close File(refnum=w885, error in=w884) -> (error out=w879:errorcluster)  [unwired: 1 out]
          }
          frame True {
          }
        }
        n389 = property on="Load Config" class="Bool (strict)"("Value"=FALSE ("Load Config")) -> ()  [unwired: 2 in, 2 out]
        n390 = Unbundle By Name(w872) -> ("Motors X"=w858:T4, "Motors Y"=w820:T4, "CCDs"=w871:string[], "detection para"=w869:T7[], "move properties"=w868:T10[], "thresholds"=w861:cluster{"Lower value":sgl, "Upper value":sgl}[])
        n391 = Cluster To Array(cluster=w820) -> (array=w834:u16[])
        n392 = Cluster To Array(cluster=w858) -> (array=w859:u16[])
        n393 = call <vilib>:"Add State(s) to Queue__jki_lib_state_machine.vi"("State(s) in (\"\")"=w874, "State(s) at Back (\"\")"="Motor Config" ("State(s) at Back (\"\")")) -> ("States Out"=w873:string)  [unwired: 13 in]
        n394 = for {
          tunnel: w871 -> [w905]
          tunnel: w869 -> [w907]
          tunnel: w868 -> [w906]
          shift-right: [w899] -> w866
          shift-left: w870 -> [w904]
          shift-right: [w897] -> w865
          shift-left: w867 -> [w903]
          tunnel: w862 -> [w902] mode=indexing
          tunnel: w861 -> [w898]
          shift-right: [w894] -> w836
          shift-left: w860 -> [w896]
          tunnel: w859 -> [w893]
          tunnel: [w891] -> w857 mode=indexing
          tunnel: w834 -> [w890]
          tunnel: [w888] -> w821 mode=indexing
          i -> [w892]
          n395 = call-poly <userlib>:"Filter 1D Array__ogtk.vi"("items to filter"=w902, "array"=w905) -> ("filtered item indices"=w908:i32[])  [unwired: 4 in, 1 out]
          n396 = Index Array(array=w908) -> (element=w889:i32)  [unwired: 1 in]
          n397 = Index Array(array=w893, index=w889) -> (element=w891:u16)
          n398 = Index Array(array=w907, index=w889) -> (element=w901:T7)
          n399 = Index Array(array=w906, index=w889) -> (element=w900:T10)
          n400 = Index Array(array=w898, index=w889) -> (element=w895:cluster{"Lower value":sgl, "Upper value":sgl})
          n401 = Index Array(array=w890, index=w889) -> (element=w888:u16)
          n402 = Replace Array Subset(array=w904, new element=w901, index=w892) -> (w899:T7[])
          n403 = Replace Array Subset(array=w903, new element=w900, index=w892) -> (w897:T10[])
          n404 = Replace Array Subset(array=w896, new element=w895, index=w892) -> (w894:cluster{"Lower value":sgl, "Upper value":sgl}[])
        }
        n405 = Array Size(array=w836) -> (size(s)=→"size(s) 6":i32)
        n406 = Index Array(array=w857) -> (element #1=w856:u16, element #2=w855:u16, element #3=w854:u16, element #4=w853:u16, element #5=w852:u16, element #6=w851:u16, element #7=w850:u16, element #8=w849:u16, element #9=w848:u16, element #10=w847:u16, element #11=w846:u16, element #12=w845:u16)  [unwired: 12 in]
        n407 = Index Array(array=w821) -> (element #1=w822:u16, element #2=w823:u16, element #3=w824:u16, element #4=w825:u16, element #5=w826:u16, element #6=w827:u16, element #7=w828:u16, element #8=w829:u16, element #9=w830:u16, element #10=w831:u16, element #11=w832:u16, element #12=w833:u16)  [unwired: 12 in]
        n408 = Bundle By Name(cluster=w858, "Motor CCD 1"=w856, "Motor CCD 2"=w855, "Motor CCD 3"=w854, "Motor CCD 4"=w853, "Motor CCD 5"=w852, "Motor CCD 6"=w851, "Motor CCD 7"=w850, "Motor CCD 8"=w849, "Motor CCD 9"=w848, "Motor CCD 10"=w847, "Motor CCD 11"=w846, "Motor CCD 12"=w845) -> (w844:T4)
        n409 = Bundle By Name(cluster=w820, "Motor CCD 1"=w822, "Motor CCD 2"=w823, "Motor CCD 3"=w824, "Motor CCD 4"=w825, "Motor CCD 5"=w826, "Motor CCD 6"=w827, "Motor CCD 7"=w828, "Motor CCD 8"=w829, "Motor CCD 9"=w830, "Motor CCD 10"=w831, "Motor CCD 11"=w832, "Motor CCD 12"=w833) -> (w819:T4)
        n410 = Bundle By Name(cluster=w864, "detection para"=w866, "move properties"=w865, "thresholds"=w836) -> (w863:T34)
        n411 = property on="associated motors X" class="Clust (strict)"(error in=w843, "Val(Sgnl)"=w844) -> (error out=w842:errorcluster)  [unwired: 1 in, 1 out]
        n412 = local write "associated motors Y"(w819) -> ()
      }
      frame "Save Config" {
        w917 = T39 {"Camera names"=[], "Motor aliases x"=[], "Motor aliases y"=[], "detection para"=[], "thresholds"=[], "move properties"=[]}  # BP Configuration
        n413 = Unbundle By Name(w928) -> ("move properties"=w920:T10[], "detection para"=w919:T7[], "thresholds"=w918:cluster{"Lower value":sgl, "Upper value":sgl}[])
        n414 = property on="associated motors X" class="Clust (strict)"() -> ("Value"=w916:T4)  [unwired: 2 in, 2 out]
        n415 = property on="Save Config" class="Bool (strict)"("Value"=FALSE ("Save Config")) -> ()  [unwired: 2 in, 2 out]
        n416 = local read "associated motors Y"() -> (w911:T4)
        n417 = Cluster To Array(cluster=w916) -> (array=w915:u16[])
        n418 = property on="Motor CCD 1" class="Ring (strict)"() -> ("Strings []"=w912:string[])  [unwired: 2 in, 2 out]
        n419 = Cluster To Array(cluster=w911) -> (array=w913:u16[])
        n420 = call "File Dialog"("pattern (all files)"="*.cfg", "pattern label"="config") -> ("selected path"=w923:path)  [unwired: 10 in, 3 out]
        n421 = call-poly <userlib>:"Index Array Elements__ogtk.vi"("indices"=w915, "array"=w912) -> ("elements"=w914:string[])  [unwired: 9 in]
        n422 = call-poly <userlib>:"Index Array Elements__ogtk.vi"("indices"=w913, "array"=w912) -> ("elements"=w910:string[])  [unwired: 9 in]
        n423 = local read "CCDs"() -> (w921:string[])
        n424 = Bundle By Name(cluster=w917, "Camera names"=w921, "move properties"=w920, "detection para"=w919, "thresholds"=w918, "Motor aliases x"=w914, "Motor aliases y"=w910) -> (w909:T39)
        n425 = disable-structure shown="Enabled" {
          disable-tunnel: w927 -> [w934 w942]
          disable-tunnel: [w933 w941] -> w926
          disable-tunnel: w923 -> [w932 w940]
          disable-tunnel: w909 -> [w931 w943]
          frame Disabled {
            n426 = Open/Create/Replace File(file path (use dialog)=w932, error in=w934, operation (0:open)=T31."replace or create with confirmation") -> (refnum out=w936:refnum<file>, error out=w937:errorcluster)  [unwired: 3 in, 1 out]
            n427 = Write to Binary File(file (use dialog)=w936, data=w931, error in=w937) -> (refnum out=w939:refnum<file>, error out=w938:errorcluster)  [unwired: 3 in, 1 out]
            n428 = Close File(refnum=w939, error in=w938) -> (error out=w933:errorcluster)  [unwired: 1 out]
          }
          frame Enabled {
            n429 = call <userlib>:"MGI Write Anything.vi"("Error In"=w942, "Anything"=w943, "Path (dialog)"=w940) -> ("Error Out"=w941:errorcluster)  [unwired: 6 in, 2 out]
          }
        }
        n430 = call <vilib>:"Add State(s) to Queue__jki_lib_state_machine.vi"("State(s) in (\"\")"=w930) -> ("States Out"=w929:string)  [unwired: 14 in]
      }
      frame "active" {
        # "Your code here.\n(You can make a copy of, or modify, this frame)"
        n431 = Empty String/Path?(string/path=w958) -> (empty?=w957:bool)
        n432 = Unbundle By Name(w954) -> ("move properties"=w970:T10[], "detection para"=w966:T7[])  [unwired: 1 out]
        n433 = Unbundle By Name(w954) -> ("active axis refs 2"=w953:T11)
        n434 = call-poly <userlib>:"Filter 1D Array__ogtk.vi"("items to filter"=w958, "array"=w968) -> ("filtered item indices"=w971:i32[])  [unwired: 4 in, 1 out]
        n435 = Index Array(array=w971) -> (element=w955:i32)  [unwired: 1 in]
        n436 = Select(t=0, s=w957, f=w955) -> (s? t:f=w951:i32)
        n437 = Index Array(array=w953, index=w951) -> (element=w952:cluster{"Ref X":refnum<vi>, "Ref Y":refnum<vi>})
        n438 = Unbundle By Name(w952) -> ("Ref X"=w950:refnum<vi>, "Ref Y"=w949:refnum<vi>)
        n439 = Index Array(array=w970, index=w951) -> (element=w969:T10)
        n440 = Index Array(array=w966, index=w951) -> (element=w965:T7)
        n441 = property on="move config" class="Clust (strict)"(error in=w961, "Value"=w969) -> (error out=w959:errorcluster)  [unwired: 1 in, 1 out]
        n442 = property on="beam detection para" class="Clust (strict)"(error in=w959, "Value"=w965) -> (error out=w960:errorcluster)  [unwired: 1 in, 1 out]
        n443 = call <vilib>:"Add State(s) to Queue__jki_lib_state_machine.vi"("State(s) in (\"\")"=w973) -> ("States Out"=w972:string)  [unwired: 14 in]
        n444 = Bundle By Name(cluster="active Axis ref 3", "Ref X"=w950, "Ref Y"=w949) -> (w963:cluster{"Ref X":refnum<vi>, "Ref Y":refnum<vi>})
        n445 = property class="DigNum (strict)"(reference=w950, error in=w960) -> (error out=w946:errorcluster, "Value"=w948:dbl)  [unwired: 1 out]
        n446 = Bundle By Name(cluster=w954, "active ccd"=w951, "active man refs"=w963) -> (w967:T34)
        n447 = property on="Position 1" class="DigNum (strict)"(error in=w946, "Value"=w948) -> (error out=w945:errorcluster)  [unwired: 1 in, 1 out]
        n448 = property class="DigNum (strict)"(reference=w949, error in=w945) -> (error out=w944:errorcluster, "Value"=w947:dbl)  [unwired: 1 out]
        n449 = property on="Position 2" class="DigNum (strict)"(error in=w944, "Value"=w947) -> (error out=w962:errorcluster)  [unwired: 1 in, 1 out]
      }
      frame "Detection Config" {
        # "Your code here.\n(You can make a copy of, or modify, this frame)"
        n450 = Unbundle By Name(w978) -> ("detection para"=w974:T7[], "active ccd"=w979:i32)
        n451 = Replace Array Subset(array=w974, new element="beam detection para", index=w979) -> (w975:T7[])
        n452 = Bundle By Name(cluster=w978, "detection para"=w975) -> (w977:T34)
        n453 = call <vilib>:"Add State(s) to Queue__jki_lib_state_machine.vi"("State(s) in (\"\")"=w982) -> ("States Out"=w981:string)  [unwired: 14 in]
      }
      frame "Motor Config" {
        # "Your code here.\n(You can make a copy of, or modify, this frame)"
        n454 = Unbundle By Name("associated motors X") -> ("Motor CCD 1"=w1012:u16, "Motor CCD 2"=w1013:u16, "Motor CCD 3"=w1014:u16, "Motor CCD 4"=w1007:u16, "Motor CCD 5"=w1006:u16, "Motor CCD 6"=w1005:u16, "Motor CCD 7"=w1004:u16, "Motor CCD 8"=w1003:u16, "Motor CCD 9"=w1002:u16, "Motor CCD 10"=w1001:u16, "Motor CCD 11"=w1000:u16, "Motor CCD 12"=w999:u16)
        n455 = Unbundle By Name("associated motors Y") -> ("Motor CCD 1"=w988:u16, "Motor CCD 2"=w987:u16, "Motor CCD 3"=w986:u16, "Motor CCD 4"=w989:u16, "Motor CCD 5"=w990:u16, "Motor CCD 6"=w991:u16, "Motor CCD 7"=w992:u16, "Motor CCD 8"=w993:u16, "Motor CCD 9"=w994:u16, "Motor CCD 10"=w995:u16, "Motor CCD 11"=w996:u16, "Motor CCD 12"=w997:u16)
        n456 = Build Array(w1012, w1013, w1014, w1007, w1006, w1005, w1004, w1003, w1002, w1001, w1000, w999) -> (w984:u16[])
        n457 = Build Array(w988, w987, w986, w989, w990, w991, w992, w993, w994, w995, w996, w997) -> (w983:u16[])
        n458 = local read "motor refs"() -> (w1010:refnum<vi>[])
        n459 = for {
          tunnel: w984 -> [w1019] mode=indexing
          tunnel: w1010 -> [w1024]
          tunnel: [w1020] -> w998 mode=indexing
          tunnel: w983 -> [w1018] mode=indexing
          n460 = Index Array(array=w1024, index=w1019) -> (element=w1023:refnum<vi>)
          n461 = Index Array(array=w1024, index=w1018) -> (element=w1022:refnum<vi>)
          n462 = Bundle By Name(cluster=cluster{"Ref X":refnum<vi>, "Ref Y":refnum<vi>} {"Ref X"=refnum, "Ref Y"=refnum} ("active Axis ref"), "Ref Y"=w1023, "Ref X"=w1022) -> (w1020:cluster{"Ref X":refnum<vi>, "Ref Y":refnum<vi>})
        }
        n463 = call <vilib>:"Add State(s) to Queue__jki_lib_state_machine.vi"("State(s) in (\"\")"=w1017) -> ("States Out"=w1016:string)  [unwired: 14 in]
        n464 = Bundle By Name(cluster=w1009, "active axis refs 2"=w998) -> (w1008:T34)
      }
      frame "Move Config" {
        # "Your code here.\n(You can make a copy of, or modify, this frame)"
        n465 = Unbundle By Name(w1026) -> ("move properties"=w1030:T10[], "active ccd"=w1029:i32)
        n466 = Replace Array Subset(array=w1030, new element="move config", index=w1029) -> (w1027:T10[])
        n467 = Bundle By Name(cluster=w1026, "move properties"=w1027) -> (w1025:T34)
        n468 = call <vilib>:"Add State(s) to Queue__jki_lib_state_machine.vi"("State(s) in (\"\")"=w1033) -> ("States Out"=w1032:string)  [unwired: 14 in]
      }
      frame "----------Centroid & Move----------" {
        # "Template Separator\n(You can make a copy of, or modify, this frame)"
        n469 = call <vilib>:"Add State(s) to Queue__jki_lib_state_machine.vi"("State(s) in (\"\")"=w1037) -> ("States Out"=w1036:string)  [unwired: 14 in]
      }
      frame "detected" {
        n470 = Unbundle By Name(w1045) -> ("Offset X"=w1077:dbl[][], "Offset Y"=w1076:dbl[][], "Size"=w1075:dbl[][], "Mean Size"=w1074:dbl[][], "Time"=w1071:timestamp[][], "Motor X"=w1054:dbl[][], "active axis refs 2"=w1053:T11, "Motor Y"=w1052:dbl[][])
        n471 = Spreadsheet String To Array(format string="%s", spreadsheet string=w1057, array type (2D Dbl)=string[] []) -> (array=w1048:string[])  [unwired: 1 in]
        n472 = for {
          tunnel: w1049 -> [w1090] mode=indexing
          tunnel: w1048 -> [w1089]
          tunnel: [w1088] -> w1047 mode=indexing
          n473 = for {
            tunnel: w1090 -> [w1093]
            tunnel: [w1092] -> w1087 mode=indexing
            tunnel: w1089 -> [w1091] mode=indexing
            n474 = Equal?(x=w1093, y=w1091) -> (x = y?=w1092:bool)
          }
          n475 = Or Array Elements(Boolean array=w1087) -> (logical OR=w1088:bool)
        }
        n476 = Unbundle By Name(w1045) -> ("Mean Centroid X"=w1081:dbl[][], "Mean Centroid Y"=w1080:dbl[][], "Centroid X"=w1083:dbl[][], "Centroid Y"=w1082:dbl[][])
        n477 = call <vilib>:"Add State(s) to Queue__jki_lib_state_machine.vi"("State(s) in (\"\")"=w1056) -> ("States Out"=w1055:string)  [unwired: 14 in]
        n478 = for {
          tunnel: w1083 -> [w1143]
          tunnel: w1082 -> [w1142]
          tunnel: w1081 -> [w1141]
          tunnel: w1080 -> [w1140]
          tunnel: [w1139] -> w1068 mode=indexing
          tunnel: [w1138] -> w1079 mode=indexing
          tunnel: w1078 -> [w1137] mode=indexing
          tunnel: w1077 -> [w1136]
          tunnel: w1076 -> [w1135]
          tunnel: [w1134] -> w1046 mode=indexing
          tunnel: [w1133] -> w1069 mode=indexing
          tunnel: w1075 -> [w1132]
          tunnel: w1074 -> [w1131]
          tunnel: [w1130] -> w1073 mode=indexing
          tunnel: w1071 -> [w1129]
          tunnel: [w1128] -> w1070 mode=indexing
          tunnel: w1054 -> [w1120]
          tunnel: w1053 -> [w1119]
          tunnel: w1052 -> [w1118]
          tunnel: [w1098] -> w1051 mode=indexing
          tunnel: [w1097] -> w1050 mode=indexing
          tunnel: w1047 -> [w1096]
          i -> [w1095]
          n479 = Unbundle By Name(w1137) -> ("Target.X::12"=w1102:refnum<vi>, "Target.Y::12"=w1101:refnum<vi>)
          n480 = Index Array(array=w1120, index (row)=w1095) -> (element=w1123:dbl[])  [unwired: 1 in]
          n481 = Index Array(array=w1119, index=w1095) -> (element=w1122:cluster{"Ref X":refnum<vi>, "Ref Y":refnum<vi>})
          n482 = Index Array(array=w1118, index (row)=w1095) -> (element=w1127:dbl[])  [unwired: 1 in]
          n483 = Index Array(array=w1096, index=w1095) -> (element=w1094:bool)
          n484 = Index Array(array=w1141, index (row)=w1095) -> (element=w1114:dbl[])  [unwired: 1 in]
          n485 = Index Array(array=w1140, index (row)=w1095) -> (element=w1115:dbl[])  [unwired: 1 in]
          n486 = Index Array(array=w1143, index (row)=w1095) -> (element=w1117:dbl[])  [unwired: 1 in]
          n487 = Index Array(array=w1142, index (row)=w1095) -> (element=w1116:dbl[])  [unwired: 1 in]
          n488 = Index Array(array=w1136, index (row)=w1095) -> (element=w1110:dbl[])  [unwired: 1 in]
          n489 = Index Array(array=w1135, index (row)=w1095) -> (element=w1109:dbl[])  [unwired: 1 in]
          n490 = Index Array(array=w1132, index (row)=w1095) -> (element=w1107:dbl[])  [unwired: 1 in]
          n491 = Index Array(array=w1131, index (row)=w1095) -> (element=w1106:dbl[])  [unwired: 1 in]
          n492 = Index Array(array=w1129, index (row)=w1095) -> (element=w1103:timestamp[])  [unwired: 1 in]
          n493 = Unbundle By Name(w1122) -> ("Ref X"=w1121:refnum<vi>, "Ref Y"=w1125:refnum<vi>)
          n494 = property class="DigNum (strict)"(reference=w1102) -> ("Value"=w1100:dbl)  [unwired: 1 in, 2 out]
          n495 = property class="DigNum (strict)"(reference=w1101) -> ("Value"=w1099:dbl)  [unwired: 1 in, 2 out]
          n496 = call <vilib>:"Std Deviation and Variance.vi"("X"=w1117) -> ("mean"=w1113:dbl)  [unwired: 1 in, 2 out]
          n497 = call <vilib>:"Std Deviation and Variance.vi"("X"=w1116) -> ("mean"=w1112:dbl)  [unwired: 1 in, 2 out]
          n498 = call <vilib>:"Std Deviation and Variance.vi"("X"=w1107) -> ("mean"=w1105:dbl)  [unwired: 1 in, 2 out]
          n499 = Get Date/Time In Seconds() -> (seconds since 1Jan1904=w1104:timestamp)
          n500 = property class="DigNum (strict)"(reference=w1121) -> ("Value"=w1124:dbl)  [unwired: 1 in, 2 out]
          n501 = property class="DigNum (strict)"(reference=w1125) -> ("Value"=w1126:dbl)  [unwired: 1 in, 2 out]
          n502 = Subtract(x=w1100, y=w1113) -> (x-y=w1111:dbl)
          n503 = Subtract(x=w1099, y=w1112) -> (x-y=w1108:dbl)
          n504 = case shown="True" w1094 {
            tunnel: [w1156 w1175] -> w1139
            tunnel: [w1144 w1174] -> w1138
            tunnel: [w1145 w1173] -> w1134
            tunnel: [w1146 w1172] -> w1133
            tunnel: [w1147 w1171] -> w1130
            tunnel: [w1148 w1170] -> w1128
            tunnel: w1115 -> [w1154 w1169]
            tunnel: w1114 -> [w1155 w1168]
            tunnel: w1113 -> [_ w1167]
            tunnel: w1112 -> [_ w1166]
            tunnel: w1111 -> [_ w1165]
            tunnel: w1110 -> [w1153 w1164]
            tunnel: w1109 -> [w1152 w1163]
            tunnel: w1108 -> [_ w1162]
            tunnel: w1106 -> [w1151 w1161]
            tunnel: w1105 -> [_ w1160]
            tunnel: w1104 -> [w1149 w1159]
            tunnel: w1103 -> [w1150 w1158]
            frame False {
              w1157 = 0.0
              n505 = Build Array (concatenate)(w1155, w1157) -> (w1156:dbl[])
              n506 = Build Array (concatenate)(w1154, w1157) -> (w1144:dbl[])
              n507 = Build Array (concatenate)(w1153, w1157) -> (w1145:dbl[])
              n508 = Build Array (concatenate)(w1152, w1157) -> (w1146:dbl[])
              n509 = Build Array (concatenate)(w1151, w1157) -> (w1147:dbl[])
              n510 = Build Array (concatenate)(w1150, w1149) -> (w1148:timestamp[])
            }
            frame True {
              n511 = Build Array (concatenate)(w1168, w1167) -> (w1175:dbl[])
              n512 = Build Array (concatenate)(w1169, w1166) -> (w1174:dbl[])
              n513 = Build Array (concatenate)(w1164, w1165) -> (w1173:dbl[])
              n514 = Build Array (concatenate)(w1163, w1162) -> (w1172:dbl[])
              n515 = Build Array (concatenate)(w1161, w1160) -> (w1171:dbl[])
              n516 = Build Array (concatenate)(w1158, w1159) -> (w1170:timestamp[])
            }
          }
          n517 = Build Array (concatenate)(w1123, w1124) -> (w1098:dbl[])
          n518 = Build Array (concatenate)(w1127, w1126) -> (w1097:dbl[])
        }
        n519 = local write "Numeric"(0.0 ("Numeric")) -> ()
        n520 = Array Size(array=w1046) -> (size(s)=w1067:i32[])
        n521 = Index Array(array=w1067, index=1) -> (element=w1065:i32)
        "History Index" <- w1065
        n522 = call <vilib>:"Add State(s) to Queue__jki_lib_state_machine.vi"("State(s) in (\"\")"=w1055, "State(s) at Back (\"\")"="Check Move\ntdms" ("State(s) at Back (\"\")")) -> ("States Out"=w1059:string)  [unwired: 13 in]
        n523 = Unbundle By Name(w1045) -> ("img to avg"=w1042:i32)
        n524 = Initialize Array(0.0 ("element"), 12 ("dimension size"), w1042) -> (w1041:dbl[][])
        n525 = Greater?(x=w1065, y="History Size") -> (0:w1063:bool)
        n526 = Bundle By Name(cluster=w1045, "Centroid X"=w1041, "Centroid Y"=w1041, "Mean Centroid X"=w1068, "Mean Centroid Y"=w1079, "Offset X"=w1046, "Offset Y"=w1069, "Mean Size"=w1073, "Size"=w1041, "Time"=w1070, "Motor X"=w1051, "Motor Y"=w1050) -> (w1038:T34)
        n527 = Select(t="history" ("State(s) at Back (\"\")"), s=w1063, f="") -> (s? t:f=w1060:string)
        n528 = call <vilib>:"Add State(s) to Queue__jki_lib_state_machine.vi"("State(s) in (\"\")"=w1059, "State(s) at Back (\"\")"=w1060) -> ("States Out"=w1040:string)  [unwired: 13 in]
        n529 = call <vilib>:"Add State(s) to Queue__jki_lib_state_machine.vi"("State(s) in (\"\")"=w1040) -> ("States Out"=w1039:string)  [unwired: 14 in]
      }
      frame "Check Move" {
        (unwired) "Device Ini" ("State(s) in Front (\"\")")
        n530 = Unbundle By Name(w1184) -> ("move properties"=w1194:T10[], "Mean Size"=w1193:dbl[][], "move properties"=w1192:T10[], "Offset X"=w1191:dbl[][], "Offset Y"=w1190:dbl[][], "active cams"=w1189:string[])
        n531 = Unbundle By Name(w1184) -> ("steps speed X"=w1183:dbl[], "steps speed Y"=w1182:dbl[])
        n532 = for {
          tunnel: w1192 -> [w1232]
          tunnel: w1191 -> [w1230]
          tunnel: w1190 -> [w1228]
          tunnel: w1193 -> [w1236]
          tunnel: [w1247] -> w1178 mode=indexing
          tunnel: [w1243] -> w1176 mode=indexing
          tunnel: w1189 -> [w1237] mode=indexing
          tunnel: [w1265] -> w1195 mode=indexing
          tunnel: [w1264] -> w1187 mode=indexing
          tunnel: w1194 -> [w1235]
          tunnel: [w1226] -> w1179 mode=indexing
          tunnel: [w1225] -> w1177 mode=indexing
          tunnel: "Speedmode" -> [w1240]
          tunnel: w1186 -> [w1238]
          shift-right: [w1218] -> w1181
          shift-left: w1183 -> [w1223]
          shift-right: [w1217] -> w1180
          shift-left: w1182 -> [w1222]
          n533 = call-poly <userlib>:"Filter 1D Array__ogtk.vi"("items to filter"=w1237, "array"=w1238) -> ("filtered item indices"=w1239:i32[])  [unwired: 4 in, 1 out]
          n534 = Index Array(array=w1239) -> (element=w1221:i32)  [unwired: 1 in]
          n535 = Index Array(array=w1235, index=w1221) -> (element=w1234:T10)
          n536 = Index Array(array=w1236, index (row)=w1221) -> (element=w1233:dbl[])  [unwired: 1 in]
          n537 = Index Array(array=w1232, index=w1221) -> (element=w1231:T10)
          n538 = Index Array(array=w1230, index (row)=w1221) -> (element=w1229:dbl[])  [unwired: 1 in]
          n539 = Index Array(array=w1228, index (row)=w1221) -> (element=w1227:dbl[])  [unwired: 1 in]
          n540 = Unbundle By Name(w1231) -> ("Tolerance [%]"=w1258:dbl)
          n541 = Reverse 1D Array(array=w1229) -> (reversed array=w1263:dbl[])
          n542 = Reverse 1D Array(array=w1227) -> (reversed array=w1262:dbl[])
          n543 = Reverse 1D Array(array=w1233) -> (reversed array=w1257:dbl[])
          n544 = Unbundle By Name(w1234) -> ("Stepsize"=w1216:dbl, "enable feedback"=w1246:bool)
          n545 = Index Array(array=w1263) -> (element=w1261:dbl)  [unwired: 1 in]
          n546 = Index Array(array=w1262) -> (element=w1260:dbl)  [unwired: 1 in]
          n547 = Index Array(array=w1257) -> (element=w1256:dbl)  [unwired: 1 in]
          n548 = Absolute Value(x=w1261) -> (abs(x)=w1224:dbl)
          n549 = Absolute Value(x=w1260) -> (abs(x)=w1242:dbl)
          n550 = Square Root(x=w1256) -> (sqrt(x)=w1255:dbl)
          n551 = Divide(x=w1258, y=100.0) -> (x/y=w1254:dbl)
          n552 = Multiply(x=w1255, y=w1254) -> (x*y=w1241:dbl)
          n553 = Not Equal To 0?(x=w1242) -> (x != 0?=w1244:bool)
          n554 = Not Equal To 0?(x=w1224) -> (x != 0?=w1249:bool)
          n555 = Greater Or Equal?(x=w1224, y=w1241) -> (x >= y?=w1248:bool)
          n556 = Greater Or Equal?(x=w1242, y=w1241) -> (x >= y?=w1245:bool)
          n557 = call "speedmode.vi"("offset X"=w1224, "offset Y"=w1242, "beamsize x tolerance"=w1241, "Speedmode @"=w1240, "step size"=w1216) -> ("steps speed Y"=w1219:dbl, "steps speed X"=w1220:dbl, "speedmode X"=w1226:bool, "speedmode Y"=w1225:bool)  [unwired: 3 in]
          n558 = Compound Arithmetic op=AND(w1246, w1249, w1248) -> (w1247:bool)
          n559 = Compound Arithmetic op=AND(w1246, w1245, w1244) -> (w1243:bool)
          n560 = Boolean To (0,1)(Boolean=w1243) -> (0, 1=w1250:i16)
          n561 = Multiply(x=w1250, y=w1242) -> (x*y=w1251:dbl)
          n562 = Boolean To (0,1)(Boolean=w1247) -> (0, 1=w1253:i16)
          n563 = Replace Array Subset(array=w1223, new element=w1220, index=w1221) -> (w1218:dbl[])
          n564 = Replace Array Subset(array=w1222, new element=w1219, index=w1221) -> (w1217:dbl[])
          n565 = Multiply(x=w1253, y=w1224) -> (x*y=w1252:dbl)
          n566 = Bundle(w1251, "GUIdevice 8"=w1237) -> (w1264:cluster{dbl, "GUIdevice 8":string})  [unwired: 1 in]
          n567 = Bundle(w1252, "GUIdevice 8"=w1237) -> (w1265:cluster{dbl, "GUIdevice 8":string})  [unwired: 1 in]
        }
        "required X" <- w1178
        "required Y" <- w1176
        "speedmode X" <- w1179
        "speedmode Y" <- w1177
        n568 = case shown="False" "Align" {
          tunnel: w1195 -> [w1271 w1276]
          tunnel: w1187 -> [w1270 w1273]
          tunnel: [w1269 w1275] -> w1198
          tunnel: [w1268 w1272] -> w1197
          frame False {
            n569 = Sort 1D Array(array=w1270) -> (sorted array=w1267:cluster{dbl, "GUIdevice 8":string}[])
            n570 = Sort 1D Array(array=w1271) -> (sorted array=w1266:cluster{dbl, "GUIdevice 8":string}[])
            n571 = Reverse 1D Array(array=w1267) -> (reversed array=w1268:cluster{dbl, "GUIdevice 8":string}[])
            n572 = Reverse 1D Array(array=w1266) -> (reversed array=w1269:cluster{dbl, "GUIdevice 8":string}[])
          }
          frame True {
            w1274 = cluster{dbl, "GUIdevice 8":string}[] [] ("Array")
            n573 = for {
              shift-right: [w1286] -> w1275
              shift-left: w1274 -> [w1288]
              tunnel: w1276 -> [w1287] mode=indexing
              n574 = Unbundle(w1287) -> (w1290:dbl)  [unwired: 1 out]
              n575 = Not Equal To 0?(x=w1290) -> (x != 0?=w1289:bool)
              n576 = case shown="True" w1289 {
                tunnel: w1288 -> [w1291 w1294]
                tunnel: w1287 -> [_ w1293]
                tunnel: [w1291 w1292] -> w1286
                frame False {
                }
                frame True {
                  n577 = Build Array (concatenate)(w1294, w1293) -> (w1292:cluster{dbl, "GUIdevice 8":string}[])
                }
              }
            }
            n578 = for {
              shift-right: [w1277] -> w1272
              shift-left: w1274 -> [w1279]
              tunnel: w1273 -> [w1278] mode=indexing
              n579 = Unbundle(w1278) -> (w1281:dbl)  [unwired: 1 out]
              n580 = Not Equal To 0?(x=w1281) -> (x != 0?=w1280:bool)
              n581 = case shown="True" w1280 {
                tunnel: w1279 -> [w1282 w1285]
                tunnel: w1278 -> [_ w1284]
                tunnel: [w1282 w1283] -> w1277
                frame False {
                }
                frame True {
                  n582 = Build Array (concatenate)(w1285, w1284) -> (w1283:cluster{dbl, "GUIdevice 8":string}[])
                }
              }
            }
          }
        }
        n583 = call <vilib>:"Add State(s) to Queue__jki_lib_state_machine.vi"("State(s) in (\"\")"=w1201) -> ("States Out"=w1200:string)  [unwired: 14 in]
        n584 = Bundle By Name(cluster=w1184, "speedmode X"=w1179, "speedmode Y"=w1177, "steps speed X"=w1181, "steps speed Y"=w1180) -> (w1185:T34)
        n585 = Index Array(array=w1197) -> (element=w1202:cluster{dbl, "GUIdevice 8":string})  [unwired: 1 in]
        n586 = Index Array(array=w1198) -> (element=w1203:cluster{dbl, "GUIdevice 8":string})  [unwired: 1 in]
        n587 = Empty Array?(array=w1197) -> (empty?=w1205:bool)
        n588 = Unbundle(w1203) -> (w1211:dbl)  [unwired: 1 out]
        n589 = Unbundle(w1202) -> (w1207:dbl)  [unwired: 1 out]
        n590 = Unbundle By Name(w1185) -> ("Feedback global"=w1212:bool)
        n591 = Empty Array?(array=w1198) -> (empty?=w1209:bool)
        n592 = property on="autodetect" class="Bool (strict)"("Value"=FALSE ("autodetect")) -> ()  [unwired: 2 in, 2 out]
        n593 = Equal To 0?(x=w1211) -> (x = 0?=w1210:bool)
        n594 = Equal To 0?(x=w1207) -> (x = 0?=w1206:bool)
        n595 = Or(x=w1210, y=w1209) -> (x .or. y?=w1208:bool)
        n596 = Or(x=w1206, y=w1205) -> (x .or. y?=w1204:bool)
        n597 = case shown="True" w1212 {
          tunnel: w1208 -> [_ w1313]
          tunnel: w1198 -> [_ w1312]
          tunnel: w1204 -> [_ w1310]
          tunnel: w1197 -> [_ w1309]
          tunnel: w1200 -> [w1295 w1308]
          tunnel: [w1295 w1307] -> w1213
          tunnel: w1179 -> [_ w1306]
          tunnel: w1178 -> [_ w1305]
          tunnel: w1177 -> [_ w1304]
          tunnel: w1176 -> [_ w1303]
          frame False {
          }
          frame True {
            n598 = case shown="False" w1313 {
              tunnel: w1312 -> [w1337 _]
              tunnel: w1308 -> [w1333 w1338]
              tunnel: [w1331 w1338] -> w1311
              frame False {
                n599 = Index Array(array=w1337) -> (element=w1336:cluster{dbl, "GUIdevice 8":string})  [unwired: 1 in]
                n600 = Unbundle By Name(w1336) -> ("GUIdevice 8"=w1335:string)
                n601 = call <vilib>:"Build State String with Arguments__jki_lib_state_machine.vi"("Arguments (\"\")"=w1335, "State"="Move X") -> ("State with Arguments"=w1332:string)  [unwired: 4 in]
                n602 = call <vilib>:"Add State(s) to Queue__jki_lib_state_machine.vi"("State(s) in (\"\")"=w1333, "State(s) at Back (\"\")"=w1332) -> ("States Out"=w1331:string)  [unwired: 13 in]
              }
              frame True {
              }
            }
            n603 = case shown="False" w1310 {
              tunnel: w1309 -> [w1329 _]
              tunnel: w1311 -> [w1325 w1330]
              tunnel: [w1323 w1330] -> w1307
              frame False {
                n604 = Index Array(array=w1329) -> (element=w1328:cluster{dbl, "GUIdevice 8":string})  [unwired: 1 in]
                n605 = Unbundle By Name(w1328) -> ("GUIdevice 8"=w1327:string)
                n606 = call <vilib>:"Build State String with Arguments__jki_lib_state_machine.vi"("Arguments (\"\")"=w1327, "State"="Move Y") -> ("State with Arguments"=w1324:string)  [unwired: 4 in]
                n607 = call <vilib>:"Add State(s) to Queue__jki_lib_state_machine.vi"("State(s) in (\"\")"=w1325, "State(s) at Back (\"\")"=w1324) -> ("States Out"=w1323:string)  [unwired: 13 in]
              }
              frame True {
              }
            }
            n608 = for {
              tunnel: w1306 -> [w1322] mode=indexing
              tunnel: w1305 -> [w1321] mode=indexing
              tunnel: [w1320] -> w1302 mode=indexing
              n609 = And(x=w1322, y=w1321) -> (x .and. y?=w1320:bool)
            }
            n610 = for {
              tunnel: w1304 -> [w1319] mode=indexing
              tunnel: w1303 -> [w1318] mode=indexing
              tunnel: [w1317] -> w1301 mode=indexing
              n611 = And(x=w1319, y=w1318) -> (x .and. y?=w1317:bool)
            }
            n612 = Or Array Elements(Boolean array=w1302) -> (logical OR=w1300:bool)
            n613 = Or Array Elements(Boolean array=w1301) -> (logical OR=w1299:bool)
            n614 = Or(x=w1300, y=w1299) -> (x .or. y?=w1298:bool)
            n615 = property on="alarms" class="Bool (strict)"() -> ("Value"=w1297:bool)  [unwired: 2 in, 2 out]
            n616 = And(x=w1297, y=w1298) -> (x .and. y?=w1296:bool)
            n617 = case shown="True" w1296 {
              frame False {
              }
              frame True {
                n618 = call <vilib>:"Beep.vi"("use system alert? (T)"=FALSE, "duration (msec)"=u32 750, "frequency (Hz)"=u32 750) -> ()  [unwired: 9 in]
              }
            }
          }
        }
        n619 = call <vilib>:"Add State(s) to Queue__jki_lib_state_machine.vi"("State(s) in (\"\")"=w1200, "State(s) at Back (\"\")"=w1213) -> ("States Out"=w1215:string)  [unwired: 13 in]
      }
      frame "Move X" {
        # "Your code here.\n(You can make a copy of, or modify, this frame)"
        n620 = Unbundle By Name(w1342) -> ("Offset X"=w1357:dbl[][])
        n621 = call-poly <userlib>:"Filter 1D Array__ogtk.vi"("items to filter"=w1345, "array"=w1361) -> ("filtered item indices"=w1349:i32[])  [unwired: 4 in, 1 out]
        n622 = Unbundle By Name(w1342) -> ("active axis refs 2"=w1360:T11, "move properties"=w1343:T10[])
        n623 = for {
          tunnel: w1349 -> [w1366] mode=indexing
          tunnel: w1343 -> [w1370]
          shift-right: [w1365] -> w1347
          shift-left: i32[] [] ("filtered item indices") -> [w1368]
          n624 = Index Array(array=w1370, index=w1366) -> (element=w1369:T10)
          n625 = Unbundle By Name(w1369) -> ("enable feedback"=w1367:bool)
          n626 = case shown="True" w1367 {
            tunnel: w1368 -> [w1371 w1374]
            tunnel: w1366 -> [_ w1373]
            tunnel: [w1371 w1372] -> w1365
            frame False {
            }
            frame True {
              n627 = Build Array (concatenate)(w1374, w1373) -> (w1372:i32[])
            }
          }
        }
        n628 = Index Array(array=w1347) -> (element=w1340:i32)  [unwired: 1 in]
        n629 = Index Array(array=w1357, index (row)=w1340) -> (element=w1356:dbl[])  [unwired: 1 in]
        n630 = Reverse 1D Array(array=w1356) -> (reversed array=w1355:dbl[])
        n631 = Index Array(array=w1360, index=w1340) -> (element=w1359:cluster{"Ref X":refnum<vi>, "Ref Y":refnum<vi>})
        n632 = Index Array(array=w1355) -> (element=w1354:dbl)  [unwired: 1 in]
        n633 = Index Array(array=w1343, index=w1340) -> (element=w1358:T10)
        n634 = Unbundle By Name(w1359) -> ("Ref X"=w1351:refnum<vi>)
        n635 = Unbundle By Name(w1358) -> ("Invert Direction X"=w1352:bool, "enable feedback"=w1350:bool)  [unwired: 1 out]
        n636 = Greater Or Equal To 0?(x=w1354) -> (x >= 0?=w1353:bool)
        n637 = Unbundle By Name(w1342) -> ("steps speed X"=w1341:dbl[])  [unwired: 1 out]
        n638 = Index Array(array=w1341, index=w1340) -> (element=w1339:dbl)
        n639 = case shown="True" w1350 {
          tunnel: w1353 -> [_ w1378]
          tunnel: w1339 -> [_ w1377]
          tunnel: w1352 -> [_ w1376]
          tunnel: w1351 -> [_ w1375]
          frame False {
          }
          frame True {
            n640 = case shown="True" w1378 {
              tunnel: w1376 -> [w1383 w1394]
              tunnel: w1377 -> [w1381 w1392]
              tunnel: w1375 -> [w1379 w1390]
              frame True {
                n641 = property class="DigNum (strict)"(reference=w1379) -> ("Value"=w1382:dbl)  [unwired: 1 in, 2 out]
                n642 = case shown="True" w1383 {
                  tunnel: w1382 -> [w1386 w1389]
                  tunnel: w1381 -> [w1385 w1388]
                  tunnel: [w1384 w1387] -> w1380
                  frame False {
                    n643 = Add(x=w1386, y=w1385) -> (x+y=w1384:dbl)
                  }
                  frame True {
                    n644 = Subtract(x=w1389, y=w1388) -> (x-y=w1387:dbl)
                  }
                }
                n645 = property class="DigNum (strict)"(reference=w1379, "Val(Sgnl)"=w1380) -> ()  [unwired: 1 in, 2 out]
              }
              frame False {
                n646 = property class="DigNum (strict)"(reference=w1390) -> ("Value"=w1393:dbl)  [unwired: 1 in, 2 out]
                n647 = case shown="False" w1394 {
                  tunnel: w1393 -> [w1397 w1400]
                  tunnel: w1392 -> [w1396 w1399]
                  tunnel: [w1395 w1398] -> w1391
                  frame False {
                    n648 = Subtract(x=w1397, y=w1396) -> (x-y=w1395:dbl)
                  }
                  frame True {
                    n649 = Add(x=w1400, y=w1399) -> (x+y=w1398:dbl)
                  }
                }
                n650 = property class="DigNum (strict)"(reference=w1390, "Val(Sgnl)"=w1391) -> ()  [unwired: 1 in, 2 out]
              }
            }
          }
        }
        n651 = call <vilib>:"Build State String with Arguments__jki_lib_state_machine.vi"("Arguments (\"\")"=w1345, "State"="Wait" ("State(s) in Front (\"\")")) -> ("State with Arguments"=w1344:string)  [unwired: 4 in]
        n652 = call <vilib>:"Add State(s) to Queue__jki_lib_state_machine.vi"("State(s) in Front (\"\")"=w1344, "State(s) in (\"\")"=w1364) -> ("States Out"=w1363:string)  [unwired: 13 in]
        "Moving X" <- w1345
      }
      frame "ManMove X" {
        # "Your code here.\n(You can make a copy of, or modify, this frame)"
        n653 = Unbundle By Name(w1412) -> ("move properties"=w1409:T10[], "active ccd"=w1405:i32, "active man refs"=w1407:cluster{"Ref X":refnum<vi>, "Ref Y":refnum<vi>}, "active cams"=w1406:string[])
        n654 = Index Array(array=w1406, index=w1405) -> (element=w1403:string)
        n655 = Index Array(array=w1409, index=w1405) -> (element=w1413:T10)
        n656 = Unbundle By Name(w1407) -> ("Ref X"=w1410:refnum<vi>)
        n657 = Unbundle By Name(w1413) -> ("Invert Direction X"=w1411:bool)  [unwired: 1 out]
        n658 = call <vilib>:"Build State String with Arguments__jki_lib_state_machine.vi"("Arguments (\"\")"=w1403, "State"="Wait" ("State(s) in Front (\"\")")) -> ("State with Arguments"=w1402:string)  [unwired: 4 in]
        n659 = call <vilib>:"Add State(s) to Queue__jki_lib_state_machine.vi"("State(s) in Front (\"\")"=w1402, "State(s) in (\"\")"=w1416) -> ("States Out"=w1415:string)  [unwired: 13 in]
        n660 = case shown="\"Left\", Default" w1401 {
          tunnel: w1411 -> [w1421 w1432]
          tunnel: "StepSize" -> [w1419 w1430]
          tunnel: w1410 -> [w1417 w1428]
          frame "Right" {
            n661 = property class="DigNum (strict)"(reference=w1417) -> ("Value"=w1420:dbl)  [unwired: 1 in, 2 out]
            n662 = case shown="False" w1421 {
              tunnel: w1420 -> [w1424 w1427]
              tunnel: w1419 -> [w1423 w1426]
              tunnel: [w1422 w1425] -> w1418
              frame False {
                n663 = Add(x=w1424, y=w1423) -> (x+y=w1422:dbl)
              }
              frame True {
                n664 = Subtract(x=w1427, y=w1426) -> (x-y=w1425:dbl)
              }
            }
            n665 = property class="DigNum (strict)"(reference=w1417, "Val(Sgnl)"=w1418) -> ()  [unwired: 1 in, 2 out]
          }
          frame "Left", Default {
            n666 = property class="DigNum (strict)"(reference=w1428) -> ("Value"=w1431:dbl)  [unwired: 1 in, 2 out]
            n667 = case shown="True" w1432 {
              tunnel: w1431 -> [w1435 w1438]
              tunnel: w1430 -> [w1434 w1437]
              tunnel: [w1433 w1436] -> w1429
              frame False {
                n668 = Subtract(x=w1435, y=w1434) -> (x-y=w1433:dbl)
              }
              frame True {
                n669 = Add(x=w1438, y=w1437) -> (x+y=w1436:dbl)
              }
            }
            n670 = property class="DigNum (strict)"(reference=w1428, "Val(Sgnl)"=w1429) -> ()  [unwired: 1 in, 2 out]
          }
        }
      }
      frame "ManMove Y" {
        # "Your code here.\n(You can make a copy of, or modify, this frame)"
        n671 = Equal?(x=w1439, y="Down") -> ()  [unwired: 1 out]
        n672 = Unbundle By Name(w1451) -> ("active cams"=w1444:string[], "move properties"=w1450:T10[], "active ccd"=w1443:i32, "active man refs"=w1449:cluster{"Ref X":refnum<vi>, "Ref Y":refnum<vi>})
        n673 = Index Array(array=w1444, index=w1443) -> (element=w1441:string)
        n674 = property on="StepSize" class="DigNum (strict)"() -> ("Value"=w1445:dbl)  [unwired: 2 in, 2 out]
        n675 = Index Array(array=w1450, index=w1443) -> (element=w1452:T10)
        n676 = Unbundle By Name(w1449) -> ("Ref Y"=w1446:refnum<vi>)
        n677 = Unbundle By Name(w1452) -> ("Invert Direction Y"=w1447:bool)  [unwired: 1 out]
        n678 = call <vilib>:"Build State String with Arguments__jki_lib_state_machine.vi"("Arguments (\"\")"=w1441, "State"="Wait" ("State(s) in Front (\"\")")) -> ("State with Arguments"=w1440:string)  [unwired: 4 in]
        n679 = call <vilib>:"Add State(s) to Queue__jki_lib_state_machine.vi"("State(s) in Front (\"\")"=w1440, "State(s) in (\"\")"=w1455) -> ("States Out"=w1454:string)  [unwired: 13 in]
        n680 = case shown="\"Down\"" w1439 {
          tunnel: w1447 -> [w1460 w1471]
          tunnel: w1445 -> [w1458 w1469]
          tunnel: w1446 -> [w1456 w1467]
          frame "Down" {
            n681 = property class="DigNum (strict)"(reference=w1456) -> ("Value"=w1459:dbl)  [unwired: 1 in, 2 out]
            n682 = case shown="False" w1460 {
              tunnel: w1459 -> [w1463 w1466]
              tunnel: w1458 -> [w1462 w1465]
              tunnel: [w1461 w1464] -> w1457
              frame False {
                n683 = Add(x=w1463, y=w1462) -> (x+y=w1461:dbl)
              }
              frame True {
                n684 = Subtract(x=w1466, y=w1465) -> (x-y=w1464:dbl)
              }
            }
            n685 = property class="DigNum (strict)"(reference=w1456, "Val(Sgnl)"=w1457) -> ()  [unwired: 1 in, 2 out]
          }
          frame "Up", Default {
            n686 = property class="DigNum (strict)"(reference=w1467) -> ("Value"=w1470:dbl)  [unwired: 1 in, 2 out]
            n687 = case shown="False" w1471 {
              tunnel: w1470 -> [w1474 w1477]
              tunnel: w1469 -> [w1473 w1476]
              tunnel: [w1472 w1475] -> w1468
              frame False {
                n688 = Subtract(x=w1474, y=w1473) -> (x-y=w1472:dbl)
              }
              frame True {
                n689 = Add(x=w1477, y=w1476) -> (x+y=w1475:dbl)
              }
            }
            n690 = property class="DigNum (strict)"(reference=w1467, "Val(Sgnl)"=w1468) -> ()  [unwired: 1 in, 2 out]
          }
        }
      }
      frame "Move Y" {
        # "Your code here.\n(You can make a copy of, or modify, this frame)"
        n691 = Unbundle By Name(w1479) -> ("Offset Y"=w1499:dbl[][])
        n692 = call-poly <userlib>:"Filter 1D Array__ogtk.vi"("items to filter"=w1487, "array"=w1503) -> ("filtered item indices"=w1492:i32[])  [unwired: 4 in, 1 out]
        n693 = Unbundle By Name(w1479) -> ("active axis refs 2"=w1502:T11, "move properties"=w1490:T10[])
        n694 = for {
          tunnel: w1492 -> [w1508] mode=indexing
          tunnel: w1490 -> [w1512]
          shift-right: [w1507] -> w1491
          shift-left: i32[] [] ("filtered item indices") -> [w1510]
          n695 = Index Array(array=w1512, index=w1508) -> (element=w1511:T10)
          n696 = Unbundle By Name(w1511) -> ("enable feedback"=w1509:bool)
          n697 = case shown="True" w1509 {
            tunnel: w1510 -> [w1513 w1516]
            tunnel: w1508 -> [_ w1515]
            tunnel: [w1513 w1514] -> w1507
            frame False {
            }
            frame True {
              n698 = Build Array (concatenate)(w1516, w1515) -> (w1514:i32[])
            }
          }
        }
        n699 = Index Array(array=w1491) -> (element=w1481:i32)  [unwired: 1 in]
        n700 = Index Array(array=w1499, index (row)=w1481) -> (element=w1498:dbl[])  [unwired: 1 in]
        n701 = Reverse 1D Array(array=w1498) -> (reversed array=w1497:dbl[])
        n702 = Index Array(array=w1502, index=w1481) -> (element=w1501:cluster{"Ref X":refnum<vi>, "Ref Y":refnum<vi>})
        n703 = Index Array(array=w1497) -> (element=w1496:dbl)  [unwired: 1 in]
        n704 = Index Array(array=w1490, index=w1481) -> (element=w1500:T10)
        n705 = Unbundle By Name(w1501) -> ("Ref Y"=w1494:refnum<vi>)
        n706 = Unbundle By Name(w1500) -> ("Invert Direction Y"=w1480:bool, "enable feedback"=w1493:bool)  [unwired: 1 out]
        n707 = Greater Or Equal To 0?(x=w1496) -> (x >= 0?=w1495:bool)
        n708 = Unbundle By Name(w1479) -> ("steps speed X"=w1485:dbl[], "steps speed Y"=w1484:dbl[])
        n709 = Index Array(array=w1484, index=w1481) -> (element=w1482:dbl)
        n710 = Index Array(array=w1485, index=w1481) -> (element=w1483:dbl)
        n711 = Select(t=w1483, s=w1480, f=w1482) -> (s? t:f=w1478:dbl)
        n712 = case shown="True" w1493 {
          tunnel: w1495 -> [_ w1520]
          tunnel: w1478 -> [_ w1519]
          tunnel: w1480 -> [_ w1518]
          tunnel: w1494 -> [_ w1517]
          frame False {
          }
          frame True {
            n713 = case shown="True" w1520 {
              tunnel: w1518 -> [w1525 w1536]
              tunnel: w1519 -> [w1523 w1534]
              tunnel: w1517 -> [w1521 w1532]
              frame True {
                n714 = property class="DigNum (strict)"(reference=w1521) -> ("Value"=w1524:dbl)  [unwired: 1 in, 2 out]
                n715 = case shown="False" w1525 {
                  tunnel: w1524 -> [w1528 w1531]
                  tunnel: w1523 -> [w1527 w1530]
                  tunnel: [w1526 w1529] -> w1522
                  frame False {
                    n716 = Add(x=w1528, y=w1527) -> (x+y=w1526:dbl)
                  }
                  frame True {
                    n717 = Subtract(x=w1531, y=w1530) -> (x-y=w1529:dbl)
                  }
                }
                n718 = property class="DigNum (strict)"(reference=w1521, "Val(Sgnl)"=w1522) -> ()  [unwired: 1 in, 2 out]
              }
              frame False {
                n719 = property class="DigNum (strict)"(reference=w1532) -> ("Value"=w1535:dbl)  [unwired: 1 in, 2 out]
                n720 = case shown="False" w1536 {
                  tunnel: w1535 -> [w1539 w1542]
                  tunnel: w1534 -> [w1538 w1541]
                  tunnel: [w1537 w1540] -> w1533
                  frame False {
                    n721 = Subtract(x=w1539, y=w1538) -> (x-y=w1537:dbl)
                  }
                  frame True {
                    n722 = Add(x=w1542, y=w1541) -> (x+y=w1540:dbl)
                  }
                }
                n723 = property class="DigNum (strict)"(reference=w1532, "Val(Sgnl)"=w1533) -> ()  [unwired: 1 in, 2 out]
              }
            }
          }
        }
        n724 = call <vilib>:"Build State String with Arguments__jki_lib_state_machine.vi"("Arguments (\"\")"=w1487, "State"="Wait" ("State(s) in Front (\"\")")) -> ("State with Arguments"=w1486:string)  [unwired: 4 in]
        n725 = call <vilib>:"Add State(s) to Queue__jki_lib_state_machine.vi"("State(s) in Front (\"\")"=w1486, "State(s) in (\"\")"=w1506) -> ("States Out"=w1505:string)  [unwired: 13 in]
        "Moving Y" <- w1487
      }
      frame "Wait" {
        # "Your code here.\n(You can make a copy of, or modify, this frame)"
        n726 = call-poly <userlib>:"Filter 1D Array__ogtk.vi"("items to filter"=w1552, "array"=w1553) -> ("filtered item indices"=w1551:i32[])  [unwired: 4 in, 1 out]
        n727 = flat-sequence {
          tunnel: T32."Disabled and Grayed Out" ("Disabled") -> [w1559]
          tunnel: w1549 -> [w1568]
          tunnel: w1548 -> [w1567]
          tunnel: [w1566] -> w1547
          tunnel: w1546 -> [w1565]
          tunnel: w1545 -> [w1564]
          tunnel: T32."Enabled" ("Disabled") -> [w1578]
          frame #0 {
            n728 = property on="Right" class="Bool (strict)"("DisabledEnum"=w1559) -> ()  [unwired: 2 in, 2 out]
            n729 = property on="Up" class="Bool (strict)"("DisabledEnum"=w1559) -> ()  [unwired: 2 in, 2 out]
            n730 = property on="Left" class="Bool (strict)"("DisabledEnum"=w1559) -> ()  [unwired: 2 in, 2 out]
            n731 = property on="Down" class="Bool (strict)"("DisabledEnum"=w1559) -> ()  [unwired: 2 in, 2 out]
            n732 = property on="StepSize" class="DigNum (strict)"("DisabledEnum"=w1559) -> ()  [unwired: 2 in, 2 out]
          }
          frame #1 {
            n733 = Wait (ms)(milliseconds to wait=u32 1500) -> ()  [unwired: 1 out]
          }
          frame #2 {
            n734 = property on="Moving Y" class="Str"("Value"="") -> ()  [unwired: 2 in, 2 out]
            n735 = property on="Moving X" class="Str"("Value"="") -> ()  [unwired: 2 in, 2 out]
          }
          frame #3 {
            n736 = Equal?(x=w1564, y=w1565) -> (x = y?=w1563:bool)
            n737 = case shown="True" w1563 {
              tunnel: w1568 -> [_ w1575]
              tunnel: w1567 -> [w1569 w1572]
              tunnel: [w1569 w1570] -> w1566
              frame False {
              }
              frame True {
                n738 = Unbundle By Name(w1575) -> ("Ref X"=w1574:refnum<vi>, "Ref Y"=w1573:refnum<vi>)
                n739 = property class="DigNum (strict)"(reference=w1574, error in=w1572) -> (error out=w1571:errorcluster, "Value"=w1577:dbl)  [unwired: 1 out]
                n740 = property class="DigNum (strict)"(reference=w1573, error in=w1571) -> (error out=w1570:errorcluster, "Value"=w1576:dbl)  [unwired: 1 out]
                n741 = property on="Position 1" class="DigNum (strict)"("Value"=w1577) -> ()  [unwired: 2 in, 2 out]
                n742 = property on="Position 2" class="DigNum (strict)"("Value"=w1576) -> ()  [unwired: 2 in, 2 out]
              }
            }
          }
          frame #4 {
            n743 = property on="Right" class="Bool (strict)"("DisabledEnum"=w1578) -> ()  [unwired: 2 in, 2 out]
            n744 = property on="Up" class="Bool (strict)"("DisabledEnum"=w1578) -> ()  [unwired: 2 in, 2 out]
            n745 = property on="Left" class="Bool (strict)"("DisabledEnum"=w1578) -> ()  [unwired: 2 in, 2 out]
            n746 = property on="Down" class="Bool (strict)"("DisabledEnum"=w1578) -> ()  [unwired: 2 in, 2 out]
            n747 = property on="StepSize" class="DigNum (strict)"("DisabledEnum"=w1578) -> ()  [unwired: 2 in, 2 out]
          }
        }
        n748 = Index Array(array=w1551) -> (element=w1546:i32)  [unwired: 1 in]
        n749 = Unbundle By Name(w1554) -> ("active axis refs 2"=w1550:T11, "active ccd"=w1545:i32)
        n750 = Index Array(array=w1550, index=w1546) -> (element=w1549:cluster{"Ref X":refnum<vi>, "Ref Y":refnum<vi>})
        n751 = call <vilib>:"Add State(s) to Queue__jki_lib_state_machine.vi"("State(s) in (\"\")"=w1558) -> ("States Out"=w1557:string)  [unwired: 14 in]
        n752 = local read "Mean Centroid X"() -> (w1555:dbl[][])
        n753 = Bundle By Name(cluster=w1554, "Mean Centroid X"=w1555, "Mean Centroid Y"=w1555) -> (w1556:T34)
      }
      frame "---------------Statistics--------------" {
        # "Template Separator\n(You can make a copy of, or modify, this frame)"
        n754 = call <vilib>:"Add State(s) to Queue__jki_lib_state_machine.vi"("State(s) in (\"\")"=w1582) -> ("States Out"=w1581:string)  [unwired: 14 in]
      }
      frame "Save Stats" {
        # "Your code here.\n(You can make a copy of, or modify, this frame)"
        n755 = property on="CCD 1" class="XYGraph (strict)"() -> ("Value"=w1593:cluster{timestamp[], dbl[]}[])  [unwired: 2 in, 2 out]
        n756 = property on="CCD 2" class="XYGraph (strict)"() -> ("Value"=w1592:cluster{timestamp[], dbl[]}[])  [unwired: 2 in, 2 out]
        n757 = property on="CCD 3" class="XYGraph (strict)"() -> ("Value"=w1591:cluster{timestamp[], dbl[]}[])  [unwired: 2 in, 2 out]
        n758 = property on="CCD 4" class="XYGraph (strict)"() -> ("Value"=w1590:cluster{timestamp[], dbl[]}[])  [unwired: 2 in, 2 out]
        n759 = property on="CCD 5" class="XYGraph (strict)"() -> ("Value"=w1589:cluster{timestamp[], dbl[]}[])  [unwired: 2 in, 2 out]
        n760 = property on="CCD 6" class="XYGraph (strict)"() -> ("Value"=w1588:cluster{timestamp[], dbl[]}[])  [unwired: 2 in, 2 out]
        n761 = property on="CCD 7" class="XYGraph (strict)"() -> ("Value"=w1587:cluster{timestamp[], dbl[]}[])  [unwired: 2 in, 2 out]
        n762 = property on="CCD 8" class="XYGraph (strict)"() -> ("Value"=w1586:cluster{timestamp[], dbl[]}[])  [unwired: 2 in, 2 out]
        n763 = Build Array(w1593, w1592, w1591, w1590, w1589, w1588, w1587, w1586) -> (w1585:cluster{timestamp[], dbl[]}[][])
        n764 = disable-structure shown="Disabled" {
          disable-tunnel: w1597 -> [w1601 _]
          disable-tunnel: [w1600 _] -> w1596
          disable-tunnel: w1585 -> [w1599 _]
          disable-tunnel: w1584 -> [w1598 _]
          frame Disabled {
            n765 = for {
              tunnel: w1599 -> [w1604] mode=indexing
              tunnel: w1598 -> [w1603] mode=indexing
              n766 = Empty String/Path?(string/path=w1603) -> (empty?=w1602:bool)
              n767 = case shown="False" w1602 {
                tunnel: w1604 -> [w1610 _]
                tunnel: w1603 -> [w1608 _]
                frame False {
                  n768 = Index Array(array=w1610, index #1=0 ("index"), index #2=1 ("index"), index #3=2 ("index"), index #4=3 ("index")) -> (element #1=w1645:cluster{timestamp[], dbl[]}, element #2=w1639:cluster{timestamp[], dbl[]}, element #3=w1638:cluster{timestamp[], dbl[]}, element #4=w1637:cluster{timestamp[], dbl[]})  [unwired: 1 in, 1 out]
                  n769 = Concatenate Strings(w1608, ".dat" ("string")) -> (w1606:string)
                  n770 = Unbundle(w1645) -> (w1644:timestamp[], w1622:dbl[])
                  n771 = Unbundle(w1639) -> (w1613:dbl[])  [unwired: 1 out]
                  n772 = Unbundle(w1638) -> (w1612:dbl[])  [unwired: 1 out]
                  n773 = Unbundle(w1637) -> (w1611:dbl[])  [unwired: 1 out]
                  n774 = Build Path(base path="save path", name or relative path=w1606) -> (appended path=w1605:path)
                  n775 = for {
                    tunnel: w1644 -> [w1647] mode=indexing
                    tunnel: [w1646] -> w1620 mode=indexing
                    n776 = Format Date/Time String(time format string (%c)="%Y%m%d%H%M%S", seconds (now)=w1647) -> (date/time string=w1646:string)  [unwired: 1 in]
                  }
                  n777 = Array Size(array=w1622) -> (size(s)=w1623:i32)
                  n778 = Number To Fractional String(number=w1622) -> (F-format string=w1619:string[])  [unwired: 3 in]
                  n779 = Number To Fractional String(number=w1613) -> (F-format string=w1616:string[])  [unwired: 3 in]
                  n780 = Number To Fractional String(number=w1612) -> (F-format string=w1615:string[])  [unwired: 3 in]
                  n781 = Number To Fractional String(number=w1611) -> (F-format string=w1614:string[])  [unwired: 3 in]
                  n782 = Initialize Array("", w1623, 5 ("dimension size")) -> (w1621:string[][])
                  n783 = Insert Into Array(array=w1621, index (col)=0 ("disabled index (col)"), new element=w1620) -> (w1631:string[][])  [unwired: 1 in]
                  n784 = Insert Into Array(array=w1631, index (col)=1 ("disabled index (col)"), new element=w1619) -> (w1630:string[][])  [unwired: 1 in]
                  n785 = Insert Into Array(array=w1630, index (col)=2 ("disabled index (col)"), new element=w1616) -> (w1634:string[][])  [unwired: 1 in]
                  n786 = Insert Into Array(array=w1634, index (col)=3 ("disabled index (col)"), new element=w1615) -> (w1635:string[][])  [unwired: 1 in]
                  n787 = Insert Into Array(array=w1635, index (col)=4 ("disabled index (col)"), new element=w1614) -> (w1636:string[][])  [unwired: 1 in]
                  n788 = Insert Into Array(array=w1636, index (row)=0, new element=string[] ["time", "Centroid X", "Centroid Y", "Motor Axis 1", "Motor Axis 2"] ("new element/subarray 2")) -> (w1618:string[][])  [unwired: 1 in]
                  n789 = call-poly <vilib>:"Write To Spreadsheet File.vi"("2D data"=w1618, "file path (dialog if empty)"=w1605) -> ()  [unwired: 6 in, 1 out]
                }
                frame True {
                }
              }
            }
            n790 = call <vilib>:"Add State(s) to Queue__jki_lib_state_machine.vi"("State(s) in (\"\")"=w1601) -> ("States Out"=w1600:string)  [unwired: 14 in]
          }
          frame Enabled {
          }
        }
        n791 = property on="Save Stats" class="Bool (strict)"("Value"=FALSE ("Save Stats")) -> ()  [unwired: 2 in, 2 out]
      }
      frame "tdms" {
        w1659 = 21600.0 ("new tdms")
        # "Your code here.\n(You can make a copy of, or modify, this frame)"
        n792 = Unbundle By Name(w1667) -> ("active cams"=w1652:string[], "Data Value Reference out"=w1649:refnum<k34>, "Offset X"=w1666:dbl[][], "Offset Y"=w1665:dbl[][], "active axis refs 2"=w1664:T11)
        n793 = for {
          tunnel: w1666 -> [w1714]
          tunnel: w1665 -> [w1713]
          tunnel: w1652 -> [w1677] mode=indexing
          tunnel: w1649 -> [w1678]
          tunnel: w1664 -> [w1699]
          tunnel: w1669 -> [w1683]
          tunnel: [w1681] -> w1668
          i -> [w1700]
          n794 = Index Array(array=w1714, index (row)=w1700) -> (element=w1712:dbl[])  [unwired: 1 in]
          n795 = Index Array(array=w1713, index (row)=w1700) -> (element=w1711:dbl[])  [unwired: 1 in]
          n796 = Index Array(array=w1699, index=w1700) -> (element=w1698:cluster{"Ref X":refnum<vi>, "Ref Y":refnum<vi>})
          n797 = Reverse 1D Array(array=w1711) -> (reversed array=w1709:dbl[])
          n798 = Reverse 1D Array(array=w1712) -> (reversed array=w1710:dbl[])
          n799 = Unbundle By Name(w1698) -> ("Ref X"=w1697:refnum<vi>, "Ref Y"=w1696:refnum<vi>)
          n800 = Index Array(array=w1710) -> (element=w1708:dbl)  [unwired: 1 in]
          n801 = Index Array(array=w1709) -> (element=w1707:dbl)  [unwired: 1 in]
          n802 = property class="DigNum (strict)"(reference=w1697, error in=w1683) -> (error out=w1682:errorcluster, "Value"=w1691:dbl)  [unwired: 1 out]
          n803 = Build Array(w1708) -> (w1680:dbl[])
          n804 = Build Array(w1707) -> (w1702:dbl[])
          n805 = Get Date/Time In Seconds() -> (seconds since 1Jan1904=w1679:timestamp)
          n806 = Build Array(w1679) -> (w1675:timestamp[])
          n807 = property class="DigNum (strict)"(reference=w1696, error in=w1682) -> (error out=w1673:errorcluster, "Value"=w1685:dbl)  [unwired: 1 out]
          n808 = Build Array(w1691) -> (w1690:dbl[])
          n809 = TDMS Write(0:w1678, 5:w1677, 7:"time", 9:w1675, 11:w1673) -> (4:w1674:refnum<k34>, 15:w1672:errorcluster)  [unwired: 1 in, 2 out]
          n810 = Build Array(w1685) -> (w1684:dbl[])
          n811 = TDMS Write(0:w1674, 5:w1677, 7:"centroid X", 9:w1680, 11:w1672) -> (4:w1705:refnum<k34>, 6:w1704:string, 15:w1703:errorcluster)  [unwired: 1 in, 1 out]
          n812 = TDMS Write(0:w1705, 5:w1704, 7:"centroid Y", 9:w1702, 11:w1703) -> (4:w1694:refnum<k34>, 6:w1693:string, 15:w1695:errorcluster)  [unwired: 1 in, 1 out]
          n813 = TDMS Write(0:w1694, 5:w1693, 7:"Motor Axis 1", 9:w1690, 11:w1695) -> (4:w1689:refnum<k34>, 6:w1688:string, 15:w1686:errorcluster)  [unwired: 1 in, 1 out]
          n814 = TDMS Write(0:w1689, 5:w1688, 7:"Motor Axis 2", 9:w1684, 11:w1686) -> (15:w1681:errorcluster)  [unwired: 1 in, 3 out]
        }
        n815 = property on="millisecond timer value" class="DigNum (strict)"() -> ("Value"=w1651:u32)  [unwired: 2 in, 2 out]
        n816 = Tick Count (ms)() -> (millisecond timer value=w1650:u32)
        n817 = Unbundle By Name(w1667) -> ()  [unwired: 1 out]
        n818 = Subtract(x=w1650, y=w1651) -> (x-y=w1654:u32)
        n819 = Divide(x=w1654, y=u32 1000) -> (x/y=w1656:dbl)
        n820 = Quotient & Remainder(x=w1656, y=w1659) -> (x-y*floor(x/y)=w1657:dbl)  [unwired: 1 out]
        n821 = Subtract(x=w1659, y=20.0) -> (x-y=w1661:dbl)
        n822 = Greater?(x=w1657, y=w1661) -> (0:w1658:bool)
        n823 = Select(t="newtdms", s=w1658, f="") -> (s? t:f=w1653:string)
        n824 = call <vilib>:"Add State(s) to Queue__jki_lib_state_machine.vi"("State(s) in (\"\")"=w1671, "State(s) at Back (\"\")"=w1653) -> ("States Out"=w1670:string)  [unwired: 13 in]
      }
      frame "Reset History" {
        # "Your code here.\n(You can make a copy of, or modify, this frame)"
        n825 = for {
          N: 1 -> [_]
          shift-right: [w1724] -> w1716
          shift-left: timestamp[][] [] ("Time") -> [w1726]
          n826 = for {
            N: 12 -> [_]
            tunnel: w1726 -> [w1729] mode=indexing
            tunnel: [w1727] -> w1724 mode=indexing
            n827 = Get Date/Time In Seconds() -> (seconds since 1Jan1904=w1728:timestamp)
            n828 = Build Array (concatenate)(w1729, w1728) -> (w1727:timestamp[])
          }
        }
        n829 = local read "Offset X"() -> (w1715:dbl[][])
        n830 = Bundle By Name(cluster=w1720, "Offset X"=w1715, "Offset Y"=w1715, "Time"=w1716, "Motor X"=w1715) -> (w1719:T34)
        n831 = call <vilib>:"Add State(s) to Queue__jki_lib_state_machine.vi"("State(s) in (\"\")"=w1723) -> ("States Out"=w1722:string)  [unwired: 14 in]
      }
      frame "New Category: 2" {
        # "Your code here.\n(You can make a copy of, or modify, this frame)"
        n832 = call <vilib>:"Add State(s) to Queue__jki_lib_state_machine.vi"("State(s) in (\"\")"=w1733) -> ("States Out"=w1732:string)  [unwired: 14 in]
      }
      frame "stats" {
        # "Your code here.\n(You can make a copy of, or modify, this frame)"
        n833 = Unbundle By Name(w1748) -> ("Offset X"=w1739:dbl[][], "Offset Y"=w1738:dbl[][], "Time"=w1737:timestamp[][], "Motor X"=w1736:dbl[][], "Motor Y"=w1735:dbl[][], "Data Value Reference out"=w1743:refnum<k34>)
        n834 = TDMS List Contents(4:w1742, 7:w1743) -> (0:w1734:errorcluster, 2:w1746:string[], 3:w1745:refnum<k34>)  [unwired: 1 in, 1 out]
        n835 = call <vilib>:"ClearError.vi"("error in (no error)"=w1734) -> ("error out"=w1744:errorcluster)
        n836 = for {
          tunnel: w1744 -> [w1815]
          tunnel: [w1801] -> w1740 mode=indexing
          tunnel: [w1800] -> w1741
          tunnel: [w1799] -> _
          tunnel: w1745 -> [w1798]
          tunnel: w1746 -> [w1797] mode=indexing
          w1816 = dbl[] [] ("appended array")
          n837 = TDMS Read(0:w1798, 5:w1797, 7:"time", 11:w1815, 12:timestamp[] [] ("appended array")) -> (4:w1830:refnum<k34>, 6:w1826:string, 10:w1807:timestamp[], 15:w1814:errorcluster)  [unwired: 3 in, 2 out]
          n838 = TDMS Read(0:w1830, 5:w1826, 7:"centroid X", 11:w1814, 12:w1816) -> (4:w1829:refnum<k34>, 6:w1825:string, 10:w1810:dbl[], 15:w1813:errorcluster)  [unwired: 3 in, 2 out]
          n839 = TDMS Read(0:w1829, 5:w1825, 7:"centroid Y", 11:w1813, 12:w1816) -> (4:w1828:refnum<k34>, 6:w1824:string, 10:w1809:dbl[], 15:w1812:errorcluster)  [unwired: 3 in, 2 out]
          n840 = TDMS Read(0:w1828, 5:w1824, 7:"Motor Axis 1", 11:w1812, 12:w1816) -> (4:w1827:refnum<k34>, 6:w1823:string, 10:w1808:dbl[], 15:w1811:errorcluster)  [unwired: 3 in, 2 out]
          n841 = TDMS Read(0:w1827, 5:w1823, 7:"Motor Axis 2", 11:w1811, 12:w1816) -> (4:w1799:refnum<k34>, 10:w1806:dbl[], 15:w1800:errorcluster)  [unwired: 3 in, 3 out]
          n842 = Bundle("appended array"=w1807, "appended array"=w1810) -> (w1805:T40)  [unwired: 1 in]
          n843 = Bundle("appended array"=w1807, "appended array"=w1809) -> (w1804:T40)  [unwired: 1 in]
          n844 = Bundle("appended array"=w1807, "appended array"=w1808) -> (w1803:T40)  [unwired: 1 in]
          n845 = Bundle("appended array"=w1807, "appended array"=w1806) -> (w1802:T40)  [unwired: 1 in]
          n846 = Build Array(w1805, w1804, w1803, w1802) -> (w1801:T41)
        }
        n847 = disable-structure shown="Disabled" {
          disable-tunnel: w1747 -> [w1780 _]
          disable-tunnel: w1739 -> [w1779 _]
          disable-tunnel: w1738 -> [w1778 _]
          disable-tunnel: w1737 -> [w1777 _]
          disable-tunnel: w1736 -> [w1776 _]
          disable-tunnel: w1735 -> [w1775 _]
          frame Disabled {
            n848 = for {
              tunnel: w1780 -> [_] mode=indexing
              tunnel: w1779 -> [w1790]
              tunnel: w1778 -> [w1789]
              tunnel: w1777 -> [w1788]
              tunnel: w1776 -> [w1784]
              tunnel: w1775 -> [w1783]
              tunnel: [w1792] -> _ mode=indexing
              i -> [w1791]
              n849 = Index Array(array=w1789, index (row)=w1791) -> (element=w1785:dbl[])  [unwired: 1 in]
              n850 = Index Array(array=w1784, index (row)=w1791) -> (element=w1782:dbl[])  [unwired: 1 in]
              n851 = Index Array(array=w1783, index (row)=w1791) -> (element=w1781:dbl[])  [unwired: 1 in]
              n852 = Index Array(array=w1790, index (row)=w1791) -> (element=w1786:dbl[])  [unwired: 1 in]
              n853 = Index Array(array=w1788, index (row)=w1791) -> (element=w1787:timestamp[])  [unwired: 1 in]
              n854 = Bundle("Time"=w1787, "Motor X"=w1782) -> (w1795:cluster{"Time":timestamp[], "Motor X":dbl[]})  [unwired: 1 in]
              n855 = Bundle("Time"=w1787, "Motor Y"=w1781) -> (w1796:cluster{"Time":timestamp[], "Motor Y":dbl[]})  [unwired: 1 in]
              n856 = Bundle("Time"=w1787, "Offset X"=w1786) -> (w1794:cluster{"Time":timestamp[], "Offset X":dbl[]})  [unwired: 1 in]
              n857 = Bundle("Time"=w1787, "Offset Y"=w1785) -> (w1793:cluster{"Time":timestamp[], "Offset Y":dbl[]})  [unwired: 1 in]
              n858 = Build Array(w1793, w1794, w1795, w1796) -> (w1792:cluster{"Time":timestamp[], "Motor Y":dbl[]}[])
            }
          }
          frame Enabled {
          }
        }
        n859 = Index Array(array=w1740, index (row) #1=0 ("index (row)"), index (row) #2=1 ("index (row)"), index (row) #3=2 ("index (row)"), index (row) #4=3 ("index (row)"), index (row) #5=4 ("index (row)"), index (row) #6=5 ("index (row)"), index (row) #7=6 ("index (row)"), index (row) #8=7 ("index (row)"), index (row) #9=8 ("index (row)"), index (row) #10=9 ("index (row)"), index (row) #11=10 ("index (row)"), index (row) #12=11 ("index (row)")) -> (element #1=→"CCD 1":T41, element #2=→"CCD 2":T41, element #3=→"CCD 3":T41, element #4=→"CCD 4":T41, element #5=→"CCD 5":T41, element #6=→"CCD 6":T41, element #7=→"CCD 7":T41, element #8=→"CCD 8":T41, element #9=→"CCD 9":T41, element #10=→"CCD 10":T41, element #11=→"CCD 11":T41, element #12=→"CCD 12":T41)  [unwired: 12 in]
        n860 = call <vilib>:"Add State(s) to Queue__jki_lib_state_machine.vi"("State(s) in (\"\")"=w1774) -> ("States Out"=w1773:string)  [unwired: 14 in]
      }
      frame "newtdms" {
        # "Your code here.\n(You can make a copy of, or modify, this frame)"
        n861 = Unbundle By Name(w1867) -> ("Data Value Reference out"=w1855:refnum<k34>, "active cams"=w1850:string[])
        n862 = TDMS Close(8:w1865, 11:w1855) -> (0:w1849:errorcluster)  [unwired: 1 out]
        n863 = Get Date/Time In Seconds() -> (seconds since 1Jan1904=w1843:timestamp)
        n864 = call <vilib>:"Clear Errors.vi"("error in (no error)"=w1849) -> ("error out"=w1836:errorcluster)  [unwired: 5 in, 1 out]
        n865 = Format Date/Time String(time format string (%c)="%Y%m%d", seconds (now)=w1843) -> (date/time string=w1844:string)  [unwired: 1 in]
        n866 = Format Date/Time String(time format string (%c)="%Y%m%d%H%M", seconds (now)=w1843) -> (date/time string=w1841:string)  [unwired: 1 in]
        n867 = property on="new tdms" class="Bool (strict)"("Value"=FALSE ("new tdms")) -> ()  [unwired: 2 in, 2 out]
        n868 = Get Date/Time In Seconds() -> (seconds since 1Jan1904=w1864:timestamp)
        n869 = Format Date/Time String(time format string (%c)="%Y%m%d%H%M", seconds (now)=w1864) -> (date/time string=w1856:string)  [unwired: 1 in]
        n870 = Build Path(base path=w1837, name or relative path=w1844) -> (appended path=w1845:path)
        n871 = Concatenate Strings(w1856, "BeampointingBELLABTL_TRA.tdms" ("string")) -> (w1862:string)
        n872 = String To Path(string=w1862) -> ()  [unwired: 1 out]
        n873 = Concatenate Strings(w1841, "BeampointingBELLABTL_TRA.tdms" ("string")) -> (w1839:string)
        n874 = String To Path(string=w1839) -> (path=w1834:path)
        n875 = call <vilib>:"Check if File or Folder Exists.vi"("error in (no error)"=w1836, "path"=w1845) -> ("error out"=w1848:errorcluster, "file or folder exists?"=w1846:bool, "dup path"=w1847:path)  [unwired: 7 in]
        n876 = case shown="False" w1846 {
          tunnel: w1847 -> [w1873 w1875]
          tunnel: [w1872 w1875] -> w1833
          tunnel: w1848 -> [w1871 w1874]
          tunnel: [w1870 w1874] -> w1835
          frame False {
            n877 = Create Folder(path (use dialog)=w1873, error in=w1871) -> (created path=w1872:path, error out=w1870:errorcluster)  [unwired: 1 in, 1 out]
          }
          frame True {
          }
        }
        n878 = call <vilib>:"Add State(s) to Queue__jki_lib_state_machine.vi"("State(s) in (\"\")"=w1869) -> ("States Out"=w1868:string)  [unwired: 14 in]
        n879 = Build Path(base path=w1833, name or relative path=w1834) -> (appended path=w1857:path)
        n880 = TDMS Open(6:FALSE ("disable buffering (T)"), 7:enum16{"1.0", "2.0"}."2.0" ("file format version (2.0)"), 8:w1835, 10:T26."create or replace" ("operation"), 11:w1857) -> (0:w1853:errorcluster, 3:w1852:refnum<k34>)  [unwired: 2 in]
        n881 = call "TDMSbuffersize.vi"("error in (no error)"=w1853, "group names"=w1850, "Data Value Reference in"=w1852) -> ("error out"=w1832:errorcluster, "Data Value Reference out"=w1851:refnum<k34>)  [unwired: 7 in]
        n882 = Bundle By Name(cluster=w1867, "Data Value Reference out"=w1851) -> (w1866:T34)
        n883 = call <vilib>:"Clear Errors.vi"("error in (no error)"=w1832) -> ("error out"=w1831:errorcluster)  [unwired: 5 in, 1 out]
      }
      frame "Center" {
        # "Your code here.\n(You can make a copy of, or modify, this frame)"
        n884 = control-ref of="image::1"() -> (w1890:refnum<vi>)
        n885 = control-ref of="image::2"() -> (w1889:refnum<vi>)
        n886 = control-ref of="image::3"() -> (w1888:refnum<vi>)
        n887 = control-ref of="image::4"() -> (w1887:refnum<vi>)
        n888 = control-ref of="image::5"() -> (w1886:refnum<vi>)
        n889 = control-ref of="image::6"() -> (w1885:refnum<vi>)
        n890 = control-ref of="image::7"() -> (w1884:refnum<vi>)
        n891 = control-ref of="image::8"() -> (w1883:refnum<vi>)
        n892 = control-ref of="image::9"() -> (w1882:refnum<vi>)
        n893 = control-ref of="image::10"() -> (w1881:refnum<vi>)
        n894 = control-ref of="image::11"() -> (w1880:refnum<vi>)
        n895 = control-ref of="image::12"() -> (w1879:refnum<vi>)
        n896 = for {
          tunnel: [w1899] -> w1878 mode=indexing
          tunnel: w1877 -> [w1898] mode=indexing
          n897 = Unbundle By Name(w1898) -> ("Target.X::12"=w1897:refnum<vi>, "Target.Y::12"=w1896:refnum<vi>)
          n898 = property class="DigNum (strict)"(reference=w1897) -> ("Value"=w1900:dbl)  [unwired: 1 in, 2 out]
          n899 = property class="DigNum (strict)"(reference=w1896) -> ("Value"=w1901:dbl)  [unwired: 1 in, 2 out]
          n900 = Bundle("Value"=w1900, "Value"=w1901) -> (w1899:cluster{"Value":dbl, "Value":dbl})  [unwired: 1 in]
        }
        n901 = call <vilib>:"Add State(s) to Queue__jki_lib_state_machine.vi"("State(s) in (\"\")"=w1895) -> ("States Out"=w1894:string)  [unwired: 14 in]
        n902 = Build Array(w1890, w1889, w1888, w1887, w1886, w1885, w1884, w1883, w1882, w1881, w1880, w1879) -> (w1891:refnum<vi>[])
        n903 = for {
          tunnel: w1891 -> [w1903] mode=indexing
          tunnel: w1878 -> [w1902] mode=indexing
          n904 = property class="ImageControl"(reference=w1903, "Image Center Position"=w1902) -> ()  [unwired: 1 in, 2 out]
        }
        n905 = property on="Center" class="Bool (strict)"("Value"=FALSE ("Center")) -> ()  [unwired: 2 in, 2 out]
      }
      frame "ImgToAvg" {
        n906 = Decimal String To Number(string=w1913) -> (number=w1910:i32)  [unwired: 2 in, 1 out]
        n907 = Bundle By Name(cluster=w1912, "img to avg"=w1910) -> (w1911:T34)
        n908 = call <vilib>:"Build State String with Arguments__jki_lib_state_machine.vi"("Arguments (\"\")"="T" ("Arguments (\"\")"), "State"=" Device Ini") -> ("State with Arguments"=w1904:string)  [unwired: 4 in]
        n909 = call <vilib>:"Add State(s) to Queue__jki_lib_state_machine.vi"("State(s) in Front (\"\")"=w1904, "State(s) in (\"\")"=w1909) -> ("States Out"=w1908:string)  [unwired: 13 in]
      }
      frame "history" {
        # "Your code here.\n(You can make a copy of, or modify, this frame)"
        n910 = Unbundle By Name(w1923) -> ("Offset X"=w1929:dbl[][], "Offset Y"=w1928:dbl[][], "Mean Centroid X"=w1927:dbl[][], "Mean Centroid Y"=w1926:dbl[][], "Motor X"=w1925:dbl[][], "Motor Y"=w1924:dbl[][], "Time"=w1915:timestamp[][])
        n911 = for {
          tunnel: w1929 -> [w1947] mode=indexing
          tunnel: w1928 -> [w1945] mode=indexing
          tunnel: w1927 -> [w1944] mode=indexing
          tunnel: w1926 -> [w1943] mode=indexing
          tunnel: w1925 -> [w1942] mode=indexing
          tunnel: w1924 -> [w1941] mode=indexing
          tunnel: [w1946] -> w1921 mode=indexing
          tunnel: [w1940] -> w1920 mode=indexing
          tunnel: [w1936] -> w1919 mode=indexing
          tunnel: [w1939] -> w1918 mode=indexing
          tunnel: [w1938] -> w1917 mode=indexing
          tunnel: [w1937] -> w1916 mode=indexing
          tunnel: w1915 -> [w1935] mode=indexing
          tunnel: [w1933] -> w1914 mode=indexing
          w1934 = 0
          n912 = Delete From Array(array=w1942, index=w1934) -> (array with subset deleted=w1938:dbl[])  [unwired: 1 in, 1 out]
          n913 = Delete From Array(array=w1941, index=w1934) -> (array with subset deleted=w1937:dbl[])  [unwired: 1 in, 1 out]
          n914 = Delete From Array(array=w1935, index=w1934) -> (array with subset deleted=w1933:timestamp[])  [unwired: 1 in, 1 out]
          n915 = Delete From Array(array=w1944, index=w1934) -> (array with subset deleted=w1936:dbl[])  [unwired: 1 in, 1 out]
          n916 = Delete From Array(array=w1943, index=w1934) -> (array with subset deleted=w1939:dbl[])  [unwired: 1 in, 1 out]
          n917 = Delete From Array(array=w1945, index=w1934) -> (array with subset deleted=w1940:dbl[])  [unwired: 1 in, 1 out]
          n918 = Delete From Array(array=w1947, index=w1934) -> (array with subset deleted=w1946:dbl[])  [unwired: 1 in, 1 out]
        }
        n919 = call <vilib>:"Add State(s) to Queue__jki_lib_state_machine.vi"("State(s) in (\"\")"=w1932) -> ("States Out"=w1931:string)  [unwired: 14 in]
        n920 = Bundle By Name(cluster=w1923, "Offset X"=w1921, "Offset Y"=w1920, "Mean Centroid X"=w1919, "Mean Centroid Y"=w1918, "Motor X"=w1917, "Motor Y"=w1916, "Time"=w1914) -> (w1922:T34)
      }
    }
    n921 = property on="Box" class="Arr (strict)"() -> ("Value"=w64:T3)  [unwired: 2 in, 2 out]
    n922 = for {
      tunnel: w65 -> [w110]
      tunnel: w56 -> [w119]
      tunnel: w62 -> [w117] mode=indexing
      tunnel: w64 -> [w78] mode=indexing
      tunnel: w59 -> [w108]
      tunnel: w58 -> [w107]
      tunnel: w57 -> [w89]
      i -> [w88]
      w103 = T42 {"Draw"=TRUE, "Target"={"x"=20.0, "y"=20.0}, "Size"={"x"=20.0, "y"=20.0}, "Angle"=1250067.0, "Color"=1250067, "Thickness"=0, "CrosshairLabel"=""} ("Crosshair")
      w97 = T43 {"Left"=0, "Top"=0, "Right"=0, "Bottom"=0} ("Bounding Rectangle")
      n923 = call-poly <userlib>:"Filter 1D Array__ogtk.vi"("items to filter"=w117, "array"=w119) -> ("filtered item indices"=w120:i32[])  [unwired: 4 in, 1 out]
      n924 = Index Array(array=w120) -> (element=w109:i32)  [unwired: 1 in]
      n925 = Index Array(array=w89, index (row)=w88) -> (element=w86:dbl[])  [unwired: 1 in]
      n926 = Index Array(array=w108, index (row)=w88) -> (element=w96:dbl[])  [unwired: 1 in]
      n927 = Index Array(array=w107, index (row)=w88) -> (element=w94:dbl[])  [unwired: 1 in]
      n928 = Index Array(array=w110, index=w109) -> (element=w118:T20)
      n929 = Reverse 1D Array(array=w86) -> (reversed array=w85:dbl[])
      n930 = Unbundle By Name(w118) -> ("Target.X::12"=w122:refnum<vi>, "Target.Y::12"=w121:refnum<vi>)
      n931 = Reverse 1D Array(array=w96) -> (reversed array=w95:dbl[])
      n932 = Reverse 1D Array(array=w94) -> (reversed array=w93:dbl[])
      n933 = Index Array(array=w85) -> (element=w83:dbl)  [unwired: 1 in]
      n934 = Square Root(x=w83) -> (sqrt(x)=w82:dbl)
      n935 = Index Array(array=w93) -> (element=w90:dbl)  [unwired: 1 in]
      n936 = Index Array(array=w95) -> (element=w91:dbl)  [unwired: 1 in]
      n937 = Divide(x=w82, y=2.0) -> (x/y=w80:dbl)
      n938 = property class="DigNum (strict)"(reference=w122) -> ("Value"=w114:dbl)  [unwired: 1 in, 2 out]
      n939 = property class="DigNum (strict)"(reference=w121) -> ("Value"=w113:dbl)  [unwired: 1 in, 2 out]
      n940 = Bundle(cluster=cluster{"xhair size":dbl, "xhair size 2":dbl} {"xhair size"=25.0, "xhair size 2"=25.0} ("size"), "xhair size"=w80, "xhair size 2"=w80) -> (w84:cluster{"xhair size":dbl, "xhair size 2":dbl})
      n941 = Bundle By Name(cluster=w103, "Draw"=TRUE, "Target.x"=w114, "Target.y"=w113, "Size"=w84, "Color"=u32 16774656, "Angle"=0.0, "Thickness"=u8 1) -> (w116:T42)
      n942 = call "draw crosshair imaq.vi"("clear overlay"=TRUE, "Crosshair"=w116, "Bounding Rectangle"=w97, "image in"=w117) -> ("error out"=w100:errorcluster, "image out"=w99:T6)  [unwired: 6 in]
      n943 = Bundle By Name(cluster=w103, "Draw"=TRUE, "Target.x"=w91, "Target.y"=w90, "Size"=w84, "Color"=u32 8322834, "Angle"=0.0, "Thickness"=u8 1) -> (w101:T42)
      n944 = case shown="True" "average centroid" {
        tunnel: w101 -> [_ w127]
        tunnel: w100 -> [_ w132]
        tunnel: w99 -> [w124 w131]
        tunnel: w97 -> [_ w130]
        tunnel: w78 -> [w125 _]
        tunnel: [w123 w129] -> w77
        frame False {
          n945 = call "draw box imaq.vi"("Color"=u32 1244928, "Rectangle"=w125, "image in"=w124) -> ("error out"=w123:errorcluster)  [unwired: 7 in, 1 out]
        }
        frame True {
          n946 = call "draw crosshair imaq.vi"("clear overlay"=FALSE, "error in (no error)"=w132, "Crosshair"=w127, "Bounding Rectangle"=w130, "image in"=w131) -> ("error out"=w129:errorcluster)  [unwired: 5 in, 1 out]
        }
      }
      "error out 3" <- w77
    }
  }
  n947 = property on="Feedback Global" class="Bool (strict)"("Value"=FALSE ("Feedback Global")) -> ()  [unwired: 2 in, 2 out]
  n948 = Unbundle By Name(w25) -> ("Data Value Reference out"=w24:refnum<k34>)
  n949 = for {
    tunnel: w53 -> [w1950] mode=indexing
    tunnel: w52 -> [w1949]
    tunnel: [w1948] -> w23
    n950 = call "IMAQ Dispose"("Image"=w1950, "error in (no error)"=w1949) -> ("error out"=w1948:errorcluster)  [unwired: 4 in]
  }
  n951 = TDMS Close(8:w23, 11:w24) -> (0:→"error out 2":errorcluster)  [unwired: 1 out]
